vi "Main-final-V1.vi"() -> ()   [LabVIEW 2016]
uses:
  <vilib>/Platform/TimedLoop/XDataNode/timing_clust.ctl
  <vilib>/Platform/TimedLoop/XDataNode/nitl_modes.ctl
  <vilib>/Platform/TimedLoop/XDataNode/wakeup.ctl
  <vilib>/Modbus/subvis/Modbus API/Modbus API.lvclass/Modbus API.ctl
  <vilib>/Modbus/subvis/Transmission Data Unit (ADU)/Transmission Data Unit/Transmission Data Unit.lvclass/Transmission Data Unit.ctl
  <vilib>/Modbus/master/Data Access/Unit ID/Set Unit ID Property.vi
  <vilib>/Modbus/subvis/Transmission Data Unit (ADU)/Transmission Data Unit/Data Access/Unit ID/Write Unit ID.vi
  <vilib>/Modbus/subvis/Modbus API/Read Transmission Data Unit.vi
  <vilib>/Modbus/subvis/Modbus API/Write Transmission Data Unit.vi
  <vilib>/Modbus/master/Modbus Master.lvclass
  C:/Program Files (x86)/National Instruments/LabVIEW 2016/vi.lib/Modbus/subvis/Modbus API/Modbus API.lvclass
  <vilib>/Instr/_visa.llb/VISA Configure Serial Port (Instr).vi
  <vilib>/Modbus/master/Create Master Instance (TCP).vi
  <vilib>/httpClient/POSTBuffer.vi
  <vilib>/Modbus/subvis/Transmission Data Unit (ADU)/Transmission Data Unit/Transmission Data Unit.lvclass
  <vilib>/platform/TimedLoop/XDataNode/XDataNode.xnode
  <vilib>/httpClient/LabVIEWHTTPClient.lvlib
  <vilib>/Platform/TimedLoop/XDataNode/XDNodeRunTimeDep.lvlib
panel:
  out "logical OR 2":bool
  out "logical OR":bool
  out "x .or. y? 2":bool
  out "x .or. y?":bool
  in  "Tab Control 2":T1(tab)
  in  "Tab Control 4":enum32{"INVERTER 1", "INVERTER 2", "INVERTER 3"}(tab)
  in  "Tab Control 5":enum32{"DATA", "PLOTS"}(tab)
  out "AC-LOAD VOLTAGE":dbl
  out "AC-LOAD-CURRENT":dbl
  out "AC-LOAD-POWER":dbl
  out "AC-GRID-VOLTAGE":dbl
  out "AC-GRID-CURRENT":dbl
  out "AC-GRID-POWER":i32
  out "DC VOLT":dbl
  out "DC-CURRENT":dbl
  out "INVERT-DC-POWER":u32
  out "DC-POWER":dbl
  out "INVERT-DC-CURRENT":dbl
  out "CHARGE-DC-CURRENT":dbl
  out "CHARGE-DC-POWER":u32
  out "DC Power":cluster{dbl[], dbl[]}[](graph)
  out "DC Current":cluster{dbl[], dbl[]}[](graph)
  out "AC Power 1":cluster{dbl[], dbl[]}[](graph)
  out "AC Current 1":cluster{dbl[], dbl[]}[](graph)
  out "AC Voltage 1":cluster{dbl[], dbl[]}[](graph)
  in  "Tab Control 6":enum32{"DATA", "PLOTS"}(tab)
  out "AC-GRID-POWER 2":i32
  out "AC-GRID-CURRENT 2":dbl
  out "AC-GRID-VOLTAGE 2":dbl
  out "AC-LOAD-POWER 2":dbl
  out "AC-LOAD-CURRENT 2":dbl
  out "AC-LOAD VOLTAGE 2":dbl
  out "CHARGE-DC-POWER 2":u32
  out "CHARGE-DC-CURRENT 2":dbl
  out "INVERT-DC-CURRENT 2":dbl
  out "DC-POWER 2":dbl
  out "INVERT-DC-POWER 2":u32
  out "DC-CURRENT 2":dbl
  out "DC VOLT 2":dbl
  out "AC Voltage 2":cluster{dbl[], dbl[]}[](graph)
  out "AC Current 2":cluster{dbl[], dbl[]}[](graph)
  out "AC Power 2":cluster{dbl[], dbl[]}[](graph)
  out "DC Current 2":cluster{dbl[], dbl[]}[](graph)
  out "DC Power 2":cluster{dbl[], dbl[]}[](graph)
  in  "Tab Control 7":enum32{"DATA", "PLOTS"}(tab)
  out "CHARGE-DC-POWER 3":u32
  out "CHARGE-DC-CURRENT 3":dbl
  out "INVERT-DC-CURRENT 3":dbl
  out "DC-POWER 3":dbl
  out "INVERT-DC-POWER 3":u32
  out "DC-CURRENT 3":dbl
  out "DC VOLT 3":dbl
  out "AC-GRID-POWER 3":i32
  out "AC-GRID-CURRENT 3":dbl
  out "AC-GRID-VOLTAGE 3":dbl
  out "AC-LOAD-POWER 3":dbl
  out "AC-LOAD-CURRENT 3":dbl
  out "AC-LOAD VOLTAGE 3":dbl
  out "DC Power 3":cluster{dbl[], dbl[]}[](graph)
  out "DC Current 3":cluster{dbl[], dbl[]}[](graph)
  out "AC Power 3":cluster{dbl[], dbl[]}[](graph)
  out "AC Current 3":cluster{dbl[], dbl[]}[](graph)
  out "AC Voltage 3":cluster{dbl[], dbl[]}[](graph)
  in  "Tab Control 8":T2(tab)
  in  "Tab Control 9":enum32{"DATA", "PLOTS"}(tab)
  out "BATT FCAP-1":dbl(slide) scale=0.0..10.0
  out "BATT-CAP-1":dbl(slide) scale=0.0..100.0
  out "BATT-AVAIL-ENERGY-1":dbl(knob) scale=0.0..5200.0
  out "BATT-ENERGY-1":dbl(knob) scale=0.0..5200.0
  out "POWER-1":dbl(knob) scale=0.0..9000.0
  out "BATT-1 CURRENT":dbl(slide) scale=0.0..150.0
  out "batt-1 volt":u8(slide) scale=0.0..59.0
  out "BATTERY VOLTAGE 1":dbl
  out "BATTERY CURRENT":dbl
  out "BATTERY POWER":dbl
  out "BATTERY MAX ENERGY":dbl
  out "BATTERY AVAIL ENERGY":dbl
  out "BATTERY REM CAPACITY":dbl
  out "BATTERY FULL CAPACITY":dbl
  out "BATT-TEMP":dbl
  out "Batt-temp-1":dbl(slide) scale=0.0..100.0
  in  "Tab Control 11":enum32{"DATA", "PLOTS"}(tab)
  out "BATT FCAP-2":dbl(slide) scale=0.0..10.0
  out "BATT-CAP-2":dbl(slide) scale=0.0..100.0
  out "BATT-AVAIL-ENERGY-2":dbl(knob) scale=0.0..5200.0
  out "BATT-ENERGY-2":dbl(knob) scale=0.0..5200.0
  out "POWER-2":dbl(knob) scale=0.0..9000.0
  out "BATT-2 CURRENT":dbl(slide) scale=0.0..150.0
  out "batt-2 volt":u8(slide) scale=0.0..59.0
  out "BATTERY VOLTAGE 2":dbl
  out "BATTERY CURRENT 2":dbl
  out "BATTERY POWER 2":dbl
  out "BATTERY MAX ENERGY 2":dbl
  out "BATTERY AVAIL ENERGY 2":dbl
  out "BATTERY REM CAPACITY 2":dbl
  out "BATTERY FULL CAPACITY 2":dbl
  out "BATT-TEMP 2":dbl
  out "Batt-temp-2":dbl(slide) scale=0.0..100.0
  in  "Tab Control 12":enum32{"DATA", "PLOTS"}(tab)
  out "BATT FCAP-3":dbl(slide) scale=0.0..10.0
  out "BATT-CAP-3":dbl(slide) scale=0.0..100.0
  out "BATT-AVAIL-ENERGY-3":dbl(knob) scale=0.0..5200.0
  out "BATT-ENERGY-3":dbl(knob) scale=0.0..5200.0
  out "POWER-3":dbl(knob) scale=0.0..9000.0
  out "BATT-3 CURRENT":dbl(slide) scale=0.0..150.0
  out "batt-3 volt":u8(slide) scale=0.0..59.0
  out "BATTERY VOLTAGE 3":dbl
  out "BATTERY CURRENT 3":dbl
  out "BATTERY POWER 3":dbl
  out "BATTERY MAX ENERGY 3":dbl
  out "BATTERY AVAIL ENERGY 3":dbl
  out "BATTERY REM CAPACITY 3":dbl
  out "BATTERY FULL CAPACITY 3":dbl
  out "BATT-TEMP 3":dbl
  out "Batt-temp-3":dbl(slide) scale=0.0..100.0
  in  "Tab Control 13":enum32{"DATA", "PLOTS"}(tab)
  out "BATT FCAP-4":dbl(slide) scale=0.0..10.0
  out "BATT-CAP-4":dbl(slide) scale=0.0..100.0
  out "BATT-AVAIL-ENERGY-4":dbl(knob) scale=0.0..5200.0
  out "BATT-ENERGY-4":dbl(knob) scale=0.0..5200.0
  out "POWER-4":dbl(knob) scale=0.0..9000.0
  out "BATT-4 CURRENT":dbl(slide) scale=0.0..150.0
  out "batt-4 volt":u8(slide) scale=0.0..59.0
  out "BATTERY VOLTAGE 4":dbl
  out "BATTERY CURRENT 4":dbl
  out "BATTERY POWER 4":dbl
  out "BATTERY MAX ENERGY 4":dbl
  out "BATTERY AVAIL ENERGY 4":dbl
  out "BATTERY REM CAPACITY 4":dbl
  out "BATTERY FULL CAPACITY 4":dbl
  out "BATT-TEMP 4":dbl
  out "Batt-temp-4":dbl(slide) scale=0.0..100.0
  in  "Tab Control 14":enum32{"DATA", "PLOTS"}(tab)
  out "BATT FCAP-5":dbl(slide) scale=0.0..10.0
  out "BATT-CAP-5":dbl(slide) scale=0.0..100.0
  out "BATT-AVAIL-ENERGY-5":dbl(knob) scale=0.0..5200.0
  out "BATT-ENERGY-5":dbl(knob) scale=0.0..5200.0
  out "POWER-5":dbl(knob) scale=0.0..9000.0
  out "BATT-5 CURRENT":dbl(slide) scale=0.0..150.0
  out "batt-5 volt":u8(slide) scale=0.0..59.0
  out "BATTERY VOLTAGE 5":dbl
  out "BATTERY CURRENT 5":dbl
  out "BATTERY POWER 5":dbl
  out "BATTERY MAX ENERGY 5":dbl
  out "BATTERY AVAIL ENERGY 5":dbl
  out "BATTERY REM CAPACITY 5":dbl
  out "BATTERY FULL CAPACITY 5":dbl
  out "BATT-TEMP 5":dbl
  out "Batt-temp-5":dbl(slide) scale=0.0..100.0
  in  "?":T3(tab)
  out "Battery Voltage Discharge Plot":cluster{dbl[], dbl[]}[](graph)
  out "Battery Current Plot":cluster{dbl[], dbl[]}[](graph)
  out "Battery Power Plot":cluster{dbl[], dbl[]}[](graph)
  in  "?":T4(tab)
  out "Battery Remaining Capacity Plot":cluster{dbl[], dbl[]}[](graph)
  out "Battery Available Energy Plot":cluster{dbl[], dbl[]}[](graph)
  out "Battery temp plot":cluster{dbl[], dbl[]}[](graph)
  in  "Tab Control 10":enum32{"DATA", "PLOTS"}(tab)
  in  "?":enum32{"Voltage", "TAP Voltage", "Temperature"}(tab)
  out "Vertical Progress Bar 6":u8(slide) scale=0.0..100.0
  out "Vertical Progress Bar 5":u8(slide) scale=0.0..100.0
  out "Vertical Progress Bar 4":u8(slide) scale=0.0..100.0
  out "Vertical Progress Bar 3":u8(slide) scale=0.0..100.0
  out "Vertical Progress Bar 2":u8(slide) scale=0.0..100.0
  out "Vertical Progress Bar":u8(slide) scale=0.0..100.0
  out "?":u8(slide) scale=0.0..100.0
  out "VOLT-CAP-6":dbl
  out "VOLT-CAP-5":dbl
  out "VOLT-CAP-4":dbl
  out "VOLT-CAP-3":dbl
  out "VOLT-CAP-2":dbl
  out "VOLT-CAP-1":dbl
  out "MOD 6":bool
  out "MOD 5":bool
  out "TAP 7":dbl(slide) scale=0.0..100.0
  out "TAP 8":dbl(slide) scale=0.0..100.0
  out "TAP 9":dbl(slide) scale=0.0..100.0
  out "TAP 10":dbl(slide) scale=0.0..100.0
  out "TAP 11":dbl(slide) scale=0.0..100.0
  out "TAP 12":dbl(slide) scale=0.0..100.0
  out "TAP 13":dbl(slide) scale=0.0..100.0
  out "TAP 14":dbl(slide) scale=0.0..100.0
  out "TAP 15":dbl(slide) scale=0.0..100.0
  out "TAP 16":dbl(slide) scale=0.0..100.0
  out "TAP 17":dbl(slide) scale=0.0..100.0
  out "TAP 18":dbl(slide) scale=0.0..100.0
  out "MOD 4":bool
  out "TAP 19":dbl(slide) scale=0.0..100.0
  out "TAP 20":dbl(slide) scale=0.0..100.0
  out "TAP 4_":dbl(slide) scale=0.0..100.0
  out "TAP 4_3":dbl(slide) scale=0.0..100.0
  out "TAP 4_2":dbl(slide) scale=0.0..100.0
  out "TAP 4_1":dbl(slide) scale=0.0..100.0
  out "MOD 3":bool
  out "MOD 2":bool
  out "MOD 1":bool
  out "TAP 3_3":dbl(slide) scale=0.0..12.0
  out "TAP 3_1":dbl(slide) scale=0.0..5.0
  out "TAP 3_2":dbl(slide) scale=0.0..8.0
  out "TAP 3_6":dbl(slide) scale=0.0..25.0
  out "TAP 3_4":dbl(slide) scale=0.0..16.0
  out "TAP 3_5":dbl(slide) scale=0.0..20.0
  out "TAP 2_6":dbl(slide) scale=0.0..25.0
  out "TAP 2_5":dbl(slide) scale=0.0..20.0
  out "TAP 2_4":dbl(slide) scale=0.0..16.0
  out "TAP 2_3":dbl(slide) scale=0.0..12.0
  out "TAP 2_2":dbl(slide) scale=0.0..8.0
  out "TAP 2_1":dbl(slide) scale=0.0..5.0
  out "TAP 1_5":dbl(slide) scale=0.0..20.0
  out "TAP 1_4":dbl(slide) scale=0.0..16.0
  out "TAP 1_6":dbl(slide) scale=0.0..25.0
  out "TAP 1_3":dbl(slide) scale=0.0..12.0
  out "TAP 1_2":dbl(slide) scale=0.0..8.0
  out "TAP 1_1":dbl(slide) scale=0.0..5.0
  out "Temp_1":dbl(slide) scale=0.0..100.0
  out "Temp_2":dbl(slide) scale=0.0..100.0
  out "Temp_3":dbl(slide) scale=0.0..100.0
  out "Temp_4":dbl(slide) scale=0.0..100.0
  out "Temp_5":dbl(slide) scale=0.0..100.0
  out "Temp_6":dbl(slide) scale=0.0..100.0
  in  "Tab Control":T5(tab)
  out "TAP Voltages":cluster{dbl[], dbl[]}[](graph)
  out "Full Voltage":cluster{dbl[], dbl[]}[](graph)
  out "Module's Voltages":cluster{dbl[], dbl[]}[](graph)
  in  "BATT-GATE 2":bool
  in  "BATT-GATE 1":bool
  in  "BATT-GATE 5":bool
  in  "BATT-GATE 3":bool
  in  "BATT-GATE 4":bool
  in  "SUPERCAP-GATE 6":bool
  in  "Load-1":bool
  in  "Load-2":bool
  out "Power Button State":dbl
  out "Power Switch Led":bool
  in  "Tab Control 3":T6(tab)
  in  "INVERTER IP: 192.168.0.151":string
  in  "error in (no error)":errorcluster
  out "error out":errorcluster
  out "error out 2":errorcluster
  out "error out 3":errorcluster
  in  "VISA resource name":refnum<visa-resource-name>
  in  "Continuous Measurement":bool
  out "Total Received":u32
  out "Counter Register":dbl
  in  "Stop RT":bool
  in  "?":bool
  in  "Transmit Frame":T7={"timestamp high"=0, "timestamp low"=0, "identifier"=18, "type"=enum."Data Frame", "info A"=0, "info B"=0, "data length"=8, "data"=[0, 0, 0, 0, 0, 0, 0, 0]} {"identifier" format="%x"; "data" format="%.0x"}
  in  "control battery url":string
  in  "Batter data send url":string
  # "https://aertcsmartgrid.onrender.com/receive-data"
  # "https://aertcsmartgrid.onrender.com/get-btcontrol"
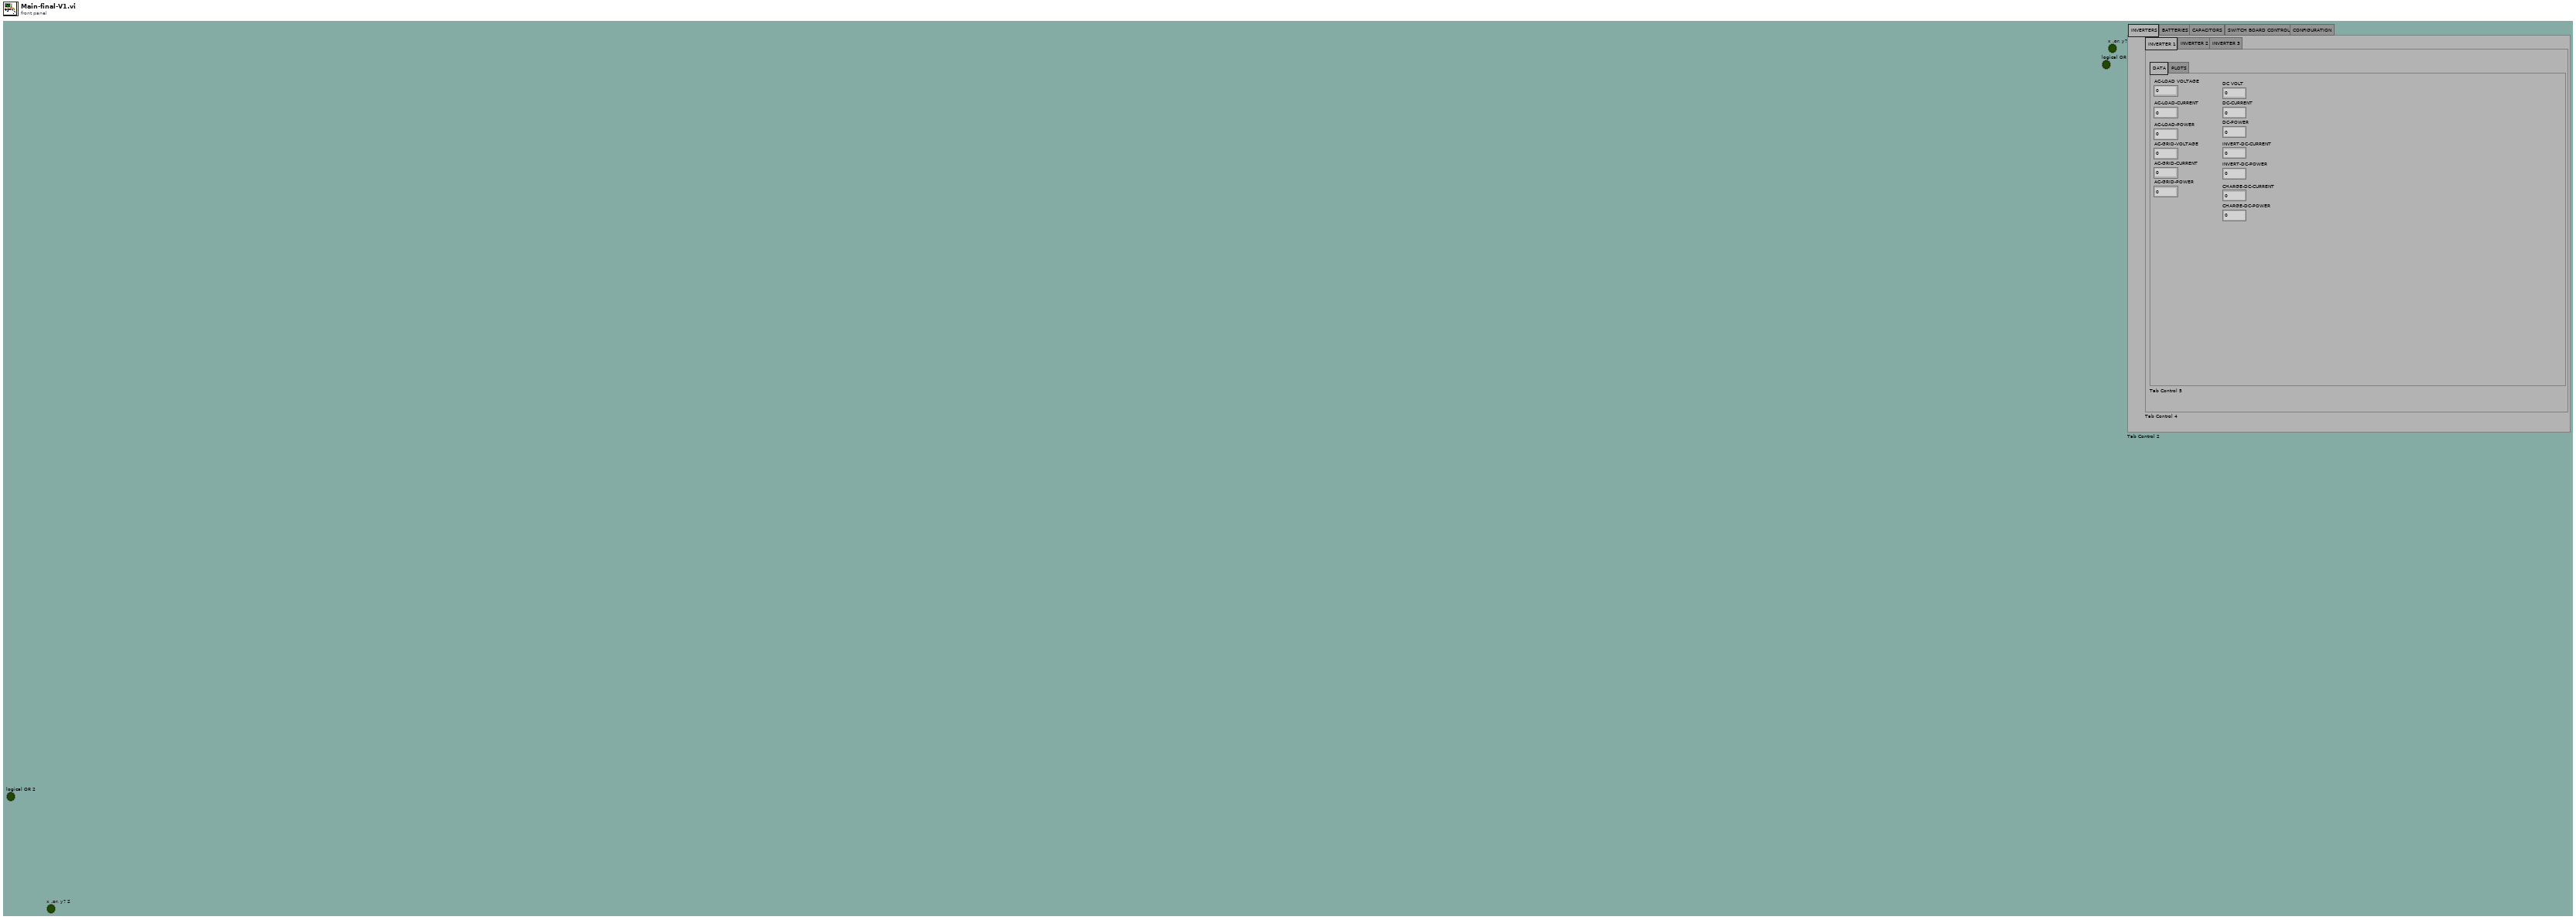
[diagram p1: front panel]
types:
  T1 = enum32{"INVERTERS", "BATTERIES", "CAPACITORS", "SWITCH BOARD CONTROL", "CONFIGURATION"}
  T2 = enum32{"BATTERY 1", "BATTERY 2", "BATTERY 3", "BATTERY 4", "BATTERY 5", "PLOTS"}
  T3 = enum32{"Voltage Plot", "Current Plot", "Power Plot"}
  T4 = enum32{"Remaining Capacity Plot", "Available Energy Plot", "Temperature Plot"}
  T5 = enum32{"TAP Plot", "FULL VOLTAGE PLOT", "FULL VOLTAGE PLOT 2"}
  T6 = enum32{"INVERTERS CONFIGURATION", "BATTERIES CONFIGURATION", "CAPACITORS CONFIGURATION", "WEBSITE CONFIGURATION"}
  T7 = cluster{"timestamp high":u32, "timestamp low":u32, "identifier":u32, "type":enum8{"Data Frame", "Remote Frame", "(reserved)", "(reserved) ", "(reserved)  ", "(reserved)   ", "Bus Error", "Transceiver Fault"}, "info A":u8, "info B":u8, "data length":u8, "data":u8[]}
  T8 = typedef "XDNodeRunTimeDep.lvlib/timing_clust.ctl" = cluster{"Expected End [f-1]":u64, "Actual End [f-1]":u64, "Finished Late? [f-1]":bool, "Expected End [i-1]":u64, "Actual End [i-1]":u64, "Finished Late? [i-1]":bool, "Expected Start [i]":u64, "Actual Start [i]":u64, "Expected Start [f]":u64, "Actual Start [f]":u64, "Source Name":string, "Structure Name":string, "Period":i64, "Deadline":i64, "Offset":i64, "Start":i64, "Priority":i32, "Timeout":i32, "Mode":T9, "Wakeup Reason":T10, "Error":errorcluster, "Source Type":string, "Secondary Source Type":string, "Global End Time":u64, "Global Start Time":u64, "Frame Duration":u64, "Iteration Duration":u64, "Assigned CPU":i32, "I/O Scan Engine Mode":u32}
  T9 = typedef "XDNodeRunTimeDep.lvlib/nitl_modes.ctl" = enum32{"No Change", "Process missed periods, maintain original phase", "Discard missed periods, maintain original phase", "Process missed periods, ignore original phase", "Discard missed periods, ignore original phase"}
  T10 = typedef "XDNodeRunTimeDep.lvlib/wakeup.ctl" = enum32{"Normal", "Aborted", "Asynchronous wakeup", "Timing source error", "Timed loop error", "Timeout"}
  T11 = typedef "LabVIEWHTTPClient.lvlib/ClientHandle.ctl" = refnum<k1>
  T12 = cluster{"unsigned byte array[0]":u8, "unsigned byte array[1]":u8, "unsigned byte array[2]":u8, "unsigned byte array[3]":u8, "unsigned byte array[4]":u8, "unsigned byte array[5]":u8, "unsigned byte array[6]":u8, "unsigned byte array[7]":u8, "unsigned byte array[8]":u8}
  T13 = cluster{"data[0]":u8, "data[1]":u8, "data[2]":u8, "data[3]":u8, "data[4]":u8, "data[5]":u8, "data[6]":u8, "data[7]":u8, "data[8]":u8}
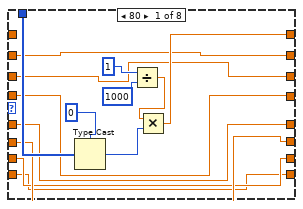
[diagram p3: hidden frame]
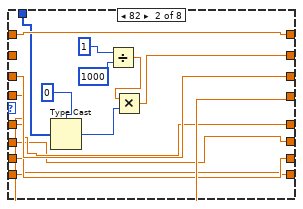
[diagram p4: hidden frame]
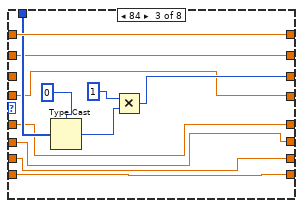
[diagram p5: hidden frame]
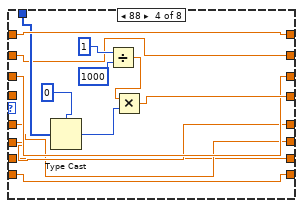
[diagram p6: hidden frame]
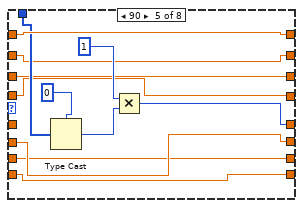
[diagram p7: hidden frame]
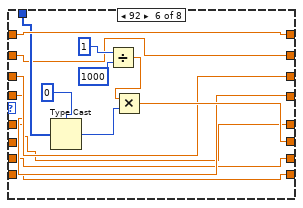
[diagram p8: hidden frame]
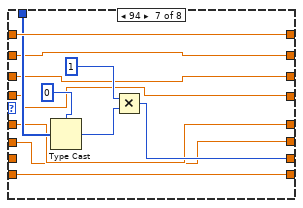
[diagram p9: hidden frame]
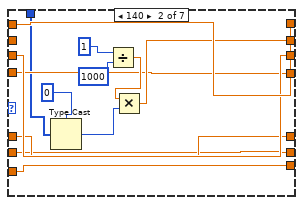
[diagram p10: hidden frame]
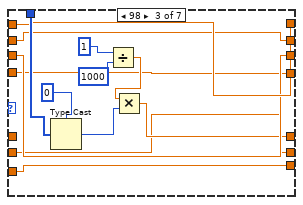
[diagram p11: hidden frame]
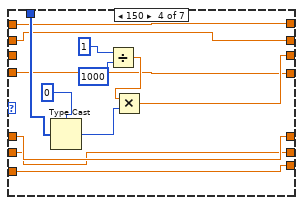
[diagram p12: hidden frame]
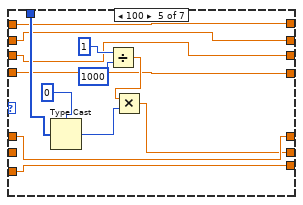
[diagram p13: hidden frame]
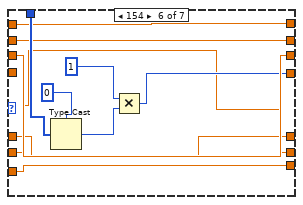
[diagram p14: hidden frame]
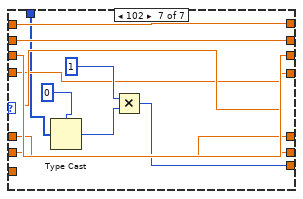
[diagram p15: hidden frame]
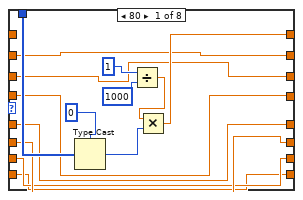
[diagram p16: hidden frame]
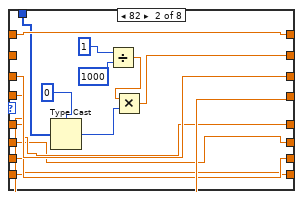
[diagram p17: hidden frame]
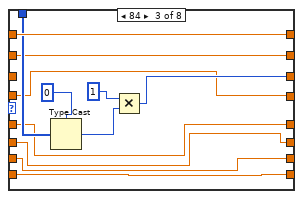
[diagram p18: hidden frame]
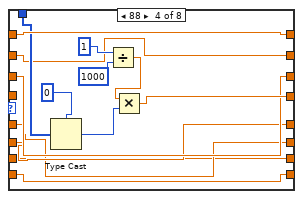
[diagram p19: hidden frame]
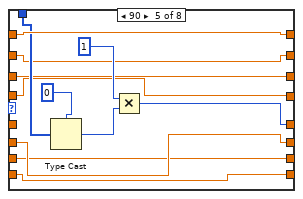
[diagram p20: hidden frame]
diagram:
  n1 = flat-sequence {
    tunnel: [w12] -> w6
    tunnel: [w11] -> w5
    tunnel: [w10] -> w4
    tunnel: [w9] -> w3
    tunnel: [w8] -> w2
    tunnel: [w7] -> w1
    tunnel: w6 -> [w137]
    tunnel: w5 -> [w136]
    tunnel: w4 -> [w125]
    tunnel: w3 -> [w124]
    tunnel: w2 -> [w123]
    tunnel: w1 -> [w122]
    frame #0 {
      n2 = call-poly "VISA Configure Serial Port"("VISA resource name"="VISA resource name", "timeout (10sec)"=u32 100000, "baud rate (9600)"=u32 115200) -> ("VISA resource name out"=w12:refnum<visa-resource-name>, "error out"=w11:errorcluster)  [unwired: 11 in]
      n3 = call <vilib>:"OpenHandle.vi"() -> ("client handle out"=w10:T11, "error out"=w9:errorcluster)  [unwired: 14 in]
      n4 = call <vilib>:"OpenHandle.vi"() -> ("client handle out"=w8:T11, "error out"=w7:errorcluster)  [unwired: 14 in]
    }
    frame #1 {
      w27 = 0.0
      w38 = 0.0
      w62 = 0.0
      w51 = 0.0
      w63 = 0.0
      w74 = 0.0
      w134 = 0.0
      w116 = 0.0
      w131 = 0.0
      w132 = 0.0
      w130 = 0.0
      w133 = 0.0
      w135 = 0.0
      w165 = 0.0
      # "M4"
      # "M3"
      # "M2"
      # "M1"
      n5 = disable-structure shown="Disabled" {
        frame Disabled {
          w171 = 0.005 ("y")
          w231 = 0.005 ("y")
          w244 = 0.005 ("y")
          n6 = Subtract() -> (y=w243:dbl, x-y=w253:dbl)  [unwired: 1 in]
          n7 = Subtract() -> (y=w242:dbl, x-y=w251:dbl)  [unwired: 1 in]
          n8 = Subtract() -> (x-y=w249:dbl)  [unwired: 2 in]
          n9 = Subtract() -> (x-y=w247:dbl)  [unwired: 2 in]
          n10 = Subtract() -> (x-y=w245:dbl)  [unwired: 2 in]
          n11 = Subtract(x=0.0, y=0.0) -> (x-y=w202:dbl)
          n12 = Subtract(x=0.0, y=0.0) -> (x-y=w186:dbl)
          n13 = Subtract(x=0.0, y=0.0) -> (x-y=w200:dbl)
          n14 = Subtract(x=0.0, y=0.0) -> (x-y=w198:dbl)
          n15 = Subtract(x=0.0, y=0.0) -> (x-y=w196:dbl)
          n16 = Subtract(x=0.0, y=0.0) -> (x-y=w194:dbl)
          n17 = Subtract(x=0.0, y=0.0) -> (x-y=w234:dbl)
          n18 = Subtract(x=0.0, y=0.0) -> (x-y=w232:dbl)
          n19 = Absolute Value(x=w253) -> (abs(x)=w254:dbl)
          n20 = Absolute Value(x=w251) -> (abs(x)=w252:dbl)
          n21 = Absolute Value(x=w249) -> (abs(x)=w250:dbl)
          n22 = Absolute Value(x=w247) -> (abs(x)=w248:dbl)
          n23 = Absolute Value(x=w245) -> (abs(x)=w246:dbl)
          n24 = Absolute Value(x=w202) -> (abs(x)=w203:dbl)
          n25 = Absolute Value(x=w186) -> (abs(x)=w187:dbl)
          n26 = Absolute Value(x=w200) -> (abs(x)=w201:dbl)
          n27 = Absolute Value(x=w198) -> (abs(x)=w199:dbl)
          n28 = Absolute Value(x=w196) -> (abs(x)=w197:dbl)
          n29 = Absolute Value(x=w194) -> (abs(x)=w195:dbl)
          n30 = Absolute Value(x=w234) -> (abs(x)=w235:dbl)
          n31 = Absolute Value(x=w232) -> (abs(x)=w233:dbl)
          n32 = Greater?(x=w254, y=w244) -> (0:w241:bool)
          n33 = Greater?(x=w252, y=w244) -> (0:w240:bool)
          n34 = Greater?(x=w250, y=w244) -> (0:w239:bool)
          n35 = Greater?(x=w248, y=w244) -> (0:w238:bool)
          n36 = Greater?(x=w246, y=w244) -> (0:w237:bool)
          n37 = call "BATT-ABSOLUTE-Second.vi"("B2"=0.0 ("y"), "Comp"=0.005 ("y"), "B1"=0.0 ("x"), "A2"=0.0 ("y"), "A1"=0.0 ("x")) -> ("Boolean"=→"x .or. y? 2":bool)  [unwired: 6 in]
          n38 = call "BATT-ABSOLUTE-Six.vi"("B2"=0.0 ("y"), "A6"=0.0 ("x"), "A3"=0.0 ("x"), "B6"=0.0 ("y"), "B3"=0.0 ("y"), "Comp"=0.005 ("y"), "A4"=0.0 ("x"), "B1"=0.0 ("y"), "B4"=0.0 ("y"), "A2"=0.0 ("x"), "A5"=0.0 ("x"), "A1"=0.0 ("x"), "B5"=0.0 ("y")) -> ("Boolean"=→"logical OR":bool)  [unwired: 6 in]
          n39 = Greater?(x=w203, y=w171) -> (0:w193:bool)
          n40 = Greater?(x=w187, y=w171) -> (0:w185:bool)
          n41 = Greater?(x=w201, y=w171) -> (0:w192:bool)
          n42 = Greater?(x=w199, y=w171) -> (0:w191:bool)
          n43 = Greater?(x=w197, y=w171) -> (0:w190:bool)
          n44 = Greater?(x=w195, y=w171) -> (0:w189:bool)
          n45 = Greater?(x=w235, y=w231) -> (0:w230:bool)
          n46 = Greater?(x=w233, y=w231) -> (0:w229:bool)
          n47 = Build Array(w241, w240, w239, w238, w237) -> (w236:bool[])
          n48 = Or(x=w230, y=w229) -> (x .or. y?=→"x .or. y?":bool)
          n49 = Build Array(w185, w193, w192, w191, w190, w189) -> (w188:bool[])
          n50 = Or Array Elements(Boolean array=w236) -> ()  [unwired: 1 out]
          n51 = Or Array Elements(Boolean array=w188) -> (logical OR=→"logical OR 2":bool)
        }
        frame Enabled {
        }
      }
      n52 = call-poly <vilib>:"Create Master Instance.vi"("error in (no error)"="error in (no error)", "port (502)"=u16 503, "address"="INVERTER IP: 192.168.0.151") -> ("error out"=w85:errorcluster, "TCP master instance"=w88:refnum<class "Modbus Master.lvclass">)  [unwired: 7 in]
      n53 = while {
        shift-right: [w595] -> w87
        shift-left: w88 -> [w504]
        shift-right: [w594] -> w84
        shift-left: w85 -> [w503]
        shift-right: [w587] -> _
        shift-left: w74 -> [w588]
        shift-right: [w494] -> _
        shift-left: w74 -> [w495]
        shift-right: [w490] -> _
        shift-left: w74 -> [w491]
        shift-right: [w486] -> _
        shift-left: w74 -> [w487]
        shift-right: [w397] -> _
        shift-left: dbl[] [] -> [w586]
        shift-right: [w395] -> _
        shift-left: dbl[] [] -> [w585]
        shift-right: [w393] -> _
        shift-left: dbl[] [] -> [w584]
        shift-right: [w492] -> _
        shift-left: w74 -> [w493]
        shift-right: [w488] -> _
        shift-left: w74 -> [w489]
        shift-right: [w484] -> _
        shift-left: w74 -> [w485]
        shift-right: [w391] -> _
        shift-left: dbl[] [] -> [w581]
        shift-right: [w389] -> _
        shift-left: dbl[] [] -> [w582]
        shift-right: [w387] -> _
        shift-left: dbl[] [] -> [w583]
        shift-right: [w429] -> _
        shift-left: dbl[] [] -> [w574]
        shift-right: [w428] -> _
        shift-left: dbl[] [] -> [w575]
        shift-right: [w427] -> _
        shift-left: dbl[] [] -> [w576]
        shift-right: [w369] -> _
        shift-left: dbl[] [] -> [w577]
        shift-right: [w367] -> _
        shift-left: dbl[] [] -> [w578]
        shift-right: [w365] -> _
        shift-left: dbl[] [] -> [w580]
        shift-right: [w363] -> _
        shift-left: dbl[] [] -> [w579]
        shift-right: [w573] -> _
        shift-left: w63 -> [w572]
        shift-right: [w568] -> _
        shift-left: w63 -> [w570]
        shift-right: [w567] -> _
        shift-left: w63 -> [w569]
        shift-right: [w450] -> _
        shift-left: w63 -> [w453]
        shift-right: [w449] -> _
        shift-left: w63 -> [w446]
        shift-right: [w448] -> _
        shift-left: w63 -> [w452]
        shift-right: [w447] -> _
        shift-left: w63 -> [w565]
        shift-right: [w566] -> _
        shift-left: w63 -> [w451]
        shift-right: [w536] -> w45
        shift-left: _ -> [_]
        shift-right: [w537] -> w46
        shift-left: _ -> [_]
        shift-right: [w542] -> _
        shift-left: w51 -> [w541]
        shift-right: [w482] -> _
        shift-left: w51 -> [w483]
        shift-right: [w478] -> _
        shift-left: w51 -> [w479]
        shift-right: [w474] -> _
        shift-left: w51 -> [w475]
        shift-right: [w339] -> _
        shift-left: dbl[] [] -> [w543]
        shift-right: [w337] -> _
        shift-left: dbl[] [] -> [w544]
        shift-right: [w335] -> _
        shift-left: dbl[] [] -> [w545]
        shift-right: [w480] -> _
        shift-left: w51 -> [w481]
        shift-right: [w476] -> _
        shift-left: w51 -> [w477]
        shift-right: [w472] -> _
        shift-left: w51 -> [w473]
        shift-right: [w329] -> _
        shift-left: dbl[] [] -> [w548]
        shift-right: [w331] -> _
        shift-left: dbl[] [] -> [w547]
        shift-right: [w333] -> _
        shift-left: dbl[] [] -> [w546]
        shift-right: [w424] -> _
        shift-left: dbl[] [] -> [w555]
        shift-right: [w423] -> _
        shift-left: dbl[] [] -> [w554]
        shift-right: [w422] -> _
        shift-left: dbl[] [] -> [w553]
        shift-right: [w313] -> _
        shift-left: dbl[] [] -> [w552]
        shift-right: [w311] -> _
        shift-left: dbl[] [] -> [w551]
        shift-right: [w309] -> _
        shift-left: dbl[] [] -> [w549]
        shift-right: [w307] -> _
        shift-left: dbl[] [] -> [w550]
        shift-right: [w556] -> _
        shift-left: w62 -> [w557]
        shift-right: [w561] -> _
        shift-left: w62 -> [w559]
        shift-right: [w562] -> _
        shift-left: w62 -> [w560]
        shift-right: [w441] -> _
        shift-left: w62 -> [w445]
        shift-right: [w440] -> _
        shift-left: w62 -> [w444]
        shift-right: [w439] -> _
        shift-left: w62 -> [w443]
        shift-right: [w438] -> _
        shift-left: w62 -> [w442]
        shift-right: [w563] -> _
        shift-left: w62 -> [w564]
        shift-right: [w533] -> w44
        shift-left: _ -> [_]
        shift-right: [w532] -> w43
        shift-left: _ -> [_]
        shift-right: [w527] -> _
        shift-left: w38 -> [w528]
        shift-right: [w465] -> _
        shift-left: w38 -> [w471]
        shift-right: [w464] -> _
        shift-left: w38 -> [w470]
        shift-right: [w463] -> _
        shift-left: w38 -> [w469]
        shift-right: [w287] -> _
        shift-left: dbl[] [] -> [w526]
        shift-right: [w285] -> _
        shift-left: dbl[] [] -> [w525]
        shift-right: [w283] -> _
        shift-left: dbl[] [] -> [w524]
        shift-right: [w462] -> _
        shift-left: w38 -> [w468]
        shift-right: [w461] -> _
        shift-left: w38 -> [w467]
        shift-right: [w460] -> _
        shift-left: w38 -> [w466]
        shift-right: [w281] -> _
        shift-left: dbl[] [] -> [w521]
        shift-right: [w279] -> _
        shift-left: dbl[] [] -> [w522]
        shift-right: [w277] -> _
        shift-left: dbl[] [] -> [w523]
        shift-right: [w419] -> _
        shift-left: dbl[] [] -> [w514]
        shift-right: [w418] -> _
        shift-left: dbl[] [] -> [w515]
        shift-right: [w417] -> _
        shift-left: dbl[] [] -> [w516]
        shift-right: [w261] -> _
        shift-left: dbl[] [] -> [w517]
        shift-right: [w259] -> _
        shift-left: dbl[] [] -> [w518]
        shift-right: [w257] -> _
        shift-left: dbl[] [] -> [w520]
        shift-right: [w255] -> _
        shift-left: dbl[] [] -> [w519]
        shift-right: [w513] -> _
        shift-left: w27 -> [w512]
        shift-right: [w508] -> _
        shift-left: w27 -> [w510]
        shift-right: [w507] -> _
        shift-left: w27 -> [w509]
        shift-right: [w433] -> _
        shift-left: w27 -> [w437]
        shift-right: [w432] -> _
        shift-left: w27 -> [w436]
        shift-right: [w431] -> _
        shift-left: w27 -> [w435]
        shift-right: [w430] -> _
        shift-left: w27 -> [w434]
        shift-right: [w506] -> _
        shift-left: w27 -> [w505]
        shift-right: [w399] -> _
        shift-left: dbl[] [] -> [w409]
        shift-right: [w371] -> _
        shift-left: dbl[] [] -> [w380]
        shift-right: [w341] -> _
        shift-left: dbl[] [] -> [w352]
        shift-right: [w315] -> _
        shift-left: dbl[] [] -> [w328]
        shift-right: [w289] -> _
        shift-left: dbl[] [] -> [w306]
        shift-right: [w263] -> _
        shift-left: dbl[] [] -> [w276]
        stop <- FALSE stop-if-true
        n54 = call "UP-COUNTER-V1.vi"("UPPER LIMIT"=17.0) -> ("COUNT"=w589:dbl)  [unwired: 10 in]
        n55 = case shown="1, Default" w589 {
          tunnel: [u32 86 u32 140 u32 98 u32 150 u32 100 u32 154 u32 102 u32 80 u32 82 u32 84 u32 88 u32 90 u32 92 u32 94 u32 96] -> w502
          frame 1, Default {
            # "TEMP-BATT"
          }
          frame 2 {
            # "AC-LOAD-VOLT"
          }
          frame 3 {
            # "AC-GRID-VOLT"
          }
          frame 4 {
            # "AC-LOAD-CURRENT"
          }
          frame 5 {
            # "AC-GRID-CURRENT"
          }
          frame 6 {
            # "AC-LOAD-POWER"
          }
          frame 7 {
            # "AC-GRID-POWER"
          }
          frame 8 {
            # "DC-VOLT"
          }
          frame 9 {
            # "DC-CURRENT"
          }
          frame 10 {
            # "DC-POWER"
          }
          frame 11 {
            # "INVERT-DC-CURRENT"
          }
          frame 12 {
            # "INVERT-DC-POWER"
          }
          frame 13 {
            # "CHARGE-DC-CURRENT"
          }
          frame 14 {
            # "CHARGE-DC-POWER"
          }
          frame 15 {
            # "CHARGE-%"
          }
        }
        n56 = property class="Modbus Master"(reference=w504, error in=w503, "Data Access:Unit ID"=u8 12 ("Unit ID")) -> (reference out=w529:refnum<class "Modbus Master.lvclass">, error out=w530:errorcluster)
        n57 = property class="Modbus Master"(reference=w504, error in=w503, "Data Access:Unit ID"=u8 10 ("Unit ID")) -> (reference out=w590:refnum<class "Modbus Master.lvclass">, error out=w591:errorcluster)
        n58 = property class="Modbus Master"(reference=w504, error in=w503, "Data Access:Unit ID"=u8 11 ("Unit ID")) -> (reference out=w540:refnum<class "Modbus Master.lvclass">, error out=w539:errorcluster)
        n59 = call-dynamic "Read Holding Registers.vi"("error in (no error)"=w530, "number of holding registers"=u32 2, "starting address"=w502, "Modbus master in"=w529) -> ("error out"=w532:errorcluster, "register values"=w511:u16[], "Modbus master out"=w533:refnum<class "Modbus Master.lvclass">)  [unwired: 5 in]
        n60 = call-dynamic "Read Holding Registers.vi"("error in (no error)"=w591, "number of holding registers"=u32 2, "starting address"=w502, "Modbus master in"=w590) -> ("error out"=w594:errorcluster, "register values"=w571:u16[], "Modbus master out"=w595:refnum<class "Modbus Master.lvclass">)  [unwired: 5 in]
        n61 = call-dynamic "Read Holding Registers.vi"("error in (no error)"=w539, "number of holding registers"=u32 2, "starting address"=w502, "Modbus master in"=w540) -> ("error out"=w537:errorcluster, "register values"=w558:u16[], "Modbus master out"=w536:refnum<class "Modbus Master.lvclass">)  [unwired: 5 in]
        n62 = case shown="86, Default" w502 {
          tunnel: w511 -> [w701 w716 w736 w749 w762 w776 w779]
          tunnel: [w710 w723 w735 w748 w761 w775 w787] -> w527
          tunnel: w528 -> [_ w723 w735 w748 w761 w775 w787]
          tunnel: [w707 w722 w731 w747 w760 w774 w786] -> w465
          tunnel: w471 -> [w707 _ w731 w747 w760 w774 w786]
          tunnel: [w706 w721 w734 w746 w757 w773 w785] -> w464
          tunnel: w470 -> [w706 w721 w734 _ w757 w773 w785]
          tunnel: [w705 w720 w733 w745 w759 w772 w780] -> w463
          tunnel: w469 -> [w705 w720 w733 w745 w759 _ w780]
          tunnel: [w704 w719 w732 w744 w758 w770 w783] -> w462
          tunnel: w468 -> [w704 w719 _ w744 w758 w770 w783]
          tunnel: [w703 w718 w730 w743 w756 w769 w782] -> w461
          tunnel: w467 -> [w703 w718 w730 w743 _ w769 w782]
          tunnel: [w702 w717 w729 w742 w755 w768 w781] -> w460
          tunnel: w466 -> [w702 w717 w729 w742 w755 w768 _]
          frame 86, Default {
            n63 = Type Cast(type=u16 0, x=w701) -> (*(type *) &x=w709:u16)
            n64 = Divide(x=u32 1, y=u32 100) -> (x/y=w712:dbl)
            n65 = Multiply(x=w712, y=w709) -> (x*y=w711:dbl)
            n66 = Subtract(x=w711, y=273) -> (x-y=w710:dbl)
          }
          frame 140 {
            n67 = Type Cast(type=u32 0, x=w716) -> (*(type *) &x=w725:u32)
            n68 = Divide(x=u32 1, y=u32 1000) -> (x/y=w726:dbl)
            n69 = Multiply(x=w726, y=w725) -> (x*y=w722:dbl)
          }
          frame 98 {
            n70 = Type Cast(type=u32 0, x=w736) -> (*(type *) &x=w738:u32)
            n71 = Divide(x=u32 1, y=u32 1000) -> (x/y=w739:dbl)
            n72 = Multiply(x=w739, y=w738) -> (x*y=w732:dbl)
          }
          frame 150 {
            n73 = Type Cast(type=0, x=w749) -> (*(type *) &x=w751:i32)
            n74 = Divide(x=u32 1, y=u32 1000) -> (x/y=w752:dbl)
            n75 = Multiply(x=w752, y=w751) -> (x*y=w746:dbl)
          }
          frame 100 {
            n76 = Type Cast(type=0, x=w762) -> (*(type *) &x=w764:i32)
            n77 = Divide(x=u32 1, y=u32 1000) -> (x/y=w765:dbl)
            n78 = Multiply(x=w765, y=w764) -> (x*y=w756:dbl)
          }
          frame 154 {
            n79 = Type Cast(type=0, x=w776) -> (*(type *) &x=w778:i32)
            n80 = Multiply(x=1, y=w778) -> (x*y=w772:i32)
          }
          frame 102 {
            n81 = Type Cast(type=0, x=w779) -> (*(type *) &x=w789:i32)
            n82 = Multiply(x=1, y=w789) -> (x*y=w781:i32)
          }
        }
        "AC-LOAD VOLTAGE 3" <- w465
        "AC-LOAD-CURRENT 3" <- w464
        "AC-LOAD-POWER 3" <- w463
        "AC-GRID-VOLTAGE 3" <- w462
        "AC-GRID-CURRENT 3" <- w461
        "AC-GRID-POWER 3" <- w460
        n83 = case shown="98" w502 {
          tunnel: w571 -> [w1102 w1117 w1137 w1150 w1163 w1177 w1180]
          tunnel: [w1111 w1124 w1136 w1149 w1162 w1176 w1188] -> w587
          tunnel: w588 -> [_ w1124 w1136 w1149 w1162 w1176 w1188]
          tunnel: [w1108 w1123 w1132 w1148 w1161 w1175 w1187] -> w494
          tunnel: w495 -> [w1108 _ w1132 w1148 w1161 w1175 w1187]
          tunnel: [w1107 w1122 w1135 w1147 w1158 w1174 w1186] -> w490
          tunnel: w491 -> [w1107 w1122 w1135 _ w1158 w1174 w1186]
          tunnel: [w1106 w1121 w1134 w1146 w1160 w1173 w1181] -> w486
          tunnel: w487 -> [w1106 w1121 w1134 w1146 w1160 _ w1181]
          tunnel: [w1105 w1120 w1133 w1145 w1159 w1171 w1184] -> w492
          tunnel: w493 -> [w1105 w1120 _ w1145 w1159 w1171 w1184]
          tunnel: [w1104 w1119 w1131 w1144 w1157 w1170 w1183] -> w488
          tunnel: w489 -> [w1104 w1119 w1131 w1144 _ w1170 w1183]
          tunnel: [w1103 w1118 w1130 w1143 w1156 w1169 w1182] -> w484
          tunnel: w485 -> [w1103 w1118 w1130 w1143 w1156 w1169 _]
          frame 86, Default {
            n84 = Type Cast(type=u16 0, x=w1102) -> (*(type *) &x=w1110:u16)
            n85 = Divide(x=u32 1, y=u32 100) -> (x/y=w1113:dbl)
            n86 = Multiply(x=w1113, y=w1110) -> (x*y=w1112:dbl)
            n87 = Subtract(x=w1112, y=273) -> (x-y=w1111:dbl)
          }
          frame 140 {
            n88 = Type Cast(type=u32 0, x=w1117) -> (*(type *) &x=w1126:u32)
            n89 = Divide(x=u32 1, y=u32 1000) -> (x/y=w1127:dbl)
            n90 = Multiply(x=w1127, y=w1126) -> (x*y=w1123:dbl)
          }
          frame 98 {
            n91 = Type Cast(type=u32 0, x=w1137) -> (*(type *) &x=w1139:u32)
            n92 = Divide(x=u32 1, y=u32 1000) -> (x/y=w1140:dbl)
            n93 = Multiply(x=w1140, y=w1139) -> (x*y=w1133:dbl)
          }
          frame 150 {
            n94 = Type Cast(type=0, x=w1150) -> (*(type *) &x=w1152:i32)
            n95 = Divide(x=u32 1, y=u32 1000) -> (x/y=w1153:dbl)
            n96 = Multiply(x=w1153, y=w1152) -> (x*y=w1147:dbl)
          }
          frame 100 {
            n97 = Type Cast(type=0, x=w1163) -> (*(type *) &x=w1165:i32)
            n98 = Divide(x=u32 1, y=u32 1000) -> (x/y=w1166:dbl)
            n99 = Multiply(x=w1166, y=w1165) -> (x*y=w1157:dbl)
          }
          frame 154 {
            n100 = Type Cast(type=0, x=w1177) -> (*(type *) &x=w1179:i32)
            n101 = Multiply(x=1, y=w1179) -> (x*y=w1173:i32)
          }
          frame 102 {
            n102 = Type Cast(type=0, x=w1180) -> (*(type *) &x=w1190:i32)
            n103 = Multiply(x=1, y=w1190) -> (x*y=w1182:i32)
          }
        }
        "AC-LOAD VOLTAGE" <- w494
        "AC-LOAD-CURRENT" <- w490
        "AC-LOAD-POWER" <- w486
        "AC-GRID-VOLTAGE" <- w492
        "AC-GRID-CURRENT" <- w488
        "AC-GRID-POWER" <- w484
        n104 = case shown="86, Default" w502 {
          tunnel: w558 -> [w894 w909 w929 w942 w955 w969 w972]
          tunnel: [w903 w916 w928 w941 w954 w968 w980] -> w542
          tunnel: w541 -> [_ w916 w928 w941 w954 w968 w980]
          tunnel: [w900 w915 w924 w940 w953 w967 w979] -> w482
          tunnel: w483 -> [w900 _ w924 w940 w953 w967 w979]
          tunnel: [w899 w914 w927 w939 w950 w966 w978] -> w478
          tunnel: w479 -> [w899 w914 w927 _ w950 w966 w978]
          tunnel: [w898 w913 w926 w938 w952 w965 w973] -> w474
          tunnel: w475 -> [w898 w913 w926 w938 w952 _ w973]
          tunnel: [w897 w912 w925 w937 w951 w963 w976] -> w480
          tunnel: w481 -> [w897 w912 _ w937 w951 w963 w976]
          tunnel: [w896 w911 w923 w936 w949 w962 w975] -> w476
          tunnel: w477 -> [w896 w911 w923 w936 _ w962 w975]
          tunnel: [w895 w910 w922 w935 w948 w961 w974] -> w472
          tunnel: w473 -> [w895 w910 w922 w935 w948 w961 _]
          frame 86, Default {
            n105 = Type Cast(type=u16 0, x=w894) -> (*(type *) &x=w902:u16)
            n106 = Divide(x=u32 1, y=u32 100) -> (x/y=w905:dbl)
            n107 = Multiply(x=w905, y=w902) -> (x*y=w904:dbl)
            n108 = Subtract(x=w904, y=273) -> (x-y=w903:dbl)
          }
          frame 140 {
            n109 = Type Cast(type=u32 0, x=w909) -> (*(type *) &x=w918:u32)
            n110 = Divide(x=u32 1, y=u32 1000) -> (x/y=w919:dbl)
            n111 = Multiply(x=w919, y=w918) -> (x*y=w915:dbl)
          }
          frame 98 {
            n112 = Type Cast(type=u32 0, x=w929) -> (*(type *) &x=w931:u32)
            n113 = Divide(x=u32 1, y=u32 1000) -> (x/y=w932:dbl)
            n114 = Multiply(x=w932, y=w931) -> (x*y=w925:dbl)
          }
          frame 150 {
            n115 = Type Cast(type=0, x=w942) -> (*(type *) &x=w944:i32)
            n116 = Divide(x=u32 1, y=u32 1000) -> (x/y=w945:dbl)
            n117 = Multiply(x=w945, y=w944) -> (x*y=w939:dbl)
          }
          frame 100 {
            n118 = Type Cast(type=0, x=w955) -> (*(type *) &x=w957:i32)
            n119 = Divide(x=u32 1, y=u32 1000) -> (x/y=w958:dbl)
            n120 = Multiply(x=w958, y=w957) -> (x*y=w949:dbl)
          }
          frame 154 {
            n121 = Type Cast(type=0, x=w969) -> (*(type *) &x=w971:i32)
            n122 = Multiply(x=1, y=w971) -> (x*y=w965:i32)
          }
          frame 102 {
            n123 = Type Cast(type=0, x=w972) -> (*(type *) &x=w982:i32)
            n124 = Multiply(x=1, y=w982) -> (x*y=w974:i32)
          }
        }
        "AC-LOAD VOLTAGE 2" <- w482
        "AC-LOAD-CURRENT 2" <- w478
        "AC-LOAD-POWER 2" <- w474
        "AC-GRID-VOLTAGE 2" <- w480
        "AC-GRID-CURRENT 2" <- w476
        "AC-GRID-POWER 2" <- w472
        n125 = case shown="96, Default" w502 {
          tunnel: [w603 w619 w630 w642 w656 w668 w682 w694] -> w508
          tunnel: [w602 w616 w634 w641 w655 w667 w681 w693] -> w507
          tunnel: [w600 w614 w628 w640 w660 w665 w679 w691] -> w432
          tunnel: [w598 w612 w626 w638 w652 w664 w686 w689] -> w430
          tunnel: [w601 w615 w629 w645 w654 w666 w680 w692] -> w433
          tunnel: [w599 w613 w627 w639 w653 w671 w678 w690] -> w431
          tunnel: [w597 w611 w625 w637 w651 w663 w677 w697] -> w506
          tunnel: [w605 w618 w632 w644 w658 w670 w684 w696] -> w513
          tunnel: w512 -> [_ w618 w632 w644 w658 w670 w684 w696]
          tunnel: w511 -> [w604 w617 w631 w643 w657 w669 w683 w695]
          tunnel: w510 -> [w603 _ w630 w642 w656 w668 w682 w694]
          tunnel: w509 -> [w602 w616 _ w641 w655 w667 w681 w693]
          tunnel: w437 -> [w601 w615 w629 _ w654 w666 w680 w692]
          tunnel: w436 -> [w600 w614 w628 w640 _ w665 w679 w691]
          tunnel: w435 -> [w599 w613 w627 w639 w653 _ w678 w690]
          tunnel: w434 -> [w598 w612 w626 w638 w652 w664 _ w689]
          tunnel: w505 -> [w597 w611 w625 w637 w651 w663 w677 _]
          frame 80 {
            n126 = Type Cast(type=u32 0, x=w604) -> (*(type *) &x=w608:u32)
            n127 = Divide(x=u32 1, y=u32 1000) -> (x/y=w609:dbl)
            n128 = Multiply(x=w609, y=w608) -> (x*y=w605:dbl)
          }
          frame 82 {
            n129 = Type Cast(type=0, x=w617) -> (*(type *) &x=w621:i32)
            n130 = Divide(x=u32 1, y=u32 1000) -> (x/y=w622:dbl)
            n131 = Multiply(x=w622, y=w621) -> (x*y=w619:dbl)
          }
          frame 84 {
            n132 = Type Cast(type=0, x=w631) -> (*(type *) &x=w636:i32)
            n133 = Multiply(x=u32 1, y=w636) -> (x*y=w634:u32)
          }
          frame 88 {
            n134 = Type Cast(type=u32 0, x=w643) -> (*(type *) &x=w647:u32)
            n135 = Divide(x=u32 1, y=u32 1000) -> (x/y=w648:dbl)
            n136 = Multiply(x=w648, y=w647) -> (x*y=w645:dbl)
          }
          frame 90 {
            n137 = Type Cast(type=u32 0, x=w657) -> (*(type *) &x=w662:u32)
            n138 = Multiply(x=u32 1, y=w662) -> (x*y=w660:u32)
          }
          frame 92 {
            n139 = Type Cast(type=u32 0, x=w669) -> (*(type *) &x=w673:u32)
            n140 = Divide(x=u32 1, y=u32 1000) -> (x/y=w674:dbl)
            n141 = Multiply(x=w674, y=w673) -> (x*y=w671:dbl)
          }
          frame 94 {
            n142 = Type Cast(type=u32 0, x=w683) -> (*(type *) &x=w688:u32)
            n143 = Multiply(x=1, y=w688) -> (x*y=w686:u32)
          }
          frame 96, Default {
            n144 = Type Cast(type=u16 0, x=w695) -> (*(type *) &x=w700:u16)
            n145 = Multiply(x=1, y=w700) -> (x*y=w697:i32)
          }
        }
        "DC VOLT 3" <- w513
        "DC-CURRENT 3" <- w508
        "INVERT-DC-POWER 3" <- w432
        "DC-POWER 3" <- w507
        "INVERT-DC-CURRENT 3" <- w433
        "CHARGE-DC-CURRENT 3" <- w431
        "CHARGE-DC-POWER 3" <- w430
        n146 = case shown="96, Default" w502 {
          tunnel: [w989 w1005 w1016 w1028 w1042 w1054 w1068 w1080] -> w568
          tunnel: [w988 w1002 w1020 w1027 w1041 w1053 w1067 w1079] -> w567
          tunnel: [w986 w1000 w1014 w1026 w1046 w1051 w1065 w1077] -> w449
          tunnel: [w984 w998 w1012 w1024 w1038 w1050 w1072 w1075] -> w447
          tunnel: [w987 w1001 w1015 w1031 w1040 w1052 w1066 w1078] -> w450
          tunnel: [w985 w999 w1013 w1025 w1039 w1057 w1064 w1076] -> w448
          tunnel: [w983 w997 w1011 w1023 w1037 w1049 w1063 w1083] -> w566
          tunnel: [w991 w1004 w1018 w1030 w1044 w1056 w1070 w1082] -> w573
          tunnel: w572 -> [_ w1004 w1018 w1030 w1044 w1056 w1070 w1082]
          tunnel: w571 -> [w990 w1003 w1017 w1029 w1043 w1055 w1069 w1081]
          tunnel: w570 -> [w989 _ w1016 w1028 w1042 w1054 w1068 w1080]
          tunnel: w569 -> [w988 w1002 _ w1027 w1041 w1053 w1067 w1079]
          tunnel: w453 -> [w987 w1001 w1015 _ w1040 w1052 w1066 w1078]
          tunnel: w446 -> [w986 w1000 w1014 w1026 _ w1051 w1065 w1077]
          tunnel: w452 -> [w985 w999 w1013 w1025 w1039 _ w1064 w1076]
          tunnel: w565 -> [w984 w998 w1012 w1024 w1038 w1050 _ w1075]
          tunnel: w451 -> [w983 w997 w1011 w1023 w1037 w1049 w1063 _]
          frame 80 {
            n147 = Type Cast(type=u32 0, x=w990) -> (*(type *) &x=w994:u32)
            n148 = Divide(x=u32 1, y=u32 1000) -> (x/y=w995:dbl)
            n149 = Multiply(x=w995, y=w994) -> (x*y=w991:dbl)
          }
          frame 82 {
            n150 = Type Cast(type=0, x=w1003) -> (*(type *) &x=w1007:i32)
            n151 = Divide(x=u32 1, y=u32 1000) -> (x/y=w1008:dbl)
            n152 = Multiply(x=w1008, y=w1007) -> (x*y=w1005:dbl)
          }
          frame 84 {
            n153 = Type Cast(type=0, x=w1017) -> (*(type *) &x=w1022:i32)
            n154 = Multiply(x=u32 1, y=w1022) -> (x*y=w1020:u32)
          }
          frame 88 {
            n155 = Type Cast(type=u32 0, x=w1029) -> (*(type *) &x=w1033:u32)
            n156 = Divide(x=u32 1, y=u32 1000) -> (x/y=w1034:dbl)
            n157 = Multiply(x=w1034, y=w1033) -> (x*y=w1031:dbl)
          }
          frame 90 {
            n158 = Type Cast(type=u32 0, x=w1043) -> (*(type *) &x=w1048:u32)
            n159 = Multiply(x=u32 1, y=w1048) -> (x*y=w1046:u32)
          }
          frame 92 {
            n160 = Type Cast(type=u32 0, x=w1055) -> (*(type *) &x=w1059:u32)
            n161 = Divide(x=u32 1, y=u32 1000) -> (x/y=w1060:dbl)
            n162 = Multiply(x=w1060, y=w1059) -> (x*y=w1057:dbl)
          }
          frame 94 {
            n163 = Type Cast(type=u32 0, x=w1069) -> (*(type *) &x=w1074:u32)
            n164 = Multiply(x=1, y=w1074) -> (x*y=w1072:u32)
          }
          frame 96, Default {
            n165 = Type Cast(type=u16 0, x=w1081) -> (*(type *) &x=w1086:u16)
            n166 = Multiply(x=1, y=w1086) -> (x*y=w1083:i32)
          }
        }
        "DC VOLT" <- w573
        "DC-CURRENT" <- w568
        "INVERT-DC-POWER" <- w449
        "DC-POWER" <- w567
        "INVERT-DC-CURRENT" <- w450
        "CHARGE-DC-CURRENT" <- w448
        "CHARGE-DC-POWER" <- w447
        n167 = case shown="96, Default" w502 {
          tunnel: [w796 w812 w823 w835 w849 w861 w875 w887] -> w561
          tunnel: [w795 w809 w827 w834 w848 w860 w874 w886] -> w562
          tunnel: [w793 w807 w821 w833 w853 w858 w872 w884] -> w440
          tunnel: [w791 w805 w819 w831 w845 w857 w879 w882] -> w438
          tunnel: [w794 w808 w822 w838 w847 w859 w873 w885] -> w441
          tunnel: [w792 w806 w820 w832 w846 w864 w871 w883] -> w439
          tunnel: [w790 w804 w818 w830 w844 w856 w870 w890] -> w563
          tunnel: [w798 w811 w825 w837 w851 w863 w877 w889] -> w556
          tunnel: w557 -> [_ w811 w825 w837 w851 w863 w877 w889]
          tunnel: w558 -> [w797 w810 w824 w836 w850 w862 w876 w888]
          tunnel: w559 -> [w796 _ w823 w835 w849 w861 w875 w887]
          tunnel: w560 -> [w795 w809 _ w834 w848 w860 w874 w886]
          tunnel: w445 -> [w794 w808 w822 _ w847 w859 w873 w885]
          tunnel: w444 -> [w793 w807 w821 w833 _ w858 w872 w884]
          tunnel: w443 -> [w792 w806 w820 w832 w846 _ w871 w883]
          tunnel: w442 -> [w791 w805 w819 w831 w845 w857 _ w882]
          tunnel: w564 -> [w790 w804 w818 w830 w844 w856 w870 _]
          frame 80 {
            n168 = Type Cast(type=u32 0, x=w797) -> (*(type *) &x=w801:u32)
            n169 = Divide(x=u32 1, y=u32 1000) -> (x/y=w802:dbl)
            n170 = Multiply(x=w802, y=w801) -> (x*y=w798:dbl)
          }
          frame 82 {
            n171 = Type Cast(type=0, x=w810) -> (*(type *) &x=w814:i32)
            n172 = Divide(x=u32 1, y=u32 1000) -> (x/y=w815:dbl)
            n173 = Multiply(x=w815, y=w814) -> (x*y=w812:dbl)
          }
          frame 84 {
            n174 = Type Cast(type=0, x=w824) -> (*(type *) &x=w829:i32)
            n175 = Multiply(x=u32 1, y=w829) -> (x*y=w827:u32)
          }
          frame 88 {
            n176 = Type Cast(type=u32 0, x=w836) -> (*(type *) &x=w840:u32)
            n177 = Divide(x=u32 1, y=u32 1000) -> (x/y=w841:dbl)
            n178 = Multiply(x=w841, y=w840) -> (x*y=w838:dbl)
          }
          frame 90 {
            n179 = Type Cast(type=u32 0, x=w850) -> (*(type *) &x=w855:u32)
            n180 = Multiply(x=u32 1, y=w855) -> (x*y=w853:u32)
          }
          frame 92 {
            n181 = Type Cast(type=u32 0, x=w862) -> (*(type *) &x=w866:u32)
            n182 = Divide(x=u32 1, y=u32 1000) -> (x/y=w867:dbl)
            n183 = Multiply(x=w867, y=w866) -> (x*y=w864:dbl)
          }
          frame 94 {
            n184 = Type Cast(type=u32 0, x=w876) -> (*(type *) &x=w881:u32)
            n185 = Multiply(x=1, y=w881) -> (x*y=w879:u32)
          }
          frame 96, Default {
            n186 = Type Cast(type=u16 0, x=w888) -> (*(type *) &x=w893:u16)
            n187 = Multiply(x=1, y=w893) -> (x*y=w890:i32)
          }
        }
        "DC VOLT 2" <- w556
        "DC-CURRENT 2" <- w561
        "INVERT-DC-POWER 2" <- w440
        "DC-POWER 2" <- w562
        "INVERT-DC-CURRENT 2" <- w441
        "CHARGE-DC-CURRENT 2" <- w439
        "CHARGE-DC-POWER 2" <- w438
        n188 = shared-variable "SBU-cRIO\\Variables for FPGA V4.lvlib\\Time"() -> (w362:dbl)  [unwired: 1 in, 1 out]
        n189 = shared-variable "SBU-cRIO\\Variables for FPGA V4.lvlib\\Time"() -> (w359:dbl)  [unwired: 1 in, 1 out]
        n190 = shared-variable "SBU-cRIO\\Variables for FPGA V4.lvlib\\Time"() -> (w410:dbl)  [unwired: 1 in, 1 out]
        n191 = shared-variable "SBU-cRIO\\Variables for FPGA V4.lvlib\\Time"() -> (w361:dbl)  [unwired: 1 in, 1 out]
        n192 = shared-variable "SBU-cRIO\\Variables for FPGA V4.lvlib\\Time"() -> (w381:dbl)  [unwired: 1 in, 1 out]
        n193 = shared-variable "SBU-cRIO\\Variables for FPGA V4.lvlib\\Time"() -> (w360:dbl)  [unwired: 1 in, 1 out]
        n194 = Build Array (concatenate)(w352, w362) -> (w342:dbl[])
        n195 = Build Array (concatenate)(w276, w359) -> (w264:dbl[])
        n196 = Build Array (concatenate)(w409, w410) -> (w382:dbl[])
        n197 = Build Array (concatenate)(w328, w361) -> (w316:dbl[])
        n198 = Build Array (concatenate)(w380, w381) -> (w372:dbl[])
        n199 = Build Array (concatenate)(w306, w360) -> (w290:dbl[])
        n200 = Build Array (concatenate)(w586, w494) -> (w398:dbl[])
        n201 = Build Array (concatenate)(w585, w490) -> (w396:dbl[])
        n202 = Build Array (concatenate)(w584, w486) -> (w394:dbl[])
        n203 = Build Array (concatenate)(w581, w492) -> (w392:dbl[])
        n204 = Build Array (concatenate)(w582, w488) -> (w390:dbl[])
        n205 = Build Array (concatenate)(w583, w484) -> (w388:dbl[])
        n206 = Build Array (concatenate)(w514, w513) -> (w419:dbl[])
        n207 = Build Array (concatenate)(w574, w573) -> (w429:dbl[])
        n208 = Build Array (concatenate)(w555, w556) -> (w424:dbl[])
        n209 = Build Array (concatenate)(w526, w465) -> (w288:dbl[])
        n210 = Build Array (concatenate)(w525, w464) -> (w286:dbl[])
        n211 = Build Array (concatenate)(w524, w463) -> (w284:dbl[])
        n212 = Build Array (concatenate)(w515, w508) -> (w418:dbl[])
        n213 = Build Array (concatenate)(w516, w507) -> (w417:dbl[])
        n214 = Build Array (concatenate)(w517, w433) -> (w262:dbl[])
        n215 = Build Array (concatenate)(w518, w432) -> (w260:dbl[])
        n216 = Build Array (concatenate)(w575, w568) -> (w428:dbl[])
        n217 = Build Array (concatenate)(w576, w567) -> (w427:dbl[])
        n218 = Build Array (concatenate)(w577, w450) -> (w370:dbl[])
        n219 = Build Array (concatenate)(w578, w449) -> (w368:dbl[])
        n220 = Build Array (concatenate)(w543, w482) -> (w340:dbl[])
        n221 = Build Array (concatenate)(w544, w478) -> (w338:dbl[])
        n222 = Build Array (concatenate)(w545, w474) -> (w336:dbl[])
        n223 = Build Array (concatenate)(w554, w561) -> (w423:dbl[])
        n224 = Build Array (concatenate)(w553, w562) -> (w422:dbl[])
        n225 = Build Array (concatenate)(w552, w441) -> (w314:dbl[])
        n226 = Build Array (concatenate)(w551, w440) -> (w312:dbl[])
        n227 = Build Array (concatenate)(w521, w462) -> (w282:dbl[])
        n228 = Build Array (concatenate)(w522, w461) -> (w280:dbl[])
        n229 = Build Array (concatenate)(w523, w460) -> (w278:dbl[])
        n230 = Build Array (concatenate)(w520, w431) -> (w258:dbl[])
        n231 = Build Array (concatenate)(w519, w430) -> (w256:dbl[])
        n232 = Build Array (concatenate)(w580, w448) -> (w366:dbl[])
        n233 = Build Array (concatenate)(w579, w447) -> (w364:dbl[])
        n234 = Build Array (concatenate)(w548, w480) -> (w330:dbl[])
        n235 = Build Array (concatenate)(w547, w476) -> (w332:dbl[])
        n236 = Build Array (concatenate)(w546, w472) -> (w334:dbl[])
        n237 = Build Array (concatenate)(w549, w439) -> (w310:dbl[])
        n238 = Build Array (concatenate)(w550, w438) -> (w308:dbl[])
        n239 = Bundle(w382, w428) -> ()  [unwired: 1 in, 1 out]
        n240 = Bundle(w382, w427) -> ()  [unwired: 1 in, 1 out]
        n241 = Bundle(w382, w370) -> (w383:cluster{dbl[], dbl[]})  [unwired: 1 in]
        n242 = Bundle(w382, w368) -> (w385:cluster{dbl[], dbl[]})  [unwired: 1 in]
        n243 = Bundle(w382, w429) -> ()  [unwired: 1 in, 1 out]
        n244 = Bundle(w382, w366) -> (w384:cluster{dbl[], dbl[]})  [unwired: 1 in]
        n245 = Bundle(w382, w364) -> (w386:cluster{dbl[], dbl[]})  [unwired: 1 in]
        n246 = Bundle(w264, w418) -> ()  [unwired: 1 in, 1 out]
        n247 = Bundle(w264, w417) -> ()  [unwired: 1 in, 1 out]
        n248 = Bundle(w264, w262) -> (w272:cluster{dbl[], dbl[]})  [unwired: 1 in]
        n249 = Bundle(w264, w260) -> (w274:cluster{dbl[], dbl[]})  [unwired: 1 in]
        n250 = Bundle(w264, w419) -> ()  [unwired: 1 in, 1 out]
        n251 = Bundle(w264, w258) -> (w273:cluster{dbl[], dbl[]})  [unwired: 1 in]
        n252 = Bundle(w264, w256) -> (w275:cluster{dbl[], dbl[]})  [unwired: 1 in]
        n253 = Bundle(w342, w340) -> (w358:cluster{dbl[], dbl[]})  [unwired: 1 in]
        n254 = Bundle(w342, w338) -> (w356:cluster{dbl[], dbl[]})  [unwired: 1 in]
        n255 = Bundle(w342, w336) -> (w354:cluster{dbl[], dbl[]})  [unwired: 1 in]
        n256 = Bundle(w342, w330) -> (w357:cluster{dbl[], dbl[]})  [unwired: 1 in]
        n257 = Bundle(w342, w332) -> (w355:cluster{dbl[], dbl[]})  [unwired: 1 in]
        n258 = Bundle(w342, w334) -> (w353:cluster{dbl[], dbl[]})  [unwired: 1 in]
        n259 = Bundle(w316, w423) -> ()  [unwired: 1 in, 1 out]
        n260 = Bundle(w316, w422) -> ()  [unwired: 1 in, 1 out]
        n261 = Bundle(w316, w314) -> (w324:cluster{dbl[], dbl[]})  [unwired: 1 in]
        n262 = Bundle(w316, w312) -> (w326:cluster{dbl[], dbl[]})  [unwired: 1 in]
        n263 = Bundle(w290, w288) -> (w305:cluster{dbl[], dbl[]})  [unwired: 1 in]
        n264 = Bundle(w290, w286) -> (w303:cluster{dbl[], dbl[]})  [unwired: 1 in]
        n265 = Bundle(w290, w284) -> (w301:cluster{dbl[], dbl[]})  [unwired: 1 in]
        n266 = Bundle(w316, w424) -> ()  [unwired: 1 in, 1 out]
        n267 = Bundle(w316, w310) -> (w325:cluster{dbl[], dbl[]})  [unwired: 1 in]
        n268 = Bundle(w316, w308) -> (w327:cluster{dbl[], dbl[]})  [unwired: 1 in]
        n269 = Bundle(w290, w282) -> (w304:cluster{dbl[], dbl[]})  [unwired: 1 in]
        n270 = Bundle(w290, w280) -> (w302:cluster{dbl[], dbl[]})  [unwired: 1 in]
        n271 = Bundle(w290, w278) -> (w300:cluster{dbl[], dbl[]})  [unwired: 1 in]
        n272 = Bundle(w382, w398) -> (w416:cluster{dbl[], dbl[]})  [unwired: 1 in]
        n273 = Bundle(w382, w396) -> (w414:cluster{dbl[], dbl[]})  [unwired: 1 in]
        n274 = Bundle(w382, w394) -> (w412:cluster{dbl[], dbl[]})  [unwired: 1 in]
        n275 = Bundle(w382, w392) -> (w415:cluster{dbl[], dbl[]})  [unwired: 1 in]
        n276 = Bundle(w382, w390) -> (w413:cluster{dbl[], dbl[]})  [unwired: 1 in]
        n277 = Bundle(w382, w388) -> (w411:cluster{dbl[], dbl[]})  [unwired: 1 in]
        n278 = Build Array(w326, w327) -> (→"DC Power 2":cluster{dbl[], dbl[]}[])
        n279 = Build Array(w324, w325) -> (→"DC Current 2":cluster{dbl[], dbl[]}[])
        n280 = Build Array(w305, w304) -> (→"AC Voltage 3":cluster{dbl[], dbl[]}[])
        n281 = Build Array(w303, w302) -> (→"AC Current 3":cluster{dbl[], dbl[]}[])
        n282 = Build Array(w301, w300) -> (→"AC Power 3":cluster{dbl[], dbl[]}[])
        n283 = Build Array(w358, w357) -> (→"AC Voltage 2":cluster{dbl[], dbl[]}[])
        n284 = Build Array(w356, w355) -> (→"AC Current 2":cluster{dbl[], dbl[]}[])
        n285 = Build Array(w354, w353) -> (→"AC Power 2":cluster{dbl[], dbl[]}[])
        n286 = Build Array(w385, w386) -> (→"DC Power":cluster{dbl[], dbl[]}[])
        n287 = Build Array(w383, w384) -> (→"DC Current":cluster{dbl[], dbl[]}[])
        n288 = Build Array(w274, w275) -> (→"DC Power 3":cluster{dbl[], dbl[]}[])
        n289 = Build Array(w272, w273) -> (→"DC Current 3":cluster{dbl[], dbl[]}[])
        n290 = Build Array(w416, w415) -> (→"AC Voltage 1":cluster{dbl[], dbl[]}[])
        n291 = Build Array(w414, w413) -> (→"AC Current 1":cluster{dbl[], dbl[]}[])
        n292 = Build Array(w412, w411) -> (→"AC Power 1":cluster{dbl[], dbl[]}[])
        n293 = feedback #1() -> (w400:bool)  [unwired: 1 in]
        n294 = call "RyanRemove.vi"("Boolean"=w400, "IN"=w382) -> ("OUT"=w399:dbl[])  [unwired: 9 in]
        n295 = call "RyanRemove.vi"("Boolean"=w400, "IN"=w398) -> ("OUT"=w397:dbl[])  [unwired: 9 in]
        n296 = call "RyanTestComp.vi"("NEW"=w397, "OLD"=w398) -> ("Boolean"=w407:bool)  [unwired: 9 in]
        n297 = call "RyanRemove.vi"("Boolean"=w400, "IN"=w396) -> ("OUT"=w395:dbl[])  [unwired: 9 in]
        n298 = call "RyanTestComp.vi"("NEW"=w395, "OLD"=w396) -> ("Boolean"=w406:bool)  [unwired: 9 in]
        n299 = call "RyanRemove.vi"("Boolean"=w400, "IN"=w394) -> ("OUT"=w393:dbl[])  [unwired: 9 in]
        n300 = call "RyanTestComp.vi"("NEW"=w393, "OLD"=w394) -> ("Boolean"=w405:bool)  [unwired: 9 in]
        n301 = call "RyanRemove.vi"("Boolean"=w400, "IN"=w392) -> ("OUT"=w391:dbl[])  [unwired: 9 in]
        n302 = call "RyanTestComp.vi"("NEW"=w391, "OLD"=w392) -> ("Boolean"=w404:bool)  [unwired: 9 in]
        n303 = call "RyanRemove.vi"("Boolean"=w400, "IN"=w390) -> ("OUT"=w389:dbl[])  [unwired: 9 in]
        n304 = call "RyanTestComp.vi"("NEW"=w389, "OLD"=w390) -> ("Boolean"=w403:bool)  [unwired: 9 in]
        n305 = call "RyanRemove.vi"("Boolean"=w400, "IN"=w388) -> ("OUT"=w387:dbl[])  [unwired: 9 in]
        n306 = call "RyanTestComp.vi"("NEW"=w387, "OLD"=w388) -> ("Boolean"=w401:bool)  [unwired: 9 in]
        n307 = Build Array(w407, w406, w405, w404, w403, w401) -> (w408:bool[])
        n308 = feedback #2() -> (w343:bool)  [unwired: 1 in]
        n309 = call "RyanRemove.vi"("Boolean"=w343, "IN"=w342) -> ("OUT"=w341:dbl[])  [unwired: 9 in]
        n310 = call "RyanRemove.vi"("Boolean"=w343, "IN"=w340) -> ("OUT"=w339:dbl[])  [unwired: 9 in]
        n311 = call "RyanTestComp.vi"("NEW"=w339, "OLD"=w340) -> ("Boolean"=w350:bool)  [unwired: 9 in]
        n312 = call "RyanRemove.vi"("Boolean"=w343, "IN"=w338) -> ("OUT"=w337:dbl[])  [unwired: 9 in]
        n313 = call "RyanTestComp.vi"("NEW"=w337, "OLD"=w338) -> ("Boolean"=w349:bool)  [unwired: 9 in]
        n314 = call "RyanRemove.vi"("Boolean"=w343, "IN"=w336) -> ("OUT"=w335:dbl[])  [unwired: 9 in]
        n315 = call "RyanTestComp.vi"("NEW"=w335, "OLD"=w336) -> ("Boolean"=w348:bool)  [unwired: 9 in]
        n316 = call "RyanRemove.vi"("Boolean"=w343, "IN"=w330) -> ("OUT"=w329:dbl[])  [unwired: 9 in]
        n317 = call "RyanTestComp.vi"("NEW"=w329, "OLD"=w330) -> ("Boolean"=w347:bool)  [unwired: 9 in]
        n318 = call "RyanRemove.vi"("Boolean"=w343, "IN"=w332) -> ("OUT"=w331:dbl[])  [unwired: 9 in]
        n319 = call "RyanTestComp.vi"("NEW"=w331, "OLD"=w332) -> ("Boolean"=w346:bool)  [unwired: 9 in]
        n320 = call "RyanRemove.vi"("Boolean"=w343, "IN"=w334) -> ("OUT"=w333:dbl[])  [unwired: 9 in]
        n321 = call "RyanTestComp.vi"("NEW"=w333, "OLD"=w334) -> ("Boolean"=w344:bool)  [unwired: 9 in]
        n322 = Build Array(w350, w349, w348, w347, w346, w344) -> (w351:bool[])
        n323 = feedback #3() -> (w291:bool)  [unwired: 1 in]
        n324 = call "RyanRemove.vi"("Boolean"=w291, "IN"=w290) -> ("OUT"=w289:dbl[])  [unwired: 9 in]
        n325 = call "RyanRemove.vi"("Boolean"=w291, "IN"=w288) -> ("OUT"=w287:dbl[])  [unwired: 9 in]
        n326 = call "RyanTestComp.vi"("NEW"=w287, "OLD"=w288) -> ("Boolean"=w298:bool)  [unwired: 9 in]
        n327 = call "RyanRemove.vi"("Boolean"=w291, "IN"=w286) -> ("OUT"=w285:dbl[])  [unwired: 9 in]
        n328 = call "RyanTestComp.vi"("NEW"=w285, "OLD"=w286) -> ("Boolean"=w297:bool)  [unwired: 9 in]
        n329 = call "RyanRemove.vi"("Boolean"=w291, "IN"=w284) -> ("OUT"=w283:dbl[])  [unwired: 9 in]
        n330 = call "RyanTestComp.vi"("NEW"=w283, "OLD"=w284) -> ("Boolean"=w296:bool)  [unwired: 9 in]
        n331 = call "RyanRemove.vi"("Boolean"=w291, "IN"=w282) -> ("OUT"=w281:dbl[])  [unwired: 9 in]
        n332 = call "RyanTestComp.vi"("NEW"=w281, "OLD"=w282) -> ("Boolean"=w295:bool)  [unwired: 9 in]
        n333 = call "RyanRemove.vi"("Boolean"=w291, "IN"=w280) -> ("OUT"=w279:dbl[])  [unwired: 9 in]
        n334 = call "RyanTestComp.vi"("NEW"=w279, "OLD"=w280) -> ("Boolean"=w294:bool)  [unwired: 9 in]
        n335 = call "RyanRemove.vi"("Boolean"=w291, "IN"=w278) -> ("OUT"=w277:dbl[])  [unwired: 9 in]
        n336 = call "RyanTestComp.vi"("NEW"=w277, "OLD"=w278) -> ("Boolean"=w292:bool)  [unwired: 9 in]
        n337 = feedback #4() -> (w373:bool)  [unwired: 1 in]
        n338 = call "RyanRemove.vi"("Boolean"=w373, "IN"=w372) -> ("OUT"=w371:dbl[])  [unwired: 9 in]
        n339 = call "RyanRemove.vi"("Boolean"=w373, "IN"=w370) -> ("OUT"=w369:dbl[])  [unwired: 9 in]
        n340 = call "RyanTestComp.vi"("NEW"=w369, "OLD"=w370) -> ("Boolean"=w378:bool)  [unwired: 9 in]
        n341 = call "RyanRemove.vi"("Boolean"=w373, "IN"=w368) -> ("OUT"=w367:dbl[])  [unwired: 9 in]
        n342 = call "RyanTestComp.vi"("NEW"=w367, "OLD"=w368) -> ("Boolean"=w377:bool)  [unwired: 9 in]
        n343 = call "RyanRemove.vi"("Boolean"=w373, "IN"=w366) -> ("OUT"=w365:dbl[])  [unwired: 9 in]
        n344 = call "RyanTestComp.vi"("NEW"=w365, "OLD"=w366) -> ("Boolean"=w376:bool)  [unwired: 9 in]
        n345 = call "RyanRemove.vi"("Boolean"=w373, "IN"=w364) -> ("OUT"=w363:dbl[])  [unwired: 9 in]
        n346 = call "RyanTestComp.vi"("NEW"=w363, "OLD"=w364) -> ("Boolean"=w375:bool)  [unwired: 9 in]
        n347 = Build Array(w378, w377, w376, w375) -> (w379:bool[])
        n348 = feedback #5() -> (w317:bool)  [unwired: 1 in]
        n349 = call "RyanRemove.vi"("Boolean"=w317, "IN"=w316) -> ("OUT"=w315:dbl[])  [unwired: 9 in]
        n350 = call "RyanRemove.vi"("Boolean"=w317, "IN"=w314) -> ("OUT"=w313:dbl[])  [unwired: 9 in]
        n351 = call "RyanTestComp.vi"("NEW"=w313, "OLD"=w314) -> ("Boolean"=w322:bool)  [unwired: 9 in]
        n352 = call "RyanRemove.vi"("Boolean"=w317, "IN"=w312) -> ("OUT"=w311:dbl[])  [unwired: 9 in]
        n353 = call "RyanTestComp.vi"("NEW"=w311, "OLD"=w312) -> ("Boolean"=w321:bool)  [unwired: 9 in]
        n354 = call "RyanRemove.vi"("Boolean"=w317, "IN"=w310) -> ("OUT"=w309:dbl[])  [unwired: 9 in]
        n355 = call "RyanTestComp.vi"("NEW"=w309, "OLD"=w310) -> ("Boolean"=w320:bool)  [unwired: 9 in]
        n356 = call "RyanRemove.vi"("Boolean"=w317, "IN"=w308) -> ("OUT"=w307:dbl[])  [unwired: 9 in]
        n357 = call "RyanTestComp.vi"("NEW"=w307, "OLD"=w308) -> ("Boolean"=w319:bool)  [unwired: 9 in]
        n358 = Build Array(w322, w321, w320, w319) -> (w323:bool[])
        n359 = Or Array Elements(Boolean array=w351) -> (logical OR=w345:bool)
        n360 = feedback-in #2(w345) -> ()
        n361 = Build Array(w298, w297, w296, w295, w294, w292) -> (w299:bool[])
        n362 = Or Array Elements(Boolean array=w379) -> (logical OR=w374:bool)
        n363 = feedback-in #4(w374) -> ()
        n364 = Or Array Elements(Boolean array=w408) -> (logical OR=w402:bool)
        n365 = feedback-in #1(w402) -> ()
        n366 = feedback #6() -> (w265:bool)  [unwired: 1 in]
        n367 = call "RyanRemove.vi"("Boolean"=w265, "IN"=w264) -> ("OUT"=w263:dbl[])  [unwired: 9 in]
        n368 = call "RyanRemove.vi"("Boolean"=w265, "IN"=w262) -> ("OUT"=w261:dbl[])  [unwired: 9 in]
        n369 = call "RyanTestComp.vi"("NEW"=w261, "OLD"=w262) -> ("Boolean"=w270:bool)  [unwired: 9 in]
        n370 = call "RyanRemove.vi"("Boolean"=w265, "IN"=w260) -> ("OUT"=w259:dbl[])  [unwired: 9 in]
        n371 = call "RyanTestComp.vi"("NEW"=w259, "OLD"=w260) -> ("Boolean"=w269:bool)  [unwired: 9 in]
        n372 = call "RyanRemove.vi"("Boolean"=w265, "IN"=w258) -> ("OUT"=w257:dbl[])  [unwired: 9 in]
        n373 = call "RyanTestComp.vi"("NEW"=w257, "OLD"=w258) -> ("Boolean"=w268:bool)  [unwired: 9 in]
        n374 = call "RyanRemove.vi"("Boolean"=w265, "IN"=w256) -> ("OUT"=w255:dbl[])  [unwired: 9 in]
        n375 = call "RyanTestComp.vi"("NEW"=w255, "OLD"=w256) -> ("Boolean"=w267:bool)  [unwired: 9 in]
        n376 = Build Array(w270, w269, w268, w267) -> (w271:bool[])
        n377 = Or Array Elements(Boolean array=w323) -> (logical OR=w318:bool)
        n378 = feedback-in #5(w318) -> ()
        n379 = Or Array Elements(Boolean array=w271) -> (logical OR=w266:bool)
        n380 = feedback-in #6(w266) -> ()
        n381 = Or Array Elements(Boolean array=w299) -> (logical OR=w293:bool)
        n382 = feedback-in #3(w293) -> ()
      }
      n383 = while {
        shift-right: [w1678] -> w140
        shift-left: w137 -> [w1516]
        shift-right: [w1677] -> w139
        shift-left: w136 -> [w1515]
        tunnel: 0 -> [w1683]
        shift-right: [w1365] -> _
        shift-left: w135 -> [w1409]
        shift-right: [w1225] -> _
        shift-left: w135 -> [w1408]
        shift-right: [w1216] -> _
        shift-left: w135 -> [w1407]
        shift-right: [w1203] -> _
        shift-left: w135 -> [w1406]
        shift-right: [w1411] -> _
        shift-left: w133 -> [w1737]
        shift-right: [w1221] -> _
        shift-left: w133 -> [w1729]
        shift-right: [w1215] -> _
        shift-left: w133 -> [w1736]
        shift-right: [w1205] -> _
        shift-left: w133 -> [w1735]
        shift-right: [w1386] -> _
        shift-left: w130 -> [w1391]
        shift-right: [w1220] -> _
        shift-left: w130 -> [w1390]
        shift-right: [w1212] -> _
        shift-left: w130 -> [w1389]
        shift-right: [w1206] -> _
        shift-left: w130 -> [w1388]
        shift-right: [w1377] -> _
        shift-left: w132 -> [w1382]
        shift-right: [w1218] -> _
        shift-left: w132 -> [w1381]
        shift-right: [w1213] -> _
        shift-left: w132 -> [w1380]
        shift-right: [w1207] -> _
        shift-left: w132 -> [w1379]
        shift-right: [w1412] -> _
        shift-left: w131 -> [w1734]
        shift-right: [w1217] -> _
        shift-left: w131 -> [w1733]
        shift-right: [w1211] -> _
        shift-left: w131 -> [w1732]
        shift-right: [w1208] -> _
        shift-left: w131 -> [w1731]
        shift-right: [w1392] -> _
        shift-left: w134 -> [w1397]
        shift-right: [w1222] -> _
        shift-left: w134 -> [w1396]
        shift-right: [w1214] -> _
        shift-left: w134 -> [w1395]
        shift-right: [w1204] -> _
        shift-left: w134 -> [w1394]
        shift-right: [w1198] -> _
        shift-left: w135 -> [w1405]
        shift-right: [w1195] -> _
        shift-left: w134 -> [w1393]
        shift-right: [w1196] -> _
        shift-left: w133 -> [w1725]
        shift-right: [w1194] -> _
        shift-left: w130 -> [w1387]
        shift-right: [w1192] -> _
        shift-left: w132 -> [w1378]
        shift-right: [w1193] -> _
        shift-left: w131 -> [w1724]
        tunnel: [w1694] -> w129
        tunnel: [w1693] -> w128
        tunnel: [w1692] -> w127
        tunnel: [w1691] -> w126
        tunnel: w125 -> [w1690]
        tunnel: w124 -> [w1689]
        tunnel: w123 -> [w1688]
        tunnel: w122 -> [w1687]
        shift-right: [w1654] -> _
        shift-left: _ -> [w1655]
        shift-right: [w1652] -> _
        shift-left: _ -> [w1653]
        shift-right: [w1650] -> _
        shift-left: _ -> [w1651]
        shift-right: [w1648] -> _
        shift-left: _ -> [w1649]
        shift-right: [w1646] -> _
        shift-left: _ -> [w1647]
        shift-right: [w1644] -> _
        shift-left: _ -> [w1645]
        shift-right: [w1630] -> _
        shift-left: _ -> [w1643]
        shift-right: [w1641] -> _
        shift-left: _ -> [w1642]
        shift-right: [w1628] -> _
        shift-left: _ -> [w1640]
        shift-right: [w1638] -> _
        shift-left: _ -> [w1639]
        shift-right: [w1626] -> _
        shift-left: _ -> [w1637]
        shift-right: [w1625] -> _
        shift-left: _ -> [w1636]
        shift-right: [w1634] -> _
        shift-left: _ -> [w1635]
        shift-right: [w1632] -> _
        shift-left: _ -> [w1633]
        shift-right: [w1631] -> _
        shift-left: _ -> [w1518]
        shift-right: [w1621] -> _
        shift-left: _ -> [w1610]
        shift-right: [w1620] -> _
        shift-left: _ -> [w1609]
        shift-right: [w1619] -> _
        shift-left: _ -> [w1608]
        shift-right: [w1618] -> _
        shift-left: _ -> [w1607]
        shift-right: [w1617] -> _
        shift-left: _ -> [w1606]
        shift-right: [w1616] -> _
        shift-left: _ -> [w1517]
        shift-right: [w1593] -> _
        shift-left: _ -> [w1605]
        shift-right: [w1615] -> _
        shift-left: _ -> [w1604]
        shift-right: [w1594] -> _
        shift-left: _ -> [w1603]
        shift-right: [w1614] -> _
        shift-left: _ -> [w1602]
        shift-right: [w1592] -> _
        shift-left: _ -> [w1597]
        shift-right: [w1591] -> _
        shift-left: _ -> [w1601]
        shift-right: [w1613] -> _
        shift-left: _ -> [w1600]
        shift-right: [w1612] -> _
        shift-left: _ -> [w1599]
        shift-right: [w1611] -> _
        shift-left: _ -> [w1598]
        shift-right: [w1376] -> _
        shift-left: 0.0 -> [w1371]
        shift-right: [w1219] -> _
        shift-left: 0.0 -> [w1373]
        shift-right: [w1587] -> _
        shift-left: _ -> [w1570]
        shift-right: [w1586] -> _
        shift-left: _ -> [w1569]
        shift-right: [w1585] -> _
        shift-left: _ -> [w1568]
        shift-right: [w1584] -> _
        shift-left: _ -> [w1567]
        shift-right: [w1583] -> _
        shift-left: _ -> [w1566]
        shift-right: [w1582] -> _
        shift-left: _ -> [w1565]
        shift-right: [w1573] -> _
        shift-left: _ -> [w1564]
        shift-right: [w1581] -> _
        shift-left: _ -> [w1563]
        shift-right: [w1574] -> _
        shift-left: _ -> [w1562]
        shift-right: [w1580] -> _
        shift-left: _ -> [w1557]
        shift-right: [w1572] -> _
        shift-left: _ -> [w1561]
        shift-right: [w1571] -> _
        shift-left: _ -> [w1560]
        shift-right: [w1579] -> _
        shift-left: _ -> [w1559]
        shift-right: [w1578] -> _
        shift-left: _ -> [w1558]
        shift-right: [w1577] -> _
        shift-left: _ -> [w1556]
        shift-right: [w1210] -> _
        shift-left: 0.0 -> [w1372]
        shift-right: [w1555] -> _
        shift-left: _ -> [w1544]
        shift-right: [w1554] -> _
        shift-left: _ -> [w1543]
        shift-right: [w1553] -> _
        shift-left: _ -> [w1542]
        shift-right: [w1552] -> _
        shift-left: _ -> [w1541]
        shift-right: [w1551] -> _
        shift-left: _ -> [w1540]
        shift-right: [w1550] -> _
        shift-left: _ -> [w1539]
        shift-right: [w1521] -> _
        shift-left: _ -> [w1538]
        shift-right: [w1549] -> _
        shift-left: _ -> [w1537]
        shift-right: [w1522] -> _
        shift-left: _ -> [w1536]
        shift-right: [w1548] -> _
        shift-left: _ -> [w1530]
        shift-right: [w1520] -> _
        shift-left: _ -> [w1529]
        shift-right: [w1519] -> _
        shift-left: _ -> [w1528]
        shift-right: [w1547] -> _
        shift-left: _ -> [w1527]
        shift-right: [w1546] -> _
        shift-left: _ -> [w1526]
        shift-right: [w1545] -> _
        shift-left: _ -> [w1525]
        shift-right: [w1209] -> _
        shift-left: 0.0 -> [w1374]
        shift-right: [w1490] -> _
        shift-left: _ -> [w1473]
        shift-right: [w1484] -> _
        shift-left: _ -> [w1472]
        shift-right: [w1489] -> _
        shift-left: _ -> [w1471]
        shift-right: [w1482] -> _
        shift-left: _ -> [w1470]
        shift-right: [w1488] -> _
        shift-left: _ -> [w1469]
        shift-right: [w1481] -> _
        shift-left: _ -> [w1468]
        shift-right: [w1480] -> _
        shift-left: _ -> [w1467]
        shift-right: [w1487] -> _
        shift-left: _ -> [w1466]
        shift-right: [w1486] -> _
        shift-left: _ -> [w1465]
        shift-right: [w1491] -> _
        shift-left: _ -> [w1474]
        shift-right: [w1492] -> _
        shift-left: _ -> [w1475]
        shift-right: [w1493] -> _
        shift-left: _ -> [w1476]
        shift-right: [w1494] -> _
        shift-left: _ -> [w1477]
        shift-right: [w1485] -> _
        shift-left: _ -> [w1464]
        shift-right: [w1495] -> _
        shift-left: _ -> [w1478]
        shift-right: [w1191] -> _
        shift-left: 0.0 -> [w1375]
        shift-right: [w1354] -> _
        shift-left: _ -> [w1370]
        shift-right: [w1357] -> _
        shift-left: dbl[] [] ("Array") -> [w1462]
        shift-right: [w1353] -> _
        shift-left: _ -> [w1369]
        shift-right: [w1351] -> _
        shift-left: _ -> [w1368]
        shift-right: [w1349] -> _
        shift-left: _ -> [w1367]
        shift-right: [w1347] -> _
        shift-left: _ -> [w1366]
        shift-right: [w1316] -> _
        shift-left: dbl[] [] ("Array") -> [w1461]
        shift-right: [w1314] -> _
        shift-left: dbl[] [] ("Array") -> [w1460]
        shift-right: [w1312] -> _
        shift-left: dbl[] [] ("Array") -> [w1459]
        shift-right: [w1310] -> _
        shift-left: dbl[] [] ("Array") -> [w1458]
        shift-right: [w1308] -> _
        shift-left: dbl[] [] ("Array") -> [w1457]
        shift-right: [w1400] -> _
        shift-left: dbl[] [] ("Array") -> [w1430]
        shift-right: [w1401] -> _
        shift-left: dbl[] [] ("Array") -> [w1431]
        shift-right: [w1402] -> _
        shift-left: dbl[] [] ("Array") -> [w1432]
        shift-right: [w1403] -> _
        shift-left: dbl[] [] ("Array") -> [w1433]
        shift-right: [w1404] -> _
        shift-left: dbl[] [] ("Array") -> [w1434]
        shift-right: [w1291] -> _
        shift-left: dbl[] [] ("Array") -> [w1429]
        shift-right: [w1289] -> _
        shift-left: dbl[] [] ("Array") -> [w1428]
        shift-right: [w1287] -> _
        shift-left: dbl[] [] ("Array") -> [w1427]
        shift-right: [w1285] -> _
        shift-left: dbl[] [] ("Array") -> [w1426]
        shift-right: [w1283] -> _
        shift-left: dbl[] [] ("Array") -> [w1425]
        shift-right: [w1261] -> _
        shift-left: dbl[] [] ("Array") -> [w1419]
        shift-right: [w1259] -> _
        shift-left: dbl[] [] ("Array") -> [w1420]
        shift-right: [w1258] -> _
        shift-left: dbl[] [] ("Array") -> [w1421]
        shift-right: [w1256] -> _
        shift-left: dbl[] [] ("Array") -> [w1422]
        shift-right: [w1254] -> _
        shift-left: dbl[] [] ("Array") -> [w1423]
        shift-right: [w1235] -> _
        shift-left: dbl[] [] ("Array") -> [w1418]
        shift-right: [w1233] -> _
        shift-left: dbl[] [] ("Array") -> [w1417]
        shift-right: [w1231] -> _
        shift-left: dbl[] [] ("Array") -> [w1416]
        shift-right: [w1229] -> _
        shift-left: dbl[] [] ("Array") -> [w1415]
        shift-right: [w1227] -> _
        shift-left: dbl[] [] ("Array") -> [w1414]
        shift-right: [w1318] -> _
        shift-left: dbl[] [] ("Array") -> [w1328]
        shift-right: [w1293] -> _
        shift-left: dbl[] [] ("Array") -> [w1302]
        shift-right: [w1262] -> _
        shift-left: dbl[] [] ("Array") -> [w1277]
        shift-right: [w1237] -> _
        shift-left: dbl[] [] ("Array") -> [w1252]
        stop <- FALSE stop-if-true
        # "CURRENT COMMANDS"
        # "BATTERY MAX: ENERGY COMMANDS"
        # "BATTERY AVAILABLE ENERGY COMMANDS"
        # "BATTERY REM: CAPACITY COMMANDS"
        # "BATTERY CAPACITY COMMANDS"
        # "VOLTAGE COMMANDS"
        n384 = shared-variable "SBU-cRIO\\Variables for FPGA V4.lvlib\\ContModeCap"() -> (w1682:bool)  [unwired: 1 in, 1 out]
        n385 = call "UP-COUNTER-V1.0.vi"("UPPER LIMIT"=u32 36) -> ("COUNT"=w1435:u32)  [unwired: 10 in]
        n386 = call "WRITE VI-V1.vi"("Numeric"=w1683, "error in (no error)"=w1515, "COUNT"=w1435, "BATTERY MEASUREMENTS"=w1682, "VISA Refnum in"=w1516) -> ("error out"=w1680:errorcluster, "Bytes at Port"=w1679:u32, "VISA Refnum out"=w1681:refnum<visa-resource-name>)  [unwired: 4 in]
        n387 = call "Clock"("Auto Reset"=TRUE) -> ("Present (s)"=w1282:dbl)  [unwired: 11 in, 7 out]
        n388 = shared-variable "SBU-cRIO\\Variables for FPGA V4.lvlib\\Time"(w1282) -> ()  [unwired: 1 in, 1 out]
        n389 = call-poly <vilib>:"POST.vi"("client handle"=w1688, "url"="control battery url", "error in (no error)"=w1687) -> ("client handle out"=w1709:T11, "body"=w1705:string, "error out"=w1708:errorcluster)  [unwired: 9 in, 1 out]
        n390 = VISA Read(VISA resource name=w1681, byte count=w1679, error in (no error)=w1680) -> (VISA resource name out=w1678:refnum<visa-resource-name>, read buffer=w1497:string, error out=w1677:errorcluster)  [unwired: 1 out]
        n391 = String To Byte Array(string=w1497) -> (unsigned byte array=w1452:u8[])
        n392 = String Subset(string=w1497) -> (substring=w1663:string)  [unwired: 2 in]
        n393 = String Subset(string=w1497) -> (substring=w1674:string)  [unwired: 2 in]
        n394 = String To Byte Array(string=w1663) -> (unsigned byte array=w1502:u8[])
        n395 = Search 1D Array(1D array=w1452, element=93 ("length (rest)")) -> (index of element=w1455:i32)  [unwired: 1 in]
        n396 = Index Array(array=w1502, index=5) -> (element=w1504:u8)
        n397 = Index Array(array=w1502, index=14) -> (element=w1501:u8)
        n398 = String To Byte Array(string=w1674) -> (unsigned byte array=w1668:u8[])
        n399 = Decrement(x=w1455) -> (x-1=w1453:i32)
        n400 = Index Array(array=w1502, index=12) -> (element=w1531:u8)
        n401 = Index Array(array=w1502, index=14) -> (element=w1659:u8)
        n402 = Index Array(array=w1452, index=w1453) -> (element=w1450:u8)
        n403 = Equal?(x=u8 126 ("y"), y=w1504) -> (x = y?=w1499:bool)
        n404 = Equal?(x=u8 8 ("y"), y=w1501) -> (x = y?=w1498:bool)
        n405 = Index Array(array=w1668, index=6) -> (element=w1672:u8)
        n406 = Index Array(array=w1668, index=8) -> (element=w1669:u8)
        n407 = And(x=w1499, y=w1498) -> (x .and. y?=w1496:bool)
        n408 = Equal?(x=w1659, y=u8 10) -> (x = y?=w1532:bool)
        n409 = Equal?(x=w1531, y=u8 23) -> (x = y?=w1657:bool)
        n410 = Equal?(x=w1531, y=u8 24) -> (x = y?=w1623:bool)
        n411 = Equal?(x=w1450, y=125) -> (x = y?=w1449:bool)
        n412 = Equal?(x=w1450, y=126) -> (x = y?=w1448:bool)
        n413 = Equal?(x=w1669, y=u8 10) -> (x = y?=w1665:bool)
        n414 = Equal?(x=w1672, y=u8 22) -> (x = y?=w1666:bool)
        n415 = Or(x=w1449, y=w1448) -> (x .or. y?=w1447:bool)
        n416 = And(x=w1623, y=w1532) -> (x .and. y?=w1622:bool)
        n417 = And(x=w1666, y=w1665) -> (x .and. y?=w1664:bool)
        n418 = And(x=w1657, y=w1532) -> (x .and. y?=w1656:bool)
        n419 = case shown="True" w1447 {
          tunnel: [w1757 w1760] -> w1437
          tunnel: w1455 -> [_ w1759]
          tunnel: w1452 -> [w1757 w1758]
          frame False {
          }
          frame True {
            n420 = Delete From Array(array=w1758, length=1 ("length (rest)"), index=w1759) -> (array with subset deleted=w1760:u8[])  [unwired: 1 out]
          }
        }
        n421 = Search 1D Array(1D array=w1437, element=94 ("length (rest)")) -> (index of element=w1445:i32)  [unwired: 1 in]
        n422 = Decrement(x=w1445) -> (x-1=w1443:i32)
        n423 = Index Array(array=w1437, index=w1443) -> (element=w1441:u8)
        n424 = Equal?(x=w1441, y=125) -> (x = y?=w1440:bool)
        n425 = Equal?(x=w1441, y=126) -> (x = y?=w1439:bool)
        n426 = Or(x=w1440, y=w1439) -> (x .or. y?=w1438:bool)
        n427 = case shown="True" w1438 {
          tunnel: [w1752 w1755] -> w1436
          tunnel: w1445 -> [_ w1754]
          tunnel: w1437 -> [w1752 w1753]
          frame False {
          }
          frame True {
            n428 = Delete From Array(array=w1753, length=1 ("length (rest)"), index=w1754) -> (array with subset deleted=w1755:u8[])  [unwired: 1 out]
          }
        }
        n429 = Byte Array To String(unsigned byte array=w1436) -> (string=w1463:string)
        n430 = String Subset(string=w1463, offset (0)=5, length (rest)=8 ("length (rest)")) -> (substring=w1456:string)
        n431 = String To Byte Array(string=w1456) -> (unsigned byte array=w1508:u8[])
        n432 = Array To Cluster(array=w1508) -> (cluster=w1747:T12)
        n433 = Unbundle By Name(w1747) -> ("unsigned byte array[0]"=w1750:u8, "unsigned byte array[1]"=w1726:u8, "unsigned byte array[2]"=w1749:u8, "unsigned byte array[3]"=w1424:u8, "unsigned byte array[4]"=w1717:u8, "unsigned byte array[5]"=w1511:u8, "unsigned byte array[6]"=w1512:u8, "unsigned byte array[7]"=w1513:u8, "unsigned byte array[8]"=w1514:u8)
        n434 = case shown="True" w1496 {
          tunnel: [w1781 w1788] -> w1488
          tunnel: [w1780 w1787] -> w1481
          tunnel: [w1779 w1786] -> w1480
          tunnel: [w1778 w1785] -> w1487
          tunnel: [w1777 w1784] -> w1486
          tunnel: [w1776 w1783] -> w1485
          tunnel: w1497 -> [_ w1782]
          tunnel: w1469 -> [w1781 _]
          tunnel: w1468 -> [w1780 _]
          tunnel: w1467 -> [w1779 _]
          tunnel: w1466 -> [w1778 _]
          tunnel: w1465 -> [w1777 _]
          tunnel: w1464 -> [w1776 _]
          frame False {
          }
          frame True {
            n435 = String Subset(string=w1782, offset (0)=0, length (rest)=8 ("length (rest)")) -> (substring=w1796:string)
            n436 = String To Byte Array(string=w1796) -> (unsigned byte array=w1797:u8[])
            n437 = Array To Cluster(array=w1797) -> (cluster=w1792:T12)
            n438 = Unbundle By Name(w1792) -> ("unsigned byte array[0]"=w1788:u8, "unsigned byte array[1]"=w1787:u8, "unsigned byte array[2]"=w1786:u8, "unsigned byte array[3]"=w1785:u8, "unsigned byte array[4]"=w1784:u8, "unsigned byte array[5]"=w1783:u8, "unsigned byte array[6]"=w1791:u8, "unsigned byte array[7]"=w1790:u8, "unsigned byte array[8]"=w1789:u8)
            n439 = Build Array(w1788, w1787, w1786, w1785, w1784, w1783, w1791, w1790, w1789) -> (w1793:u8[])
            n440 = Number To Hexadecimal String(2:w1793) -> ()  [unwired: 1 in, 1 out]
          }
        }
        n441 = Equal?(x=u8 25 ("y"), y=w1531) -> (x = y?=w1589:bool)
        n442 = Equal?(x=u8 26 ("y"), y=w1531) -> (x = y?=w1535:bool)
        n443 = Build Array(w1750, w1726, w1749, w1424, w1717, w1511, w1512, w1513, w1514) -> (w1748:u8[])
        n444 = And(x=w1589, y=w1532) -> (x .and. y?=w1590:bool)
        n445 = And(x=w1535, y=w1532) -> (x .and. y?=w1533:bool)
        n446 = Equal?(x=w1424, y=u32 8) -> (x = y?=w1730:bool)
        n447 = Equal?(x=w1424, y=u32 3) -> (x = y?=w1742:bool)
        n448 = Equal?(x=w1424, y=u32 4) -> (x = y?=w1744:bool)
        n449 = Equal?(x=w1424, y=u32 75) -> (x = y?=w1740:bool)
        n450 = Equal?(x=w1424, y=u32 9) -> (x = y?=w1727:bool)
        n451 = Equal?(x=w1424, y=u32 76) -> (x = y?=w1738:bool)
        n452 = Number To Hexadecimal String(2:w1748) -> ()  [unwired: 1 in, 1 out]
        n453 = case shown="True" w1590 {
          tunnel: w1497 -> [_ w1900]
          tunnel: [w1883 w1899] -> w1580
          tunnel: [w1882 w1898] -> w1572
          tunnel: [w1881 w1897] -> w1571
          tunnel: [w1880 w1896] -> w1579
          tunnel: [w1879 w1895] -> w1578
          tunnel: [w1878 w1894] -> w1577
          tunnel: w1561 -> [w1882 _]
          tunnel: w1560 -> [w1881 _]
          tunnel: w1559 -> [w1880 _]
          tunnel: w1558 -> [w1879 _]
          tunnel: w1557 -> [w1883 _]
          tunnel: w1556 -> [w1878 _]
          tunnel: [w1877 w1893] -> w1555
          tunnel: [w1876 w1892] -> w1554
          tunnel: [w1875 w1891] -> w1553
          tunnel: [w1874 w1890] -> w1552
          tunnel: [w1873 w1889] -> w1551
          tunnel: [w1872 w1888] -> w1550
          tunnel: [w1871 w1887] -> w1521
          tunnel: [w1870 w1886] -> w1549
          tunnel: [w1869 w1885] -> w1522
          tunnel: w1544 -> [w1877 _]
          tunnel: w1543 -> [w1876 _]
          tunnel: w1542 -> [w1875 _]
          tunnel: w1541 -> [w1874 _]
          tunnel: w1540 -> [w1873 _]
          tunnel: w1539 -> [w1872 _]
          tunnel: w1538 -> [w1871 _]
          tunnel: w1537 -> [w1870 _]
          tunnel: w1536 -> [w1869 _]
          frame False {
          }
          frame True {
            n454 = String Subset(string=w1900, offset (0)=0, length (rest)=8 ("length (rest)")) -> (substring=w1910:string)
            n455 = String To Byte Array(string=w1910) -> (unsigned byte array=w1911:u8[])
            n456 = Array To Cluster(array=w1911) -> (cluster=w1906:T12)
            n457 = String Subset(string=w1900, offset (0)=8, length (rest)=14 ("length (rest)")) -> (substring=w1905:string)
            n458 = String To Byte Array(string=w1905) -> (unsigned byte array=w1884:u8[])
            n459 = Array To Cluster(array=w1884) -> (cluster=w1901:T12)
            n460 = Unbundle By Name(w1906) -> ("unsigned byte array[0]"=w1899:u8, "unsigned byte array[1]"=w1898:u8, "unsigned byte array[2]"=w1897:u8, "unsigned byte array[3]"=w1896:u8, "unsigned byte array[4]"=w1895:u8, "unsigned byte array[5]"=w1894:u8, "unsigned byte array[6]"=w1893:u8, "unsigned byte array[7]"=w1892:u8)
            n461 = Unbundle By Name(w1901) -> ("unsigned byte array[0]"=w1891:u8, "unsigned byte array[1]"=w1890:u8, "unsigned byte array[2]"=w1889:u8, "unsigned byte array[3]"=w1888:u8, "unsigned byte array[4]"=w1887:u8, "unsigned byte array[5]"=w1886:u8, "unsigned byte array[6]"=w1885:u8)
            n462 = Build Array(w1899, w1898, w1897, w1896, w1895, w1894, w1893, w1892) -> (w1907:u8[])
            n463 = Build Array(w1891, w1890, w1889, w1888, w1887, w1886, w1885) -> (w1902:u8[])
            n464 = Number To Hexadecimal String(2:w1902) -> ()  [unwired: 1 in, 1 out]
            n465 = Number To Hexadecimal String(2:w1907) -> ()  [unwired: 1 in, 1 out]
          }
        }
        n466 = case shown="True" w1533 {
          tunnel: [w1826 w1842] -> w1548
          tunnel: [w1825 w1841] -> w1520
          tunnel: [w1824 w1840] -> w1519
          tunnel: [w1823 w1839] -> w1547
          tunnel: [w1822 w1838] -> w1546
          tunnel: [w1821 w1837] -> w1545
          tunnel: w1530 -> [w1826 _]
          tunnel: w1529 -> [w1825 _]
          tunnel: w1528 -> [w1824 _]
          tunnel: w1527 -> [w1823 _]
          tunnel: w1526 -> [w1822 _]
          tunnel: w1525 -> [w1821 _]
          tunnel: w1497 -> [_ w1836]
          tunnel: [w1820 w1835] -> w1495
          tunnel: [w1819 w1834] -> w1494
          tunnel: [w1818 w1833] -> w1493
          tunnel: [w1817 w1832] -> w1492
          tunnel: [w1816 w1831] -> w1491
          tunnel: [w1815 w1830] -> w1490
          tunnel: [w1814 w1829] -> w1484
          tunnel: [w1813 w1828] -> w1489
          tunnel: [w1812 w1827] -> w1482
          tunnel: w1478 -> [w1820 _]
          tunnel: w1477 -> [w1819 _]
          tunnel: w1476 -> [w1818 _]
          tunnel: w1475 -> [w1817 _]
          tunnel: w1474 -> [w1816 _]
          tunnel: w1473 -> [w1815 _]
          tunnel: w1472 -> [w1814 _]
          tunnel: w1471 -> [w1813 _]
          tunnel: w1470 -> [w1812 _]
          frame False {
          }
          frame True {
            n467 = String Subset(string=w1836, offset (0)=0, length (rest)=8 ("length (rest)")) -> (substring=w1853:string)
            n468 = String To Byte Array(string=w1853) -> (unsigned byte array=w1854:u8[])
            n469 = Array To Cluster(array=w1854) -> (cluster=w1849:T12)
            n470 = String Subset(string=w1836, offset (0)=8, length (rest)=14 ("length (rest)")) -> (substring=w1847:string)
            n471 = String To Byte Array(string=w1847) -> (unsigned byte array=w1848:u8[])
            n472 = Array To Cluster(array=w1848) -> (cluster=w1843:T12)
            n473 = Unbundle By Name(w1843) -> ("unsigned byte array[0]"=w1833:u8, "unsigned byte array[1]"=w1832:u8, "unsigned byte array[2]"=w1831:u8, "unsigned byte array[3]"=w1830:u8, "unsigned byte array[4]"=w1829:u8, "unsigned byte array[5]"=w1828:u8, "unsigned byte array[6]"=w1827:u8)
            n474 = Unbundle By Name(w1849) -> ("unsigned byte array[0]"=w1842:u8, "unsigned byte array[1]"=w1841:u8, "unsigned byte array[2]"=w1840:u8, "unsigned byte array[3]"=w1839:u8, "unsigned byte array[4]"=w1838:u8, "unsigned byte array[5]"=w1837:u8, "unsigned byte array[6]"=w1835:u8, "unsigned byte array[7]"=w1834:u8)
            n475 = Build Array(w1833, w1832, w1831, w1830, w1829, w1828, w1827) -> (w1844:u8[])
            n476 = Number To Hexadecimal String(2:w1844) -> ()  [unwired: 1 in, 1 out]
            n477 = Build Array(w1842, w1841, w1840, w1839, w1838, w1837, w1835, w1834) -> (w1850:u8[])
            n478 = Number To Hexadecimal String(2:w1850) -> ()  [unwired: 1 in, 1 out]
          }
        }
        n479 = case shown="True" w1622 {
          tunnel: w1497 -> [_ w1956]
          tunnel: [w1940 w1955] -> w1614
          tunnel: [w1939 w1954] -> w1592
          tunnel: [w1938 w1953] -> w1591
          tunnel: [w1937 w1952] -> w1613
          tunnel: [w1936 w1951] -> w1612
          tunnel: [w1935 w1950] -> w1611
          tunnel: w1602 -> [w1940 _]
          tunnel: w1601 -> [w1938 _]
          tunnel: w1600 -> [w1937 _]
          tunnel: w1599 -> [w1936 _]
          tunnel: w1598 -> [w1935 _]
          tunnel: w1597 -> [w1939 _]
          tunnel: [w1934 w1949] -> w1587
          tunnel: [w1933 w1948] -> w1586
          tunnel: [w1932 w1947] -> w1585
          tunnel: [w1931 w1946] -> w1584
          tunnel: [w1930 w1945] -> w1583
          tunnel: [w1929 w1944] -> w1582
          tunnel: [w1928 w1943] -> w1573
          tunnel: [w1927 w1942] -> w1581
          tunnel: [w1926 w1941] -> w1574
          tunnel: w1570 -> [w1934 _]
          tunnel: w1569 -> [w1933 _]
          tunnel: w1568 -> [w1932 _]
          tunnel: w1567 -> [w1931 _]
          tunnel: w1566 -> [w1930 _]
          tunnel: w1565 -> [w1929 _]
          tunnel: w1564 -> [w1928 _]
          tunnel: w1563 -> [w1927 _]
          tunnel: w1562 -> [w1926 _]
          frame False {
          }
          frame True {
            n480 = String Subset(string=w1956, offset (0)=0, length (rest)=8 ("length (rest)")) -> (substring=w1967:string)
            n481 = String To Byte Array(string=w1967) -> (unsigned byte array=w1968:u8[])
            n482 = Array To Cluster(array=w1968) -> (cluster=w1963:T12)
            n483 = String Subset(string=w1956, offset (0)=8, length (rest)=14 ("length (rest)")) -> (substring=w1961:string)
            n484 = String To Byte Array(string=w1961) -> (unsigned byte array=w1962:u8[])
            n485 = Array To Cluster(array=w1962) -> (cluster=w1957:T12)
            n486 = Unbundle By Name(w1957) -> ("unsigned byte array[0]"=w1947:u8, "unsigned byte array[1]"=w1946:u8, "unsigned byte array[2]"=w1945:u8, "unsigned byte array[3]"=w1944:u8, "unsigned byte array[4]"=w1943:u8, "unsigned byte array[5]"=w1942:u8, "unsigned byte array[6]"=w1941:u8)
            n487 = Unbundle By Name(w1963) -> ("unsigned byte array[0]"=w1955:u8, "unsigned byte array[1]"=w1954:u8, "unsigned byte array[2]"=w1953:u8, "unsigned byte array[3]"=w1952:u8, "unsigned byte array[4]"=w1951:u8, "unsigned byte array[5]"=w1950:u8, "unsigned byte array[6]"=w1949:u8, "unsigned byte array[7]"=w1948:u8)
            n488 = Build Array(w1955, w1954, w1953, w1952, w1951, w1950, w1949, w1948) -> (w1964:u8[])
            n489 = Number To Hexadecimal String(2:w1964) -> ()  [unwired: 1 in, 1 out]
            n490 = Build Array(w1947, w1946, w1945, w1944, w1943, w1942, w1941) -> (w1958:u8[])
            n491 = Number To Hexadecimal String(2:w1958) -> ()  [unwired: 1 in, 1 out]
          }
        }
        n492 = case shown="True" w1656 {
          tunnel: w1497 -> [_ w2010]
          tunnel: [w1998 w2019] -> w1638
          tunnel: [w1997 w2020] -> w1626
          tunnel: [w1996 w2018] -> w1625
          tunnel: [w1995 w2017] -> w1634
          tunnel: [w1994 w1999] -> w1632
          tunnel: [w1993 w2016] -> w1631
          tunnel: w1639 -> [w1998 _]
          tunnel: w1637 -> [w1997 _]
          tunnel: w1636 -> [w1996 _]
          tunnel: w1635 -> [w1995 _]
          tunnel: w1633 -> [w1994 _]
          tunnel: w1518 -> [w1993 _]
          tunnel: [w1991 w2009] -> w1621
          tunnel: [w1992 w2008] -> w1620
          tunnel: [w1990 w2001] -> w1619
          tunnel: [w1989 w2002] -> w1618
          tunnel: [w1988 w2003] -> w1617
          tunnel: [w1987 w2004] -> w1616
          tunnel: [w1986 w2005] -> w1593
          tunnel: [w1985 w2006] -> w1615
          tunnel: [w1984 w2007] -> w1594
          tunnel: w1610 -> [w1992 _]
          tunnel: w1609 -> [w1991 _]
          tunnel: w1608 -> [w1990 _]
          tunnel: w1607 -> [w1989 _]
          tunnel: w1606 -> [w1988 _]
          tunnel: w1517 -> [w1987 _]
          tunnel: w1605 -> [w1986 _]
          tunnel: w1604 -> [w1985 _]
          tunnel: w1603 -> [w1984 _]
          frame False {
          }
          frame True {
            n493 = String Subset(string=w2010, offset (0)=8, length (rest)=14 ("length (rest)")) -> (substring=w2014:string)
            n494 = String To Byte Array(string=w2014) -> (unsigned byte array=w2015:u8[])
            n495 = Array To Cluster(array=w2015) -> (cluster=w2011:T12)
            n496 = String Subset(string=w2010, offset (0)=0, length (rest)=8 ("length (rest)")) -> (substring=w2024:string)
            n497 = String To Byte Array(string=w2024) -> (unsigned byte array=w2025:u8[])
            n498 = Array To Cluster(array=w2025) -> (cluster=w2021:T12)
            n499 = Unbundle By Name(w2011) -> ("unsigned byte array[0]"=w2001:u8, "unsigned byte array[1]"=w2002:u8, "unsigned byte array[2]"=w2003:u8, "unsigned byte array[3]"=w2004:u8, "unsigned byte array[4]"=w2005:u8, "unsigned byte array[5]"=w2006:u8, "unsigned byte array[6]"=w2007:u8)
            n500 = Unbundle By Name(w2021) -> ("unsigned byte array[0]"=w2019:u8, "unsigned byte array[1]"=w2020:u8, "unsigned byte array[2]"=w2018:u8, "unsigned byte array[3]"=w2017:u8, "unsigned byte array[4]"=w1999:u8, "unsigned byte array[5]"=w2016:u8, "unsigned byte array[6]"=w2009:u8, "unsigned byte array[7]"=w2008:u8)
            n501 = Build Array(w2001, w2002, w2003, w2004, w2005, w2006, w2007) -> (w2000:u8[])
            n502 = Number To Hexadecimal String(2:w2000) -> ()  [unwired: 1 in, 1 out]
          }
        }
        n503 = case shown="True" w1664 {
          tunnel: w1497 -> [_ w2046]
          tunnel: [w2034 w2043] -> w1654
          tunnel: [w2033 w2042] -> w1652
          tunnel: [w2032 w2041] -> w1650
          tunnel: [w2031 w2040] -> w1648
          tunnel: [w2030 w2039] -> w1646
          tunnel: [w2029 w2038] -> w1644
          tunnel: [w2028 w2037] -> w1630
          tunnel: [w2027 w2036] -> w1641
          tunnel: [w2026 w2035] -> w1628
          tunnel: w1655 -> [w2034 _]
          tunnel: w1653 -> [w2033 _]
          tunnel: w1651 -> [w2032 _]
          tunnel: w1649 -> [w2031 _]
          tunnel: w1647 -> [w2030 _]
          tunnel: w1645 -> [w2029 _]
          tunnel: w1643 -> [w2028 _]
          tunnel: w1642 -> [w2027 _]
          tunnel: w1640 -> [w2026 _]
          frame False {
          }
          frame True {
            n504 = String Subset(string=w2046, offset (0)=0, length (rest)=10 ("length (rest)")) -> (substring=w2049:string)
            n505 = String To Byte Array(string=w2049) -> (unsigned byte array=w2050:u8[])
            n506 = Array To Cluster(array=w2050) -> (cluster=w2044:T12)
            n507 = Unbundle By Name(w2044) -> ("unsigned byte array[0]"=w2043:u8, "unsigned byte array[1]"=w2042:u8, "unsigned byte array[2]"=w2041:u8, "unsigned byte array[3]"=w2040:u8, "unsigned byte array[4]"=w2039:u8, "unsigned byte array[5]"=w2038:u8, "unsigned byte array[6]"=w2037:u8, "unsigned byte array[7]"=w2036:u8, "unsigned byte array[8]"=w2035:u8)
            n508 = Build Array(w2043, w2042, w2041, w2040, w2039, w2038, w2037, w2036, w2035) -> (w2045:u8[])
            n509 = Number To Hexadecimal String(2:w2045) -> ()  [unwired: 1 in, 1 out]
          }
        }
        n510 = call "VOLTAGE READ-VI.vi"("unsigned byte array[7]"=w1513, "unsigned byte array[6]"=w1512, "unsigned byte array[5]"=w1511, "unsigned byte array[1]"=w1726, "unsigned byte array[8]"=w1514, "Numeric 8"=w1409, "Numeric 7"=w1408, "Numeric 9"=w1405, "Numeric 6"=w1407, "Numeric 5"=w1406, "Boolean"=w1730) -> ("Numeric 4"=w1365:dbl, "Numeric 3"=w1225:dbl, "Numeric 2"=w1216:dbl, "Numeric"=w1203:dbl, "Numeric 10"=w1198:dbl)
        "BATTERY VOLTAGE 1" <- w1365
        "batt-1 volt" <- w1365
        "BATTERY VOLTAGE 2" <- w1225
        "batt-2 volt" <- w1225
        "BATTERY VOLTAGE 3" <- w1216
        "batt-3 volt" <- w1216
        "BATTERY VOLTAGE 4" <- w1203
        "batt-4 volt" <- w1203
        "BATTERY VOLTAGE 5" <- w1198
        "batt-5 volt" <- w1198
        n511 = call "CURRENT READ-VI.vi"("unsigned byte array[7]"=w1513, "unsigned byte array[6]"=w1512, "unsigned byte array[5]"=w1511, "unsigned byte array[1]"=w1726, "unsigned byte array[8]"=w1514, "Numeric 4"=w1397, "Numeric 3"=w1396, "Numeric 5"=w1393, "Boolean"=w1727, "Numeric 2"=w1395, "Numeric"=w1394) -> ("Numeric 9"=w1392:dbl, "Numeric 8"=w1222:dbl, "Numeric 7"=w1214:dbl, "Numeric 6"=w1204:dbl, "Numeric 10"=w1195:dbl)
        "BATTERY CURRENT" <- w1392
        "BATT-1 CURRENT" <- w1392
        "BATTERY CURRENT 2" <- w1222
        "BATT-2 CURRENT" <- w1222
        "BATTERY CURRENT 3" <- w1214
        "BATT-3 CURRENT" <- w1214
        "BATTERY CURRENT 4" <- w1204
        "BATT-4 CURRENT" <- w1204
        "BATTERY CURRENT 5" <- w1195
        "BATT-5 CURRENT" <- w1195
        n512 = call "BATTERY FULL CAPACITY VI.vi"("unsigned byte array[7]"=w1513, "unsigned byte array[6]"=w1512, "unsigned byte array[5]"=w1511, "unsigned byte array[1]"=w1726, "unsigned byte array[8]"=w1514, "Numeric 4"=w1737, "Numeric 3"=w1729, "Numeric 5"=w1725, "Numeric 2"=w1736, "Numeric"=w1735, "Boolean"=w1744) -> ("Numeric 9"=w1411:dbl, "Numeric 8"=w1221:dbl, "Numeric 7"=w1215:dbl, "Numeric 6"=w1205:dbl, "Numeric 10"=w1196:dbl)
        "BATTERY FULL CAPACITY" <- w1411
        "BATT FCAP-1" <- w1411
        "BATTERY FULL CAPACITY 2" <- w1221
        "BATT FCAP-2" <- w1221
        "BATTERY FULL CAPACITY 3" <- w1215
        "BATT FCAP-3" <- w1215
        "BATTERY FULL CAPACITY 4" <- w1205
        "BATT FCAP-4" <- w1205
        "BATTERY FULL CAPACITY 5" <- w1196
        "BATT FCAP-5" <- w1196
        n513 = call "BATTERY REM-CAPACITY VI.vi"("unsigned byte array[7]"=w1513, "unsigned byte array[6]"=w1512, "unsigned byte array[5]"=w1511, "unsigned byte array[1]"=w1726, "unsigned byte array[8]"=w1514, "Numeric 9"=w1391, "Numeric 8"=w1390, "Numeric 10"=w1387, "Boolean"=w1742, "Numeric 7"=w1389, "Numeric 6"=w1388) -> ("Numeric 4"=w1386:dbl, "Numeric 3"=w1220:dbl, "Numeric 2"=w1212:dbl, "Numeric"=w1206:dbl, "Numeric 5"=w1194:dbl)
        "BATTERY REM CAPACITY" <- w1386
        "BATT-CAP-1" <- w1386
        "BATTERY REM CAPACITY 2" <- w1220
        "BATT-CAP-2" <- w1220
        "BATTERY REM CAPACITY 3" <- w1212
        "BATT-CAP-3" <- w1212
        "BATTERY REM CAPACITY 4" <- w1206
        "BATT-CAP-4" <- w1206
        "BATTERY REM CAPACITY 5" <- w1194
        "BATT-CAP-5" <- w1194
        n514 = call "BATTERY MAX ENERGY VI.vi"("unsigned byte array[7]"=w1513, "unsigned byte array[6]"=w1512, "unsigned byte array[5]"=w1511, "unsigned byte array[1]"=w1726, "unsigned byte array[8]"=w1514, "Numeric 9"=w1734, "Numeric 8"=w1733, "Numeric 10"=w1724, "Boolean"=w1738, "Numeric 7"=w1732, "Numeric 6"=w1731) -> ("Numeric 4"=w1412:dbl, "Numeric 3"=w1217:dbl, "Numeric 2"=w1211:dbl, "Numeric"=w1208:dbl, "Numeric 5"=w1193:dbl)
        "BATTERY MAX ENERGY" <- w1412
        "BATT-ENERGY-1" <- w1412
        "BATTERY MAX ENERGY 2" <- w1217
        "BATT-ENERGY-2" <- w1217
        "BATTERY MAX ENERGY 3" <- w1211
        "BATT-ENERGY-3" <- w1211
        "BATTERY MAX ENERGY 4" <- w1208
        "BATT-ENERGY-4" <- w1208
        "BATTERY MAX ENERGY 5" <- w1193
        "BATT-ENERGY-5" <- w1193
        n515 = call "BATTERY AVAILABLE ENERGY VI.vi"("unsigned byte array[7]"=w1513, "unsigned byte array[6]"=w1512, "unsigned byte array[5]"=w1511, "unsigned byte array[1]"=w1726, "unsigned byte array[8]"=w1514, "Numeric 4"=w1382, "Numeric 3"=w1381, "Numeric 5"=w1378, "Boolean"=w1740, "Numeric 2"=w1380, "Numeric"=w1379) -> ("Numeric 9"=w1377:dbl, "Numeric 8"=w1218:dbl, "Numeric 7"=w1213:dbl, "Numeric 6"=w1207:dbl, "Numeric 10"=w1192:dbl)
        "BATTERY AVAIL ENERGY" <- w1377
        "BATT-AVAIL-ENERGY-1" <- w1377
        "BATTERY AVAIL ENERGY 2" <- w1218
        "BATT-AVAIL-ENERGY-2" <- w1218
        "BATTERY AVAIL ENERGY 3" <- w1213
        "BATT-AVAIL-ENERGY-3" <- w1213
        "BATTERY AVAIL ENERGY 4" <- w1207
        "BATT-AVAIL-ENERGY-4" <- w1207
        "BATTERY AVAIL ENERGY 5" <- w1192
        "BATT-AVAIL-ENERGY-5" <- w1192
        n516 = Build Array "Battery"(w1365, w1225, w1216, w1203, w1198) -> (w1686:dbl[])
        n517 = String To Byte Array(string=w1705) -> (unsigned byte array=w1701:u8[])
        n518 = Flatten To JSON(anything=w1686) -> (JSON string=w1685:string)  [unwired: 2 in, 1 out]
        n519 = call-poly <vilib>:"POST.vi"("client handle"=w1690, "url"="Batter data send url", "buffer"=w1685, "error in (no error)"=w1689) -> ("client handle out"=w1713:T11, "error out"=w1712:errorcluster)  [unwired: 8 in, 2 out]
        n520 = Multiply(x=w1198, y=w1195) -> (x*y=w1197:dbl)
        "BATTERY POWER 5" <- w1197
        "POWER-5" <- w1197
        n521 = Multiply(x=w1365, y=w1392) -> (x*y=w1199:dbl)
        "BATTERY POWER" <- w1199
        "POWER-1" <- w1199
        n522 = Empty Array?(array=w1701) -> (empty?=w1702:bool)
        n523 = Multiply(x=w1203, y=w1204) -> (x*y=w1202:dbl)
        "BATTERY POWER 4" <- w1202
        "POWER-4" <- w1202
        n524 = Multiply(x=w1225, y=w1222) -> (x*y=w1200:dbl)
        "BATTERY POWER 2" <- w1200
        "POWER-2" <- w1200
        n525 = shared-variable "SBU-cRIO\\Variables for FPGA V4.lvlib\\Time"() -> (w1280:dbl)  [unwired: 1 in, 1 out]
        n526 = shared-variable "SBU-cRIO\\Variables for FPGA V4.lvlib\\Time"() -> (w1278:dbl)  [unwired: 1 in, 1 out]
        n527 = shared-variable "SBU-cRIO\\Variables for FPGA V4.lvlib\\Time"() -> (w1253:dbl)  [unwired: 1 in, 1 out]
        n528 = Multiply(x=w1216, y=w1214) -> (x*y=w1201:dbl)
        "BATTERY POWER 3" <- w1201
        "POWER-3" <- w1201
        n529 = shared-variable "SBU-cRIO\\Variables for FPGA V4.lvlib\\Time"() -> (w1281:dbl)  [unwired: 1 in, 1 out]
        n530 = shared-variable "SBU-cRIO\\Variables for FPGA V4.lvlib\\Time"() -> (w1226:dbl)  [unwired: 1 in, 1 out]
        n531 = Select(t=0.0 ("x"), s=w1702, f=48.0 ("x")) -> (s? t:f=w1698:dbl)
        n532 = call <vilib>:"AddHeader.vi"("client handle"=w1709, "header"="Content-Type", "error in (no error)"=w1708) -> ("client handle out"=w1692:T11, "error out"=w1691:errorcluster)  [unwired: 11 in]
        n533 = call <vilib>:"AddHeader.vi"("client handle"=w1713, "header"="Content-Type", "value"="application/json", "error in (no error)"=w1712) -> ("client handle out"=w1694:T11, "error out"=w1693:errorcluster)  [unwired: 10 in]
        n534 = Build Array (concatenate)(w1302, w1280) -> (w1279:dbl[])
        n535 = Build Array (concatenate)(w1277, w1278) -> (w1263:dbl[])
        n536 = Build Array (concatenate)(w1428, w1220) -> (w1290:dbl[])
        n537 = Build Array (concatenate)(w1427, w1212) -> (w1288:dbl[])
        n538 = Build Array (concatenate)(w1426, w1206) -> (w1286:dbl[])
        n539 = Build Array (concatenate)(w1425, w1194) -> (w1284:dbl[])
        n540 = Build Array (concatenate)(w1420, w1218) -> (w1260:dbl[])
        n541 = Build Array (concatenate)(w1421, w1213) -> (w1223:dbl[])
        n542 = Build Array (concatenate)(w1422, w1207) -> (w1257:dbl[])
        n543 = Build Array (concatenate)(w1423, w1192) -> (w1255:dbl[])
        n544 = Build Array (concatenate)(w1429, w1386) -> (w1292:dbl[])
        n545 = Build Array (concatenate)(w1419, w1377) -> (w1224:dbl[])
        n546 = Build Array (concatenate)(w1252, w1253) -> (w1238:dbl[])
        n547 = Index Array(array=w1701, index=2) -> (element=w1704:u8)
        n548 = Index Array(array=w1701, index=0) -> (element=w1703:u8)
        n549 = Build Array (concatenate)(w1462, w1226) -> (w1358:dbl[])
        n550 = Build Array (concatenate)(w1369, w1225) -> (w1355:dbl[])
        n551 = Build Array (concatenate)(w1368, w1216) -> (w1352:dbl[])
        n552 = Build Array (concatenate)(w1367, w1203) -> (w1350:dbl[])
        n553 = Build Array (concatenate)(w1366, w1198) -> (w1348:dbl[])
        n554 = Build Array (concatenate)(w1370, w1365) -> (w1356:dbl[])
        n555 = Build Array (concatenate)(w1430, w1197) -> (w1400:dbl[])
        n556 = Build Array (concatenate)(w1460, w1222) -> (w1315:dbl[])
        n557 = Build Array (concatenate)(w1459, w1214) -> (w1313:dbl[])
        n558 = Build Array (concatenate)(w1458, w1204) -> (w1311:dbl[])
        n559 = Build Array (concatenate)(w1457, w1195) -> (w1309:dbl[])
        n560 = Build Array (concatenate)(w1433, w1200) -> (w1403:dbl[])
        n561 = Build Array (concatenate)(w1432, w1201) -> (w1402:dbl[])
        n562 = Build Array (concatenate)(w1431, w1202) -> (w1401:dbl[])
        n563 = Build Array (concatenate)(w1461, w1392) -> (w1317:dbl[])
        n564 = Build Array (concatenate)(w1434, w1199) -> (w1404:dbl[])
        n565 = Build Array (concatenate)(w1328, w1281) -> (w1319:dbl[])
        n566 = Subtract(x=w1704, y=w1698) -> ()  [unwired: 1 out]
        n567 = Subtract(x=w1703, y=w1698) -> (x-y=w1697:dbl)
        "Power Button State" <- w1697
        n568 = Bundle(w1279, w1292) -> (w1307:cluster{dbl[], dbl[]})  [unwired: 1 in]
        n569 = Bundle(w1279, w1290) -> (w1306:cluster{dbl[], dbl[]})  [unwired: 1 in]
        n570 = Bundle(w1279, w1288) -> (w1305:cluster{dbl[], dbl[]})  [unwired: 1 in]
        n571 = Bundle(w1279, w1286) -> (w1304:cluster{dbl[], dbl[]})  [unwired: 1 in]
        n572 = Bundle(w1279, w1284) -> (w1303:cluster{dbl[], dbl[]})  [unwired: 1 in]
        n573 = Bundle(w1279, w1224) -> (w1276:cluster{dbl[], dbl[]})  [unwired: 1 in]
        n574 = Bundle(w1279, w1260) -> (w1275:cluster{dbl[], dbl[]})  [unwired: 1 in]
        n575 = Bundle(w1279, w1223) -> (w1274:cluster{dbl[], dbl[]})  [unwired: 1 in]
        n576 = Bundle(w1279, w1257) -> (w1273:cluster{dbl[], dbl[]})  [unwired: 1 in]
        n577 = Bundle(w1279, w1255) -> (w1272:cluster{dbl[], dbl[]})  [unwired: 1 in]
        n578 = Bundle(w1358, w1356) -> (w1364:cluster{dbl[], dbl[]})  [unwired: 1 in]
        n579 = Bundle(w1358, w1355) -> (w1363:cluster{dbl[], dbl[]})  [unwired: 1 in]
        n580 = Bundle(w1358, w1352) -> (w1362:cluster{dbl[], dbl[]})  [unwired: 1 in]
        n581 = Bundle(w1358, w1350) -> (w1361:cluster{dbl[], dbl[]})  [unwired: 1 in]
        n582 = Bundle(w1358, w1348) -> (w1360:cluster{dbl[], dbl[]})  [unwired: 1 in]
        n583 = Bundle(w1319, w1404) -> (w1333:cluster{dbl[], dbl[]})  [unwired: 1 in]
        n584 = Bundle(w1319, w1403) -> (w1332:cluster{dbl[], dbl[]})  [unwired: 1 in]
        n585 = Bundle(w1319, w1402) -> (w1331:cluster{dbl[], dbl[]})  [unwired: 1 in]
        n586 = Bundle(w1319, w1401) -> (w1330:cluster{dbl[], dbl[]})  [unwired: 1 in]
        n587 = Bundle(w1319, w1400) -> (w1329:cluster{dbl[], dbl[]})  [unwired: 1 in]
        n588 = Bundle(w1319, w1317) -> (w1338:cluster{dbl[], dbl[]})  [unwired: 1 in]
        n589 = Bundle(w1319, w1315) -> (w1337:cluster{dbl[], dbl[]})  [unwired: 1 in]
        n590 = Bundle(w1319, w1313) -> (w1336:cluster{dbl[], dbl[]})  [unwired: 1 in]
        n591 = Bundle(w1319, w1311) -> (w1335:cluster{dbl[], dbl[]})  [unwired: 1 in]
        n592 = Bundle(w1319, w1309) -> (w1334:cluster{dbl[], dbl[]})  [unwired: 1 in]
        n593 = Number To Boolean Array(number=w1697) -> (Boolean array=w1696:bool[])
        n594 = Build Array(w1621, w1620, w1619, w1618, w1617, w1616, w1593, w1615, w1594, w1614, w1592, w1591, w1613, w1612, w1611) -> ()  [unwired: 1 out]
        n595 = Build Array(w1654, w1652, w1650, w1648, w1646, w1644, w1630, w1641, w1628, w1638, w1626, w1625, w1634, w1632, w1631) -> ()  [unwired: 1 out]
        n596 = Build Array(w1555, w1554, w1553, w1552, w1551, w1550, w1521, w1549, w1522, w1548, w1520, w1519, w1547, w1546, w1545) -> ()  [unwired: 1 out]
        n597 = Build Array(w1495, w1494, w1493, w1492, w1491, w1490, w1484, w1489, w1482, w1488, w1481, w1480, w1487, w1486, w1485) -> ()  [unwired: 1 out]
        n598 = Build Array(w1587, w1586, w1585, w1584, w1583, w1582, w1573, w1581, w1574, w1580, w1572, w1571, w1579, w1578, w1577) -> ()  [unwired: 1 out]
        n599 = Equal?(x=w1482, y=u32 10) -> (x = y?=w1479:bool)
        n600 = Index Array(array=w1696, index=0) -> (element=w1684:bool)
        "Power Switch Led" <- w1684
        n601 = Build Array(w1276, w1275, w1274, w1273, w1272) -> (→"Battery Available Energy Plot":cluster{dbl[], dbl[]}[])
        n602 = shared-variable "SBU-cRIO\\Variables for FPGA V4.lvlib\\BATT-GATE 1"(w1684) -> ()  [unwired: 1 in, 1 out]
        n603 = Build Array(w1364, w1363, w1362, w1361, w1360) -> (→"Battery Voltage Discharge Plot":cluster{dbl[], dbl[]}[])
        n604 = Equal?(x=w1594, y=u32 10) -> (x = y?=w1596:bool)
        n605 = Equal?(x=w1522, y=u32 10) -> (x = y?=w1523:bool)
        n606 = Build Array(w1333, w1332, w1331, w1330, w1329) -> (→"Battery Power Plot":cluster{dbl[], dbl[]}[])
        n607 = Equal?(x=w1574, y=u32 10) -> (x = y?=w1576:bool)
        n608 = Build Array(w1338, w1337, w1336, w1335, w1334) -> (→"Battery Current Plot":cluster{dbl[], dbl[]}[])
        n609 = Build Array(w1307, w1306, w1305, w1304, w1303) -> (→"Battery Remaining Capacity Plot":cluster{dbl[], dbl[]}[])
        n610 = Equal?(x=w1628, y=u8 10) -> (x = y?=w1629:bool)
        n611 = shared-variable "SBU-cRIO\\Variables for FPGA V4.lvlib\\GATE-BATT-1"("BATT-GATE 1") -> ()  [unwired: 1 in, 1 out]
        n612 = shared-variable "SBU-cRIO\\Variables for FPGA V4.lvlib\\BATT-GATE 2"("BATT-GATE 5") -> ()  [unwired: 1 in, 1 out]
        n613 = shared-variable "SBU-cRIO\\Variables for FPGA V4.lvlib\\BATT-GATE 3"("BATT-GATE 3") -> ()  [unwired: 1 in, 1 out]
        n614 = shared-variable "SBU-cRIO\\Variables for FPGA V4.lvlib\\BATT-GATE 4"("BATT-GATE 4") -> ()  [unwired: 1 in, 1 out]
        n615 = shared-variable "SBU-cRIO\\Variables for FPGA V4.lvlib\\BATT-GATE 5"("BATT-GATE 2") -> ()  [unwired: 1 in, 1 out]
        n616 = case shown="True" w1523 {
          tunnel: w1521 -> [_ w1802]
          tunnel: w1520 -> [_ w1801]
          tunnel: w1519 -> [_ w1800]
          tunnel: [w1798 w1799] -> w1209
          tunnel: w1374 -> [w1798 _]
          frame False {
          }
          frame True {
            n617 = case shown="25, Default" w1802 {
              tunnel: w1801 -> [w1805]
              tunnel: w1800 -> [w1804]
              tunnel: [w1803] -> w1799
              frame 25, Default {
                n618 = Build Array(w1805, w1804) -> (w1806:u8[])
                n619 = Byte Array To String(unsigned byte array=w1806) -> (string=w1811:string)
                n620 = Reverse String(1:w1811) -> (0:w1810:string)
                n621 = Type Cast(type=i16 0, x=w1810) -> (*(type *) &x=w1807:i16)
                n622 = Multiply(x=w1807, y=0.1) -> (x*y=w1803:dbl)
              }
            }
          }
        }
        "Batt-temp-4" <- w1209
        "BATT-TEMP 4" <- w1209
        n623 = Build Array (concatenate)(w1415, w1209) -> (w1230:dbl[])
        n624 = Bundle(w1238, w1230) -> (w1248:cluster{dbl[], dbl[]})  [unwired: 1 in]
        n625 = case shown="True" w1576 {
          tunnel: w1573 -> [_ w1859]
          tunnel: w1572 -> [_ w1858]
          tunnel: w1571 -> [_ w1857]
          tunnel: [w1855 w1856] -> w1210
          tunnel: w1372 -> [w1855 _]
          frame False {
          }
          frame True {
            n626 = case shown="24, Default" w1859 {
              tunnel: w1858 -> [w1862]
              tunnel: w1857 -> [w1861]
              tunnel: [w1860] -> w1856
              frame 24, Default {
                n627 = Build Array(w1862, w1861) -> (w1863:u8[])
                n628 = Byte Array To String(unsigned byte array=w1863) -> (string=w1868:string)
                n629 = Reverse String(1:w1868) -> (0:w1867:string)
                n630 = Type Cast(type=i16 0, x=w1867) -> (*(type *) &x=w1864:i16)
                n631 = Multiply(x=w1864, y=0.1) -> (x*y=w1860:dbl)
              }
            }
          }
        }
        "Batt-temp-3" <- w1210
        "BATT-TEMP 3" <- w1210
        n632 = Build Array (concatenate)(w1416, w1210) -> (w1232:dbl[])
        n633 = Bundle(w1238, w1232) -> (w1249:cluster{dbl[], dbl[]})  [unwired: 1 in]
        n634 = case shown="True" w1479 {
          tunnel: w1484 -> [_ w1766]
          tunnel: w1481 -> [_ w1765]
          tunnel: w1480 -> [_ w1764]
          tunnel: [w1762 w1763] -> w1191
          tunnel: w1375 -> [w1762 _]
          frame False {
          }
          frame True {
            n635 = case shown="26, Default" w1766 {
              tunnel: w1765 -> [w1769]
              tunnel: w1764 -> [w1768]
              tunnel: [w1767] -> w1763
              frame 26, Default {
                n636 = Build Array(w1769, w1768) -> (w1770:u8[])
                n637 = Byte Array To String(unsigned byte array=w1770) -> (string=w1775:string)
                n638 = Reverse String(1:w1775) -> (0:w1774:string)
                n639 = Type Cast(type=i16 0, x=w1774) -> (*(type *) &x=w1771:i16)
                n640 = Multiply(x=w1771, y=0.1) -> (x*y=w1767:dbl)
              }
            }
          }
        }
        "Batt-temp-5" <- w1191
        "BATT-TEMP 5" <- w1191
        n641 = Build Array (concatenate)(w1414, w1191) -> (w1228:dbl[])
        n642 = Bundle(w1238, w1228) -> (w1247:cluster{dbl[], dbl[]})  [unwired: 1 in]
        n643 = case shown="True" w1596 {
          tunnel: w1593 -> [_ w1916]
          tunnel: w1592 -> [_ w1915]
          tunnel: w1591 -> [_ w1914]
          tunnel: [w1912 w1913] -> w1219
          tunnel: w1373 -> [w1912 _]
          frame False {
          }
          frame True {
            n644 = case shown="23, Default" w1916 {
              tunnel: w1915 -> [w1919]
              tunnel: w1914 -> [w1918]
              tunnel: [w1917] -> w1913
              frame 23, Default {
                n645 = Build Array(w1919, w1918) -> (w1920:u8[])
                n646 = Byte Array To String(unsigned byte array=w1920) -> (string=w1925:string)
                n647 = Reverse String(1:w1925) -> (0:w1924:string)
                n648 = Type Cast(type=i16 0, x=w1924) -> (*(type *) &x=w1921:i16)
                n649 = Multiply(x=w1921, y=0.1) -> (x*y=w1917:dbl)
              }
            }
          }
        }
        "Batt-temp-2" <- w1219
        "BATT-TEMP 2" <- w1219
        n650 = Build Array (concatenate)(w1417, w1219) -> (w1234:dbl[])
        n651 = Bundle(w1238, w1234) -> (w1250:cluster{dbl[], dbl[]})  [unwired: 1 in]
        n652 = case shown="True" w1629 {
          tunnel: w1630 -> [_ w1974]
          tunnel: w1626 -> [_ w1973]
          tunnel: w1625 -> [_ w1972]
          tunnel: [w1969 w1971] -> w1376
          tunnel: w1371 -> [w1969 w1970]
          frame False {
          }
          frame True {
            n653 = case shown="22, Default" w1974 {
              tunnel: w1973 -> [w1977]
              tunnel: w1972 -> [w1976]
              tunnel: [w1975] -> w1971
              tunnel: w1970 -> [_]
              frame 22, Default {
                n654 = Build Array(w1977, w1976) -> (w1978:u8[])
                n655 = Byte Array To String(unsigned byte array=w1978) -> (string=w1983:string)
                n656 = Reverse String(1:w1983) -> (0:w1982:string)
                n657 = Type Cast(type=i16 0, x=w1982) -> (*(type *) &x=w1979:i16)
                n658 = Multiply(x=w1979, y=0.1) -> (x*y=w1975:dbl)
              }
            }
          }
        }
        "BATT-TEMP" <- w1376
        "Batt-temp-1" <- w1376
        n659 = Build Array (concatenate)(w1418, w1376) -> (w1236:dbl[])
        n660 = Bundle(w1238, w1236) -> (w1251:cluster{dbl[], dbl[]})  [unwired: 1 in]
        n661 = Build Array(w1251, w1250, w1249, w1248, w1247) -> (→"Battery temp plot":cluster{dbl[], dbl[]}[])
        n662 = shared-variable "SBU-cRIO\\Variables for FPGA V4.lvlib\\LO1-REL 1"("Load-1") -> ()  [unwired: 1 in, 1 out]
        n663 = shared-variable "SBU-cRIO\\Variables for FPGA V4.lvlib\\LO1-REL 2"("Load-1") -> ()  [unwired: 1 in, 1 out]
        n664 = shared-variable "SBU-cRIO\\Variables for FPGA V4.lvlib\\LO2-REL 1"("Load-2") -> ()  [unwired: 1 in, 1 out]
        n665 = shared-variable "SBU-cRIO\\Variables for FPGA V4.lvlib\\LO2-REL 2"("Load-2") -> ()  [unwired: 1 in, 1 out]
        n666 = shared-variable "SBU-cRIO\\Variables for FPGA V4.lvlib\\SUPCAP-GATE 6"("SUPERCAP-GATE 6") -> ()  [unwired: 1 in, 1 out]
        n667 = feedback #7() -> (w1339:bool)  [unwired: 1 in]
        n668 = call "RyanRemove.vi"("Boolean"=w1339, "IN"=w1358) -> ("OUT"=w1357:dbl[])  [unwired: 9 in]
        n669 = call "RyanRemove.vi"("Boolean"=w1339, "IN"=w1356) -> ("OUT"=w1354:dbl[])  [unwired: 9 in]
        n670 = call "RyanTestComp.vi"("NEW"=w1356, "OLD"=w1354) -> ("Boolean"=w1342:bool)  [unwired: 9 in]
        n671 = call "RyanRemove.vi"("Boolean"=w1339, "IN"=w1355) -> ("OUT"=w1353:dbl[])  [unwired: 9 in]
        n672 = call "RyanTestComp.vi"("NEW"=w1353, "OLD"=w1355) -> ("Boolean"=w1343:bool)  [unwired: 9 in]
        n673 = call "RyanRemove.vi"("Boolean"=w1339, "IN"=w1352) -> ("OUT"=w1351:dbl[])  [unwired: 9 in]
        n674 = call "RyanTestComp.vi"("NEW"=w1351, "OLD"=w1352) -> ("Boolean"=w1344:bool)  [unwired: 9 in]
        n675 = call "RyanRemove.vi"("Boolean"=w1339, "IN"=w1350) -> ("OUT"=w1349:dbl[])  [unwired: 9 in]
        n676 = call "RyanTestComp.vi"("NEW"=w1349, "OLD"=w1350) -> ("Boolean"=w1345:bool)  [unwired: 9 in]
        n677 = call "RyanRemove.vi"("Boolean"=w1339, "IN"=w1348) -> ("OUT"=w1347:dbl[])  [unwired: 9 in]
        n678 = call "RyanTestComp.vi"("NEW"=w1347, "OLD"=w1348) -> ("Boolean"=w1346:bool)  [unwired: 9 in]
        n679 = Build Array(w1342, w1343, w1344, w1345, w1346) -> (w1341:bool[])
        n680 = feedback #8() -> (w1320:bool)  [unwired: 1 in]
        n681 = call "RyanRemove.vi"("Boolean"=w1320, "IN"=w1319) -> ("OUT"=w1318:dbl[])  [unwired: 9 in]
        n682 = call "RyanRemove.vi"("Boolean"=w1320, "IN"=w1317) -> ("OUT"=w1316:dbl[])  [unwired: 9 in]
        n683 = call "RyanTestComp.vi"("NEW"=w1316, "OLD"=w1317) -> ("Boolean"=w1326:bool)  [unwired: 9 in]
        n684 = call "RyanRemove.vi"("Boolean"=w1320, "IN"=w1315) -> ("OUT"=w1314:dbl[])  [unwired: 9 in]
        n685 = call "RyanTestComp.vi"("NEW"=w1314, "OLD"=w1315) -> ("Boolean"=w1325:bool)  [unwired: 9 in]
        n686 = call "RyanRemove.vi"("Boolean"=w1320, "IN"=w1313) -> ("OUT"=w1312:dbl[])  [unwired: 9 in]
        n687 = call "RyanTestComp.vi"("NEW"=w1312, "OLD"=w1313) -> ("Boolean"=w1324:bool)  [unwired: 9 in]
        n688 = call "RyanRemove.vi"("Boolean"=w1320, "IN"=w1311) -> ("OUT"=w1310:dbl[])  [unwired: 9 in]
        n689 = call "RyanTestComp.vi"("NEW"=w1310, "OLD"=w1311) -> ("Boolean"=w1323:bool)  [unwired: 9 in]
        n690 = call "RyanRemove.vi"("Boolean"=w1320, "IN"=w1309) -> ("OUT"=w1308:dbl[])  [unwired: 9 in]
        n691 = call "RyanTestComp.vi"("NEW"=w1308, "OLD"=w1309) -> ("Boolean"=w1322:bool)  [unwired: 9 in]
        n692 = Build Array(w1326, w1325, w1324, w1323, w1322) -> (w1327:bool[])
        n693 = feedback #9() -> (w1294:bool)  [unwired: 1 in]
        n694 = call "RyanRemove.vi"("Boolean"=w1294, "IN"=w1279) -> ("OUT"=w1293:dbl[])  [unwired: 9 in]
        n695 = call "RyanRemove.vi"("Boolean"=w1294, "IN"=w1292) -> ("OUT"=w1291:dbl[])  [unwired: 9 in]
        n696 = call "RyanTestComp.vi"("NEW"=w1291, "OLD"=w1292) -> ("Boolean"=w1300:bool)  [unwired: 9 in]
        n697 = call "RyanRemove.vi"("Boolean"=w1294, "IN"=w1290) -> ("OUT"=w1289:dbl[])  [unwired: 9 in]
        n698 = call "RyanTestComp.vi"("NEW"=w1289, "OLD"=w1290) -> ("Boolean"=w1299:bool)  [unwired: 9 in]
        n699 = call "RyanRemove.vi"("Boolean"=w1294, "IN"=w1288) -> ("OUT"=w1287:dbl[])  [unwired: 9 in]
        n700 = call "RyanTestComp.vi"("NEW"=w1287, "OLD"=w1288) -> ("Boolean"=w1298:bool)  [unwired: 9 in]
        n701 = call "RyanRemove.vi"("Boolean"=w1294, "IN"=w1286) -> ("OUT"=w1285:dbl[])  [unwired: 9 in]
        n702 = call "RyanTestComp.vi"("NEW"=w1285, "OLD"=w1286) -> ("Boolean"=w1297:bool)  [unwired: 9 in]
        n703 = call "RyanRemove.vi"("Boolean"=w1294, "IN"=w1284) -> ("OUT"=w1283:dbl[])  [unwired: 9 in]
        n704 = call "RyanTestComp.vi"("NEW"=w1283, "OLD"=w1284) -> ("Boolean"=w1296:bool)  [unwired: 9 in]
        n705 = Build Array(w1300, w1299, w1298, w1297, w1296) -> (w1301:bool[])
        n706 = Or Array Elements(Boolean array=w1341) -> (logical OR=w1340:bool)
        n707 = feedback-in #7(w1340) -> ()
        n708 = Or Array Elements(Boolean array=w1327) -> (logical OR=w1321:bool)
        n709 = feedback-in #8(w1321) -> ()
        n710 = feedback #10() -> (w1264:bool)  [unwired: 1 in]
        n711 = call "RyanRemove.vi"("Boolean"=w1264, "IN"=w1263) -> ("OUT"=w1262:dbl[])  [unwired: 9 in]
        n712 = call "RyanRemove.vi"("Boolean"=w1264, "IN"=w1224) -> ("OUT"=w1261:dbl[])  [unwired: 9 in]
        n713 = call "RyanTestComp.vi"("NEW"=w1261, "OLD"=w1224) -> ("Boolean"=w1270:bool)  [unwired: 9 in]
        n714 = call "RyanRemove.vi"("Boolean"=w1264, "IN"=w1260) -> ("OUT"=w1259:dbl[])  [unwired: 9 in]
        n715 = call "RyanTestComp.vi"("NEW"=w1259, "OLD"=w1260) -> ("Boolean"=w1269:bool)  [unwired: 9 in]
        n716 = call "RyanRemove.vi"("Boolean"=w1264, "IN"=w1223) -> ("OUT"=w1258:dbl[])  [unwired: 9 in]
        n717 = call "RyanTestComp.vi"("NEW"=w1258, "OLD"=w1223) -> ("Boolean"=w1268:bool)  [unwired: 9 in]
        n718 = call "RyanRemove.vi"("Boolean"=w1264, "IN"=w1257) -> ("OUT"=w1256:dbl[])  [unwired: 9 in]
        n719 = call "RyanTestComp.vi"("NEW"=w1256, "OLD"=w1257) -> ("Boolean"=w1267:bool)  [unwired: 9 in]
        n720 = call "RyanRemove.vi"("Boolean"=w1264, "IN"=w1255) -> ("OUT"=w1254:dbl[])  [unwired: 9 in]
        n721 = call "RyanTestComp.vi"("NEW"=w1254, "OLD"=w1255) -> ("Boolean"=w1266:bool)  [unwired: 9 in]
        n722 = Build Array(w1270, w1269, w1268, w1267, w1266) -> (w1271:bool[])
        n723 = Or Array Elements(Boolean array=w1301) -> (logical OR=w1295:bool)
        n724 = feedback-in #9(w1295) -> ()
        n725 = Or Array Elements(Boolean array=w1271) -> (logical OR=w1265:bool)
        n726 = feedback-in #10(w1265) -> ()
        n727 = feedback #11() -> (w1239:bool)  [unwired: 1 in]
        n728 = call "RyanRemove.vi"("Boolean"=w1239, "IN"=w1238) -> ("OUT"=w1237:dbl[])  [unwired: 9 in]
        n729 = call "RyanRemove.vi"("Boolean"=w1239, "IN"=w1236) -> ("OUT"=w1235:dbl[])  [unwired: 9 in]
        n730 = call "RyanTestComp.vi"("NEW"=w1235, "OLD"=w1236) -> ("Boolean"=w1245:bool)  [unwired: 9 in]
        n731 = call "RyanRemove.vi"("Boolean"=w1239, "IN"=w1234) -> ("OUT"=w1233:dbl[])  [unwired: 9 in]
        n732 = call "RyanTestComp.vi"("NEW"=w1233, "OLD"=w1234) -> ("Boolean"=w1244:bool)  [unwired: 9 in]
        n733 = call "RyanRemove.vi"("Boolean"=w1239, "IN"=w1232) -> ("OUT"=w1231:dbl[])  [unwired: 9 in]
        n734 = call "RyanTestComp.vi"("NEW"=w1231, "OLD"=w1232) -> ("Boolean"=w1243:bool)  [unwired: 9 in]
        n735 = call "RyanRemove.vi"("Boolean"=w1239, "IN"=w1230) -> ("OUT"=w1229:dbl[])  [unwired: 9 in]
        n736 = call "RyanTestComp.vi"("NEW"=w1229, "OLD"=w1230) -> ("Boolean"=w1242:bool)  [unwired: 9 in]
        n737 = call "RyanRemove.vi"("Boolean"=w1239, "IN"=w1228) -> ("OUT"=w1227:dbl[])  [unwired: 9 in]
        n738 = call "RyanTestComp.vi"("NEW"=w1227, "OLD"=w1228) -> ("Boolean"=w1241:bool)  [unwired: 9 in]
        n739 = Build Array(w1245, w1244, w1243, w1242, w1241) -> (w1246:bool[])
        n740 = Or Array Elements(Boolean array=w1246) -> (logical OR=w1240:bool)
        n741 = feedback-in #11(w1240) -> ()
      }
      n742 = node-c288(i64 25 ("Period")) -> (w170:T8)  [unwired: 3 in]
      n743 = timed-loop "Timed loop" {
        timing: w170 -> [_]
        timing-out: [_] -> w169
        border: w165 -> [_]
        border: w165 -> [_]
        border: w165 -> [_]
        border: w165 -> [_]
        border: w165 -> [_]
        border: w165 -> [_]
        border: 0.0 -> [_]
        border: w165 -> [_]
        border: w165 -> [_]
        border: w165 -> [_]
        border: w165 -> [_]
        border: w165 -> [_]
        border: w165 -> [_]
        border: w165 -> [_]
        border: w165 -> [_]
        border: w165 -> [_]
        border: w165 -> [_]
        border: w165 -> [_]
        border: w165 -> [_]
        border: w165 -> [_]
        border: w165 -> [_]
        border: w165 -> [_]
        border: w165 -> [_]
        border: w165 -> [_]
        border: w165 -> [_]
        border: w165 -> [_]
        border: w165 -> [_]
        border: w165 -> [_]
        border: w165 -> [_]
        border: w165 -> [_]
        border: w165 -> [_]
        border: w165 -> [_]
        border: w165 -> [_]
        border: w165 -> [_]
        border: w165 -> [_]
        border: w165 -> [_]
        border: w165 -> [_]
        shift-right: [w2214] -> _
        shift-left: w165 -> [w2213]
        shift-right: [w2209] -> _
        shift-left: w165 -> [w2208]
        shift-right: [w2206] -> _
        shift-left: w165 -> [w2207]
        shift-right: [w2204] -> _
        shift-left: w165 -> [w2205]
        shift-right: [w2203] -> _
        shift-left: w165 -> [w2202]
        shift-right: [w2201] -> _
        shift-left: w165 -> [w2200]
        shift-right: [w2182] -> _
        shift-left: w165 -> [w2181]
        shift-right: [w2059] -> _
        shift-left: dbl[] [] -> [w2185]
        shift-right: [w2162] -> _
        shift-left: dbl[] [] -> [w2179]
        shift-right: [w2161] -> _
        shift-left: dbl[] [] -> [w2173]
        shift-right: [w2160] -> _
        shift-left: dbl[] [] -> [w2172]
        shift-right: [w2159] -> _
        shift-left: dbl[] [] -> [w2171]
        shift-right: [w2158] -> _
        shift-left: dbl[] [] -> [w2170]
        shift-right: [w2157] -> _
        shift-left: dbl[] [] -> [w2169]
        shift-right: [w2135] -> _
        shift-left: dbl[] [] -> [w2141]
        shift-right: [w2134] -> _
        shift-left: dbl[] [] -> [w2140]
        shift-right: [w2138] -> _
        shift-left: dbl[] [] -> [w2144]
        shift-right: [w2137] -> _
        shift-left: dbl[] [] -> [w2143]
        shift-right: [w2136] -> _
        shift-left: dbl[] [] -> [w2142]
        shift-right: [w2133] -> _
        shift-left: dbl[] [] -> [w2139]
        shift-right: [w2120] -> _
        shift-left: dbl[] [] -> [w2126]
        shift-right: [w2119] -> _
        shift-left: dbl[] [] -> [w2125]
        shift-right: [w2118] -> _
        shift-left: dbl[] [] -> [w2124]
        shift-right: [w2117] -> _
        shift-left: dbl[] [] -> [w2123]
        shift-right: [w2116] -> _
        shift-left: dbl[] [] -> [w2122]
        shift-right: [w2115] -> _
        shift-left: dbl[] [] -> [w2121]
        shift-right: [w2090] -> _
        shift-left: dbl[] [] -> [w2102]
        shift-right: [w2089] -> _
        shift-left: dbl[] [] -> [w2101]
        shift-right: [w2088] -> _
        shift-left: dbl[] [] -> [w2100]
        shift-right: [w2091] -> _
        shift-left: dbl[] [] -> [w2103]
        shift-right: [w2087] -> _
        shift-left: dbl[] [] -> [w2099]
        shift-right: [w2086] -> _
        shift-left: dbl[] [] -> [w2098]
        shift-right: [w2064] -> _
        shift-left: w116 -> [w2081]
        shift-right: [w2063] -> _
        shift-left: w116 -> [w2080]
        shift-right: [w2062] -> _
        shift-left: w116 -> [w2079]
        shift-right: [w2061] -> _
        shift-left: w116 -> [w2078]
        shift-right: [w2060] -> _
        shift-left: w116 -> [w2076]
        shift-right: [w2069] -> _
        shift-left: dbl[] [] -> [w2070]
        shift-right: [w2054] -> _
        shift-left: dbl[] [] -> [w2068]
        shift-right: [w2053] -> _
        shift-left: dbl[] [] -> [w2067]
        shift-right: [w2052] -> _
        shift-left: dbl[] [] -> [w2066]
        shift-right: [w2051] -> _
        shift-left: dbl[] [] -> [w2065]
        stop <- "Stop RT" stop-if-true
        w2077 = 36.7 ("Count per volt")
        w2183 = 0.025 ("Time Target (s)")
        # "Module 1"
        # "Module 2"
        # "Module 3"
        # "Module 4"
        # "Module 5"
        # "M2T6"
        # "M2T5"
        # "M2T4"
        # "M2T3"
        # "M2T2"
        # "M2T1"
        # "M1T6"
        # "M1T5"
        # "M1T4"
        # "M1T3"
        # "M1T2"
        # "M1T1"
        # "M1T1"
        # "Time"
        n744 = node-c288() -> ()  [unwired: 1 in, 1 out]
        n745 = shared-variable "SBU-cRIO\\Variables for FPGA V4.lvlib\\Recent Receive"() -> (w2273:T7)  [unwired: 1 in, 1 out]
        n746 = shared-variable "SBU-cRIO\\Variables for FPGA V4.lvlib\\ContModeCap"("Continuous Measurement") -> ()  [unwired: 1 in, 1 out]
        n747 = Unbundle By Name(w2273) -> ("identifier"=w2216:u32, "data"=w2272:u8[])  [unwired: 6 out]
        n748 = shared-variable "SBU-cRIO\\Variables for FPGA V4.lvlib\\Total Received"() -> (→"Total Received":u32)  [unwired: 1 in, 1 out]
        n749 = shared-variable "SBU-cRIO\\Variables for FPGA V4.lvlib\\Stop RT"("Stop RT") -> ()  [unwired: 1 in, 1 out]
        n750 = shared-variable "SBU-cRIO\\Variables for FPGA V4.lvlib\\Turn on SW1"("?") -> ()  [unwired: 1 in, 1 out]
        n751 = Array To Cluster(array=w2272) -> (cluster=w2275:T13)
        n752 = feedback #12() -> (w2279:dbl)
        n753 = Increment(x=w2279) -> (x+1=w2278:dbl)
        n754 = Greater?(x=13.0, y=w2278) -> (0:w2280:bool)
        n755 = Select(t=w2278, s=w2280, f=0.0 ("t")) -> (s? t:f=w2212:dbl)
        "Counter Register" <- w2212
        n756 = case shown="True" "Continuous Measurement" {
          tunnel: "Transmit Frame" -> [w2468 w2473]
          tunnel: [w2468 w2472] -> w2282
          tunnel: w2212 -> [_ w2471]
          tunnel: TRUE -> [w2467 w2470]
          tunnel: [w2467 w2469] -> w2276
          frame False {
          }
          frame True {
            n757 = case shown="1, Default" w2471 {
              tunnel: w2473 -> [w2476 w2483 w2488 w2493 w2498 w2503 w2508 w2513 w2518 w2523 w2528 w2533]
              tunnel: [w2475 w2482 w2487 w2492 w2497 w2502 w2507 w2512 w2517 w2522 w2527 w2532] -> w2472
              tunnel: w2470 -> [w2474 w2479 w2484 w2489 w2494 w2499 w2504 w2509 w2514 w2519 w2524 w2529]
              tunnel: [w2474 w2479 w2484 w2489 w2494 w2499 w2504 w2509 w2514 w2519 w2524 w2529] -> w2469
              frame 1, Default {
                n758 = call "ReadModule.vi"("Transmit Frame in"=w2476, "Numeric"=8, "Numeric 2"=1) -> ("Transmit Frame out"=w2475:T7)  [unwired: 8 in]
              }
              frame 2 {
                n759 = call "ReadModule.vi"("Transmit Frame in"=w2483, "Numeric"=8, "Numeric 2"=2) -> ("Transmit Frame out"=w2482:T7)  [unwired: 8 in]
              }
              frame 3 {
                n760 = call "ReadModule.vi"("Transmit Frame in"=w2488, "Numeric"=8, "Numeric 2"=3) -> ("Transmit Frame out"=w2487:T7)  [unwired: 8 in]
              }
              frame 4 {
                n761 = call "ReadModule.vi"("Transmit Frame in"=w2493, "Numeric"=8, "Numeric 2"=4) -> ("Transmit Frame out"=w2492:T7)  [unwired: 8 in]
              }
              frame 5 {
                n762 = call "ReadModule.vi"("Transmit Frame in"=w2498, "Numeric"=8, "Numeric 2"=5) -> ("Transmit Frame out"=w2497:T7)  [unwired: 8 in]
              }
              frame 6 {
                n763 = call "ReadModule.vi"("Transmit Frame in"=w2503, "Numeric"=8, "Numeric 2"=6) -> ("Transmit Frame out"=w2502:T7)  [unwired: 8 in]
              }
              frame 7 {
                n764 = call "ReadModule.vi"("Transmit Frame in"=w2508, "Numeric"=1, "Numeric 2"=1) -> ("Transmit Frame out"=w2507:T7)  [unwired: 8 in]
              }
              frame 8 {
                n765 = call "ReadModule.vi"("Transmit Frame in"=w2513, "Numeric"=1, "Numeric 2"=2) -> ("Transmit Frame out"=w2512:T7)  [unwired: 8 in]
              }
              frame 9 {
                n766 = call "ReadModule.vi"("Transmit Frame in"=w2518, "Numeric"=1, "Numeric 2"=3) -> ("Transmit Frame out"=w2517:T7)  [unwired: 8 in]
              }
              frame 10 {
                n767 = call "ReadModule.vi"("Transmit Frame in"=w2523, "Numeric"=1, "Numeric 2"=4) -> ("Transmit Frame out"=w2522:T7)  [unwired: 8 in]
              }
              frame 11 {
                n768 = call "ReadModule.vi"("Transmit Frame in"=w2528, "Numeric"=1, "Numeric 2"=5) -> ("Transmit Frame out"=w2527:T7)  [unwired: 8 in]
              }
              frame 12 {
                n769 = call "ReadModule.vi"("Transmit Frame in"=w2533, "Numeric"=1, "Numeric 2"=6) -> ("Transmit Frame out"=w2532:T7)  [unwired: 8 in]
              }
            }
          }
        }
        n770 = feedback-in #12(w2212) -> ()
        n771 = Unbundle By Name(w2275) -> ("data[0]"=w2085:u8, "data[2]"=w2084:u8, "data[3]"=w2083:u8, "data[4]"=w2239:u8, "data[5]"=w2215:u8, "data[6]"=w2238:u8, "data[7]"=w2237:u8)  [unwired: 1 out]
        n772 = Equal?(x=u32 273, y=w2216) -> (x = y?=w2082:bool)
        n773 = Equal?(x=u32 1297, y=w2216) -> (x = y?=w2236:bool)
        n774 = Equal?(x=w2216, y=u32 1041) -> (x = y?=w2235:bool)
        n775 = Equal?(x=w2085, y=u8 1) -> (x = y?=w2250:bool)
        "MOD 1" <- w2250
        n776 = Equal?(x=w2085, y=u8 3) -> (x = y?=w2248:bool)
        "MOD 3" <- w2248
        n777 = Equal?(x=w2085, y=u8 4) -> (x = y?=w2240:bool)
        "MOD 4" <- w2240
        n778 = Equal?(x=w2085, y=u8 5) -> (x = y?=w2220:bool)
        "MOD 5" <- w2220
        n779 = Equal?(x=w2085, y=u8 6) -> (x = y?=w2219:bool)
        "MOD 6" <- w2219
        n780 = Equal?(x=w2085, y=u8 2) -> (x = y?=w2249:bool)
        "MOD 2" <- w2249
        n781 = shared-variable "SBU-cRIO\\Variables for FPGA V4.lvlib\\Transmit Frame"(w2282) -> ()  [unwired: 1 in, 1 out]
        n782 = shared-variable "SBU-cRIO\\Variables for FPGA V4.lvlib\\Transmit"(w2276) -> ()  [unwired: 1 in, 1 out]
        n783 = feedback #13() -> (w2269:dbl)
        n784 = feedback #14() -> (w2268:dbl)
        n785 = feedback #15() -> (w2270:dbl)
        n786 = feedback #16() -> (w2267:dbl)
        n787 = feedback #17() -> (w2266:dbl)
        n788 = feedback #18() -> (w2265:dbl)
        n789 = feedback #19() -> (w2258:dbl)
        n790 = feedback #20() -> (w2259:dbl)
        n791 = feedback #21() -> (w2260:dbl)
        n792 = call "CAP-MOD-1.vi"("Boolean 3"=w2250, "data[2]"=w2084, "Numeric 7"=w2265, "data[3]"=w2083, "data[4]"=w2239, "data[5]"=w2215, "data[6]"=w2238, "Boolean"=w2235, "data[7]"=w2237, "Boolean 2"=w2236, "Count per volt"=w2077, "Numeric 10"=w2268, "Numeric 9"=w2267, "Numeric 11"=w2269, "Numeric 8"=w2266, "Numeric 12"=w2270) -> ("Numeric 5"=w2178:dbl, "Numeric 4"=w2177:dbl, "Numeric 6"=w2180:dbl, "Numeric"=w2174:dbl, "Numeric 3"=w2176:dbl, "Numeric 2"=w2175:dbl)  [unwired: 6 in]
        "TAP 1_1" <- w2180
        "TAP 1_2" <- w2178
        "TAP 1_3" <- w2177
        "TAP 1_4" <- w2176
        "TAP 1_5" <- w2175
        "TAP 1_6" <- w2174
        n793 = feedback-in #13(w2178) -> ()
        n794 = feedback-in #14(w2177) -> ()
        n795 = feedback-in #15(w2180) -> ()
        n796 = feedback-in #16(w2176) -> ()
        n797 = feedback-in #17(w2175) -> ()
        n798 = feedback-in #18(w2174) -> ()
        n799 = feedback #22() -> (w2263:dbl)
        n800 = feedback #23() -> (w2262:dbl)
        n801 = feedback #24() -> (w2261:dbl)
        n802 = call "CAP-MOD-4.vi"("Count per volt"=w2077, "Boolean 3"=w2249, "Numeric 10"=w2261, "data[2]"=w2084, "data[3]"=w2083, "data[4]"=w2239, "data[5]"=w2215, "Boolean"=w2235, "data[6]"=w2238, "Boolean 2"=w2236, "data[7]"=w2237, "Numeric 9"=w2260, "Numeric 12"=w2263, "Numeric 8"=w2259, "Numeric 11"=w2262, "Numeric 7"=w2258) -> ("Numeric 4"=w2154:dbl, "Numeric 5"=w2155:dbl, "Numeric 6"=w2156:dbl, "Numeric 3"=w2153:dbl, "Numeric"=w2151:dbl, "Numeric 2"=w2152:dbl)  [unwired: 6 in]
        "TAP 2_1" <- w2156
        "TAP 2_2" <- w2155
        "TAP 2_3" <- w2154
        "TAP 2_4" <- w2153
        "TAP 2_5" <- w2152
        "TAP 2_6" <- w2151
        n803 = feedback-in #19(w2156) -> ()
        n804 = feedback-in #20(w2155) -> ()
        n805 = feedback-in #21(w2154) -> ()
        n806 = feedback-in #22(w2153) -> ()
        n807 = feedback-in #23(w2152) -> ()
        n808 = feedback-in #24(w2151) -> ()
        n809 = feedback #25() -> (w2254:dbl)
        n810 = feedback #26() -> (w2256:dbl)
        n811 = feedback #27() -> (w2255:dbl)
        n812 = feedback #28() -> (w2253:dbl)
        n813 = feedback #29() -> (w2251:dbl)
        n814 = feedback #30() -> (w2252:dbl)
        n815 = call "CAP-M0D3.vi"("data[2]"=w2084, "data[3]"=w2083, "Numeric 8"=w2252, "data[4]"=w2239, "data[5]"=w2215, "data[6]"=w2238, "data[7]"=w2237, "Boolean"=w2235, "Count per volt"=w2077, "Boolean 2"=w2236, "Boolean 3"=w2248, "Numeric 10"=w2254, "Numeric 9"=w2253, "Numeric 11"=w2255, "Numeric 7"=w2251, "Numeric 12"=w2256) -> ("Numeric 5"=w2131:dbl, "Numeric 4"=w2130:dbl, "Numeric 6"=w2132:dbl, "Numeric 3"=w2129:dbl, "Numeric 2"=w2128:dbl, "Numeric"=w2127:dbl)  [unwired: 6 in]
        "TAP 3_4" <- w2129
        "TAP 3_5" <- w2128
        "TAP 3_6" <- w2127
        "TAP 3_1" <- w2132
        "TAP 3_2" <- w2131
        "TAP 3_3" <- w2130
        n816 = feedback-in #25(w2130) -> ()
        n817 = feedback-in #26(w2132) -> ()
        n818 = feedback-in #27(w2131) -> ()
        n819 = feedback-in #28(w2129) -> ()
        n820 = feedback-in #29(w2128) -> ()
        n821 = feedback-in #30(w2127) -> ()
        n822 = feedback #31() -> (w2245:dbl)
        n823 = feedback #32() -> (w2246:dbl)
        n824 = feedback #33() -> (w2247:dbl)
        n825 = feedback #34() -> (w2242:dbl)
        n826 = feedback #35() -> (w2241:dbl)
        n827 = feedback #36() -> (w2243:dbl)
        n828 = call "CAP-5.vi"("data[2]"=w2084, "data[3]"=w2083, "Numeric 9"=w2243, "Count per volt"=w2077, "data[4]"=w2239, "data[5]"=w2215, "data[6]"=w2238, "Boolean"=w2235, "data[7]"=w2237, "Boolean 2"=w2236, "Boolean 3"=w2240, "Numeric 12"=w2247, "Numeric 8"=w2242, "Numeric 11"=w2246, "Numeric 7"=w2241, "Numeric 10"=w2245) -> ("Numeric 5"=w2108:dbl, "Numeric 4"=w2107:dbl, "Numeric 6"=w2199:dbl, "Numeric 3"=w2106:dbl, "Numeric 2"=w2105:dbl, "Numeric"=w2104:dbl)  [unwired: 6 in]
        "TAP 4_1" <- w2108
        "TAP 4_2" <- w2107
        "TAP 4_3" <- w2199
        "TAP 4_" <- w2106
        "TAP 20" <- w2105
        "TAP 19" <- w2104
        n829 = feedback-in #31(w2108) -> ()
        n830 = feedback-in #32(w2107) -> ()
        n831 = feedback-in #33(w2199) -> ()
        n832 = feedback-in #34(w2106) -> ()
        n833 = feedback-in #35(w2105) -> ()
        n834 = feedback-in #36(w2104) -> ()
        n835 = feedback #37() -> (w2223:dbl)
        n836 = feedback #38() -> (w2222:dbl)
        n837 = feedback #39() -> (w2221:dbl)
        n838 = feedback #40() -> (w2226:dbl)
        n839 = feedback #41() -> (w2225:dbl)
        n840 = feedback #42() -> (w2224:dbl)
        n841 = call "CAP-MOD-5.vi"("data[2]"=w2084, "data[3]"=w2083, "Numeric 10"=w2224, "data[4]"=w2239, "data[5]"=w2215, "data[6]"=w2238, "data[7]"=w2237, "Boolean 2"=w2235, "Count per volt"=w2077, "Boolean 3"=w2236, "Boolean"=w2220, "Numeric 9"=w2223, "Numeric 12"=w2226, "Numeric 8"=w2222, "Numeric 11"=w2225, "Numeric 7"=w2221) -> ("Numeric 6"=w2198:dbl, "Numeric 5"=w2197:dbl, "Numeric 4"=w2196:dbl, "Numeric 3"=w2195:dbl, "Numeric 2"=w2194:dbl, "Numeric"=w2193:dbl)  [unwired: 6 in]
        "TAP 18" <- w2198
        "TAP 17" <- w2197
        "TAP 16" <- w2196
        "TAP 15" <- w2195
        "TAP 14" <- w2194
        "TAP 13" <- w2193
        n842 = feedback-in #37(w2198) -> ()
        n843 = feedback-in #38(w2197) -> ()
        n844 = feedback-in #39(w2196) -> ()
        n845 = feedback-in #40(w2195) -> ()
        n846 = feedback-in #41(w2194) -> ()
        n847 = feedback-in #42(w2193) -> ()
        n848 = feedback #43() -> (w2229:dbl)
        n849 = feedback #44() -> (w2228:dbl)
        n850 = feedback #45() -> (w2227:dbl)
        n851 = feedback #46() -> (w2232:dbl)
        n852 = feedback #47() -> (w2231:dbl)
        n853 = feedback #48() -> (w2230:dbl)
        n854 = call "CAP-MOD-6.vi"("data[2]"=w2084, "data[3]"=w2083, "Numeric 10"=w2230, "data[4]"=w2239, "data[5]"=w2215, "Count per volt"=w2077, "data[6]"=w2238, "Boolean 2"=w2235, "data[7]"=w2237, "Boolean 3"=w2236, "Boolean"=w2219, "Numeric 7"=w2227, "Numeric 12"=w2232, "Numeric 8"=w2228, "Numeric 11"=w2231, "Numeric 9"=w2229) -> ("Numeric 6"=w2192:dbl, "Numeric 5"=w2191:dbl, "Numeric 4"=w2190:dbl, "Numeric 3"=w2189:dbl, "Numeric 2"=w2188:dbl, "Numeric"=w2187:dbl)  [unwired: 6 in]
        "TAP 12" <- w2192
        "TAP 11" <- w2191
        "TAP 10" <- w2190
        "TAP 9" <- w2189
        "TAP 8" <- w2188
        "TAP 7" <- w2187
        n855 = feedback-in #43(w2192) -> ()
        n856 = feedback-in #44(w2191) -> ()
        n857 = feedback-in #45(w2190) -> ()
        n858 = feedback-in #46(w2189) -> ()
        n859 = feedback-in #47(w2188) -> ()
        n860 = feedback-in #48(w2187) -> ()
        n861 = case shown="1, Default" w2085 {
          tunnel: w2082 -> [w2403 w2414 w2425 w2436 w2447 w2458]
          tunnel: w2215 -> [w2402 w2413 w2424 w2435 w2446 w2457]
          tunnel: [w2401 w2415 w2427 w2437 w2451 w2463] -> w2214
          tunnel: w2213 -> [w2400 w2415 w2427 w2437 w2451 w2463]
          tunnel: [w2399 w2412 w2426 w2438 w2450 w2462] -> w2209
          tunnel: w2208 -> [w2399 w2411 w2426 w2438 w2450 w2462]
          tunnel: [w2398 w2410 w2423 w2439 w2449 w2461] -> w2206
          tunnel: w2207 -> [w2398 w2410 w2422 w2439 w2449 w2461]
          tunnel: [w2397 w2409 w2421 w2434 w2448 w2460] -> w2204
          tunnel: w2205 -> [w2397 w2409 w2421 w2433 w2448 w2460]
          tunnel: [w2396 w2408 w2420 w2432 w2445 w2459] -> w2203
          tunnel: w2202 -> [w2396 w2408 w2420 w2432 w2444 w2459]
          tunnel: [w2395 w2407 w2419 w2431 w2443 w2456] -> w2201
          tunnel: w2200 -> [w2395 w2407 w2419 w2431 w2443 w2455]
          frame 1, Default {
            n862 = case shown="True" w2403 {
              tunnel: w2402 -> [_ w2406]
              tunnel: [w2404 w2405] -> w2401
              tunnel: w2400 -> [w2404 _]
              frame False {
              }
              frame True {
                n863 = To Double Precision Float(number=w2406) -> (double precision float=w2405:dbl)
              }
            }
          }
          frame 2 {
            n864 = case shown="True" w2414 {
              tunnel: w2413 -> [_ w2418]
              tunnel: [w2416 w2417] -> w2412
              tunnel: w2411 -> [w2416 _]
              frame False {
              }
              frame True {
                n865 = To Double Precision Float(number=w2418) -> (double precision float=w2417:dbl)
              }
            }
          }
          frame 3 {
            n866 = case shown="True" w2425 {
              tunnel: w2424 -> [_ w2430]
              tunnel: [w2428 w2429] -> w2423
              tunnel: w2422 -> [w2428 _]
              frame False {
              }
              frame True {
                n867 = To Double Precision Float(number=w2430) -> (double precision float=w2429:dbl)
              }
            }
          }
          frame 4 {
            n868 = case shown="True" w2436 {
              tunnel: w2435 -> [_ w2442]
              tunnel: [w2440 w2441] -> w2434
              tunnel: w2433 -> [w2440 _]
              frame False {
              }
              frame True {
                n869 = To Double Precision Float(number=w2442) -> (double precision float=w2441:dbl)
              }
            }
          }
          frame 5 {
            n870 = case shown="True" w2447 {
              tunnel: w2446 -> [_ w2454]
              tunnel: [w2452 w2453] -> w2445
              tunnel: w2444 -> [w2452 _]
              frame False {
              }
              frame True {
                n871 = To Double Precision Float(number=w2454) -> (double precision float=w2453:dbl)
              }
            }
          }
          frame 6 {
            n872 = case shown="False" w2458 {
              tunnel: w2457 -> [_ w2466]
              tunnel: [w2464 w2465] -> w2456
              tunnel: w2455 -> [w2464 _]
              frame False {
              }
              frame True {
                n873 = To Double Precision Float(number=w2466) -> (double precision float=w2465:dbl)
              }
            }
          }
        }
        "Temp_1" <- w2214
        "Temp_2" <- w2209
        "Temp_3" <- w2206
        "Temp_4" <- w2204
        "Temp_5" <- w2203
        "Temp_6" <- w2201
        n874 = Build Array(w2180, w2178, w2177, w2176, w2175, w2174, w2156, w2155, w2154, w2153, w2152, w2151, w2132, w2131, w2130, w2129, w2128, w2127, w2108, w2107, w2199, w2106, w2105, w2104, w2198, w2197, w2196, w2195, w2194, w2193, w2192, w2191, w2190, w2189, w2188, w2187) -> (w2186:dbl[])
        n875 = call "Elapsed Time"("Time Target (s)"=w2183, "Auto Reset"=TRUE) -> ()  [unwired: 10 in, 8 out]
        n876 = Add(x=w2183, y=w2181) -> (x+y=w2182:dbl)
        n877 = Array To Cluster(array=w2186) -> ()  [unwired: 1 out]
        n878 = case shown="5" w2085 {
          tunnel: w2084 -> [w2294 w2316 w2338 w2360 w2382]
          tunnel: w2083 -> [w2293 w2315 w2337 w2359 w2381]
          tunnel: w2082 -> [w2292 w2314 w2336 w2358 w2380]
          tunnel: w2081 -> [w2291 w2313 w2335 w2357 w2379]
          tunnel: [w2290 w2313 w2335 w2357 w2379] -> w2064
          tunnel: [w2289 w2312 w2334 w2356 w2378] -> w2063
          tunnel: w2080 -> [w2289 w2311 w2334 w2356 w2378]
          tunnel: [w2288 w2310 w2333 w2355 w2377] -> w2062
          tunnel: w2079 -> [w2288 w2310 w2332 w2355 w2377]
          tunnel: [w2287 w2309 w2331 w2354 w2373] -> w2061
          tunnel: w2078 -> [w2287 w2309 w2331 w2353 w2373]
          tunnel: w2077 -> [w2286 w2308 w2330 w2352 w2376]
          tunnel: [w2285 w2307 w2329 w2351 w2375] -> w2060
          tunnel: w2076 -> [w2285 w2307 w2329 w2351 w2374]
          frame 1, Default {
            n879 = case shown="True" w2292 {
              tunnel: [w2295 w2299] -> w2290
              tunnel: w2294 -> [_ w2298]
              tunnel: w2293 -> [_ w2297]
              tunnel: w2291 -> [w2295 _]
              tunnel: w2286 -> [_ w2296]
              frame False {
              }
              frame True {
                n880 = To Double Precision Float(number=w2298) -> (double precision float=w2301:dbl)
                n881 = To Double Precision Float(number=w2297) -> (double precision float=w2300:dbl)
                n882 = Multiply(x=w2300, y=255.0) -> (x*y=w2303:dbl)
                n883 = Add(x=w2301, y=w2303) -> (x+y=w2305:dbl)
                n884 = Multiply(x=w2305, y=w2296) -> (x*y=w2304:dbl)
                n885 = Divide(x=w2304, y=1000.0) -> (x/y=w2299:dbl)
              }
            }
          }
          frame 2 {
            n886 = case shown="True" w2314 {
              tunnel: [w2317 w2321] -> w2312
              tunnel: w2316 -> [_ w2320]
              tunnel: w2315 -> [_ w2319]
              tunnel: w2311 -> [w2317 _]
              tunnel: w2308 -> [_ w2318]
              frame False {
              }
              frame True {
                n887 = To Double Precision Float(number=w2320) -> (double precision float=w2323:dbl)
                n888 = To Double Precision Float(number=w2319) -> (double precision float=w2322:dbl)
                n889 = Multiply(x=w2322, y=255.0) -> (x*y=w2325:dbl)
                n890 = Add(x=w2323, y=w2325) -> (x+y=w2327:dbl)
                n891 = Multiply(x=w2327, y=w2318) -> (x*y=w2326:dbl)
                n892 = Divide(x=w2326, y=1000.0) -> (x/y=w2321:dbl)
              }
            }
          }
          frame 3 {
            n893 = case shown="True" w2336 {
              tunnel: w2338 -> [_ w2343]
              tunnel: w2337 -> [_ w2342]
              tunnel: [w2339 w2341] -> w2333
              tunnel: w2332 -> [w2339 _]
              tunnel: w2330 -> [_ w2340]
              frame False {
              }
              frame True {
                n894 = To Double Precision Float(number=w2343) -> (double precision float=w2345:dbl)
                n895 = To Double Precision Float(number=w2342) -> (double precision float=w2344:dbl)
                n896 = Multiply(x=w2344, y=255.0) -> (x*y=w2347:dbl)
                n897 = Add(x=w2345, y=w2347) -> (x+y=w2349:dbl)
                n898 = Multiply(x=w2349, y=w2340) -> (x*y=w2348:dbl)
                n899 = Divide(x=w2348, y=1000.0) -> (x/y=w2341:dbl)
              }
            }
          }
          frame 4 {
            n900 = case shown="True" w2358 {
              tunnel: w2360 -> [_ w2365]
              tunnel: w2359 -> [_ w2364]
              tunnel: [w2361 w2363] -> w2354
              tunnel: w2353 -> [w2361 _]
              tunnel: w2352 -> [_ w2362]
              frame False {
              }
              frame True {
                n901 = To Double Precision Float(number=w2365) -> (double precision float=w2367:dbl)
                n902 = To Double Precision Float(number=w2364) -> (double precision float=w2366:dbl)
                n903 = Multiply(x=w2366, y=255.0) -> (x*y=w2369:dbl)
                n904 = Add(x=w2367, y=w2369) -> (x+y=w2371:dbl)
                n905 = Multiply(x=w2371, y=w2362) -> (x*y=w2370:dbl)
                n906 = Divide(x=w2370, y=1000.0) -> (x/y=w2363:dbl)
              }
            }
          }
          frame 5 {
            n907 = case shown="True" w2380 {
              tunnel: w2382 -> [_ w2387]
              tunnel: w2381 -> [_ w2386]
              tunnel: w2376 -> [_ w2385]
              tunnel: [w2383 w2384] -> w2375
              tunnel: w2374 -> [w2383 _]
              frame False {
              }
              frame True {
                n908 = To Double Precision Float(number=w2387) -> (double precision float=w2389:dbl)
                n909 = To Double Precision Float(number=w2386) -> (double precision float=w2388:dbl)
                n910 = Multiply(x=w2388, y=255.0) -> (x*y=w2391:dbl)
                n911 = Add(x=w2389, y=w2391) -> (x+y=w2393:dbl)
                n912 = Multiply(x=w2393, y=w2385) -> (x*y=w2392:dbl)
                n913 = Divide(x=w2392, y=1000.0) -> (x/y=w2384:dbl)
              }
            }
          }
        }
        "VOLT-CAP-1" <- w2064
        "VOLT-CAP-2" <- w2063
        "VOLT-CAP-3" <- w2062
        "VOLT-CAP-4" <- w2061
        "VOLT-CAP-5" <- w2060
        "Vertical Progress Bar 2" <- w2063
        "Vertical Progress Bar 5" <- w2060
        "Vertical Progress Bar 4" <- w2061
        "Vertical Progress Bar 3" <- w2062
        "Vertical Progress Bar" <- w2064
        n914 = Build Array (concatenate)(w2126, w2127) -> (w2120:dbl[])
        n915 = Build Array (concatenate)(w2125, w2128) -> (w2119:dbl[])
        n916 = Build Array (concatenate)(w2124, w2129) -> (w2118:dbl[])
        n917 = Build Array (concatenate)(w2123, w2130) -> (w2117:dbl[])
        n918 = Build Array (concatenate)(w2185, w2181) -> (w2059:dbl[])
        n919 = Build Array (concatenate)(w2122, w2131) -> (w2116:dbl[])
        n920 = Build Array (concatenate)(w2121, w2132) -> (w2115:dbl[])
        n921 = Build Array (concatenate)(w2179, w2180) -> (w2162:dbl[])
        n922 = Build Array (concatenate)(w2173, w2178) -> (w2161:dbl[])
        n923 = Build Array (concatenate)(w2172, w2177) -> (w2160:dbl[])
        n924 = Build Array (concatenate)(w2171, w2176) -> (w2159:dbl[])
        n925 = Build Array (concatenate)(w2144, w2156) -> (w2138:dbl[])
        n926 = Build Array (concatenate)(w2143, w2155) -> (w2137:dbl[])
        n927 = Build Array (concatenate)(w2170, w2175) -> (w2158:dbl[])
        n928 = Build Array (concatenate)(w2169, w2174) -> (w2157:dbl[])
        n929 = Build Array (concatenate)(w2142, w2154) -> (w2136:dbl[])
        n930 = Build Array (concatenate)(w2141, w2153) -> (w2135:dbl[])
        n931 = Build Array (concatenate)(w2140, w2152) -> (w2134:dbl[])
        n932 = Build Array (concatenate)(w2139, w2151) -> (w2133:dbl[])
        n933 = Build Array (concatenate)(w2103, w2108) -> (w2091:dbl[])
        n934 = Build Array (concatenate)(w2102, w2107) -> (w2090:dbl[])
        n935 = Build Array (concatenate)(w2101, w2106) -> (w2089:dbl[])
        n936 = Build Array (concatenate)(w2100, w2105) -> (w2088:dbl[])
        n937 = Build Array (concatenate)(w2099, w2104) -> (w2087:dbl[])
        n938 = Build Array (concatenate)(w2098, w2104) -> (w2086:dbl[])
        n939 = Bundle(w2059, w2120) -> (w2114:cluster{dbl[], dbl[]})  [unwired: 1 in]
        n940 = Bundle(w2059, w2119) -> (w2113:cluster{dbl[], dbl[]})  [unwired: 1 in]
        n941 = Bundle(w2059, w2118) -> (w2112:cluster{dbl[], dbl[]})  [unwired: 1 in]
        n942 = Bundle(w2059, w2117) -> (w2111:cluster{dbl[], dbl[]})  [unwired: 1 in]
        n943 = Bundle(w2059, w2116) -> (w2110:cluster{dbl[], dbl[]})  [unwired: 1 in]
        n944 = Bundle(w2059, w2115) -> (w2109:cluster{dbl[], dbl[]})  [unwired: 1 in]
        n945 = Bundle(w2059, w2162) -> (w2168:cluster{dbl[], dbl[]})  [unwired: 1 in]
        n946 = Bundle(w2059, w2161) -> (w2167:cluster{dbl[], dbl[]})  [unwired: 1 in]
        n947 = Bundle(w2059, w2160) -> (w2166:cluster{dbl[], dbl[]})  [unwired: 1 in]
        n948 = Bundle(w2059, w2159) -> (w2165:cluster{dbl[], dbl[]})  [unwired: 1 in]
        n949 = Bundle(w2059, w2138) -> (w2150:cluster{dbl[], dbl[]})  [unwired: 1 in]
        n950 = Bundle(w2059, w2137) -> (w2149:cluster{dbl[], dbl[]})  [unwired: 1 in]
        n951 = Bundle(w2059, w2158) -> (w2164:cluster{dbl[], dbl[]})  [unwired: 1 in]
        n952 = Bundle(w2059, w2157) -> (w2163:cluster{dbl[], dbl[]})  [unwired: 1 in]
        n953 = Bundle(w2059, w2136) -> (w2148:cluster{dbl[], dbl[]})  [unwired: 1 in]
        n954 = Bundle(w2059, w2135) -> (w2147:cluster{dbl[], dbl[]})  [unwired: 1 in]
        n955 = Bundle(w2059, w2134) -> (w2146:cluster{dbl[], dbl[]})  [unwired: 1 in]
        n956 = Bundle(w2059, w2133) -> (w2145:cluster{dbl[], dbl[]})  [unwired: 1 in]
        n957 = Bundle(w2059, w2091) -> (w2097:cluster{dbl[], dbl[]})  [unwired: 1 in]
        n958 = Bundle(w2059, w2090) -> (w2096:cluster{dbl[], dbl[]})  [unwired: 1 in]
        n959 = Bundle(w2059, w2089) -> (w2095:cluster{dbl[], dbl[]})  [unwired: 1 in]
        n960 = Bundle(w2059, w2088) -> (w2094:cluster{dbl[], dbl[]})  [unwired: 1 in]
        n961 = Bundle(w2059, w2087) -> (w2093:cluster{dbl[], dbl[]})  [unwired: 1 in]
        n962 = Bundle(w2059, w2086) -> (w2092:cluster{dbl[], dbl[]})  [unwired: 1 in]
        n963 = Build Array (concatenate)(w2070, w2064) -> (w2069:dbl[])
        n964 = Build Array (concatenate)(w2068, w2063) -> (w2054:dbl[])
        n965 = Build Array (concatenate)(w2066, w2061) -> (w2052:dbl[])
        n966 = Build Array (concatenate)(w2065, w2060) -> (w2051:dbl[])
        n967 = Build Array (concatenate)(w2067, w2062) -> (w2053:dbl[])
        n968 = Bundle(w2059, w2069) -> (w2072:cluster{dbl[], dbl[]})  [unwired: 1 in]
        n969 = Bundle(w2059, w2054) -> (w2058:cluster{dbl[], dbl[]})  [unwired: 1 in]
        n970 = Bundle(w2059, w2053) -> (w2057:cluster{dbl[], dbl[]})  [unwired: 1 in]
        n971 = Bundle(w2059, w2052) -> (w2056:cluster{dbl[], dbl[]})  [unwired: 1 in]
        n972 = Bundle(w2059, w2051) -> (w2055:cluster{dbl[], dbl[]})  [unwired: 1 in]
        n973 = Build Array(w2168, w2167, w2166, w2165, w2164, w2163, w2150, w2149, w2148, w2147, w2146, w2145, w2114, w2113, w2112, w2111, w2110, w2109, w2097, w2096, w2095, w2094, w2093, w2092) -> (→"TAP Voltages":cluster{dbl[], dbl[]}[])
        n974 = Build Array(w2072, w2058, w2057, w2056, w2055) -> (→"Full Voltage":cluster{dbl[], dbl[]}[])
        n975 = node-c288() -> ()  [unwired: 1 in, 1 out]
      }
      n976 = VISA Close(VISA resource name=w140, error in (no error)=w139) -> ()  [unwired: 1 out]
      n977 = call-dynamic "Close.vi"("error in (no error)"=w43, "Modbus master in"=w44) -> ("error out"=→"error out 3":errorcluster)  [unwired: 9 in]
      n978 = call-dynamic "Close.vi"("error in (no error)"=w84, "Modbus master in"=w87) -> ("error out"=→"error out":errorcluster)  [unwired: 9 in]
      n979 = call-dynamic "Close.vi"("error in (no error)"=w46, "Modbus master in"=w45) -> ("error out"=→"error out 2":errorcluster)  [unwired: 9 in]
      n980 = call <vilib>:"CloseHandle.vi"("client handle"=w129, "error in (no error)"=w128) -> ()  [unwired: 13 in, 1 out]
      n981 = call <vilib>:"CloseHandle.vi"("client handle"=w127, "error in (no error)"=w126) -> ()  [unwired: 13 in, 1 out]
      n982 = node-c288(w169) -> ()  [unwired: 1 out]
    }
  }
